vi "myRIO_BRig_RT_v0,50.vi"() -> ()   [LabVIEW 2014]
uses:
  myRIO_BRig_RT__Case_Exp_stateList.ctl
  myRIO_BRig_RT__Case_NonExp_stateList.ctl
  <vilib>/Platform/TimedLoop/XDataNode/timing_clust.ctl
  <vilib>/Platform/TimedLoop/XDataNode/nitl_modes.ctl
  <vilib>/Platform/TimedLoop/XDataNode/wakeup.ctl
  <vilib>/WebDAVClient/Advanced/SessionHandle.ctl
  <vilib>/myRIO/Common/Instrument Driver Framework/myRIO v1.0/UART/vis/myRIO v1.0 Close UART.vi
  <vilib>/FPGAPlugInAG/myRIO-1900/niLvFpga_Open_myRIO-1900.vi
  <vilib>/rvi/interface/common/dynamic/niFpgaDynamicAddResources.vi
  <vilib>/Utility/error.llb/Error Cluster From Error Code.vi
  <vilib>/rvi/errors/niLvFpgaAdjustHostInterfaceError.vi
  <vilib>/FPGAPlugInAG/Dynamic/niLvFpga_Close_Dynamic.vi
  <vilib>/myRIO/Common/Instrument Driver Framework/Utilities/vis/FPGA Ref Manager.vi
  <vilib>/myRIO/Common/Instrument Driver Framework/myRIO v1.0/myRIO v1.0 Reset FPGA.vi
  <vilib>/myRIO/Common/Instrument Driver Framework/myRIO v1.0/IRQ/vis/myRIO v1.0 IRQ Info FGV.vi
  <vilib>/myRIO/Common/Instrument Driver Framework/myRIO v1.0/IRQ/vis/myRIO v1.0 Timer IRQ Info FGV.vi
  <vilib>/myRIO/Common/Instrument Driver Framework/myRIO v1.0/IRQ/vis/myRIO v1.0 ISR Agent.vi
  <vilib>/rvi/interface/nirviOpenFPGA/nirviOpenFPGA.xnode
  myRIO_BRig_FPGA_v3,40__build.lvbitx
  myRIO_BRig_FPGA_v3,40.vi
  <vilib>/rvi/interface/nirviReadWriteControl/nirviReadWriteControl.xnode
  <vilib>/Platform/TimedLoop/XDataNode/XDataNode.xnode
  <vilib>/rvi/interface/nirviCloseFPGA/nirviCloseFPGA.xnode
  <vilib>/Platform/TimedLoop/XDataNode/XDNodeRunTimeDep.lvlib
  <vilib>/rvi/interface/Simulation/niFpgaSimulationCallBeginRW.vi
  <vilib>/myRIO/Instrument Drivers/Utilities/Utilities.lvlib
  <vilib>/WebDAVClient/NI_WebDAV.lvlib
  NiFpgaLv.dll
panel:
  in  "laser_power":dbl
  in  "f_millisec2count":dbl=109.0
  in  "laser_Tshutter":dbl=2.0
  in  "laser_Freq":dbl=10.0
  in  "laser_Tpeak":dbl=2.0
  in  "laser_duration":u16
  out "error out":errorcluster
  in  "LC_Cue1_All_Count":u16
  in  "LC_Cue1_First_Count":u16
  in  "LC_Cue1_All_delayOpt":bool
  in  "LC_ENL1_All_delayOpt":bool
  in  "LC_ENL1_All_Count":u16
  in  "LC_ENL1_First_Count":u16
  in  "LC_Cue1_First_delayOpt":bool
  in  "LC_ENL1_First_delayOpt":bool
  in  "Tcycle_Cue_max":u16=1000 caption="Max [ms]" min=5 max=5000 step=5
  in  "Tcycle_Cue_min":u16=1000 caption="Min [ms]" min=5 max=5000 step=5
  in  "SendData":bool
  out "cSpout":enum16{"Left", "Right"}(ring) caption="Left or Right Spout"
  out "A4":u32 caption="LickCounter_Right"
  out "A2":u32 caption="LickCounter_Left"
  in  "tDelay_laser_wro":u32
  in  "tCycle_laser_wro":u32=1000
  in  "tDelay_laser_rew":u32
  in  "laserResponse_wrong_LED":bool
  out "error_initTrial":errorcluster
  out "error_Selection_pre":errorcluster
  out "error_Selection":errorcluster
  in  "tCycle_laser_rew":u32=1000
  out "SelectWrong":bool
  out "SelectReward":bool
  in  "Left(F)_or_Right(T)":bool
  in  "ignoreWrong":bool
  in  "SelectionState":bool
  in  "laserResponse_wrong":bool
  in  "laserResponse_reward":bool
  in  "laserResponse_reward_LED":bool
  out "nRewards_Right":u16 caption="# Rewards Total (Right)"
  out "nRewards_Left":u16 caption="# Rewards Total (Left)"
  out "nRewards_cur":u16 caption="# Rewards in Current Block"
  out "TpB_target":u16 caption="Target Trials Per Block"
  out "cState_NonExp":T1 caption="NonExperimental State"
  out "iBlock":u16 caption="Current Block"
  out "cState":T2 caption="Experimental State"
  out "iTrial":u16 caption="Current Trial"
  in  "warmupType":bool
  in  "TestConnection":bool
  in  "warmup":bool caption="WarmUp"
  in  "Host Filename Prefix":string="Exp1_TM2"
  out "Connected To Host?":bool
  in  "Host Password":string="sabalab"
  in  "Host UserName":string="Test2"
  in  "sp_RightSpout":u16(slide)=2 max=2 step=1 scale=0.0..2.0
  in  "sp_LeftSpout":u16(slide)=2 max=2 step=1 scale=0.0..2.0
  in  "BUR_max":u16 caption="Count Reward Structure  (0 = off)"
  in  "LC_Wrong_Probability":u16
  in  "LC_Wrong_Trial":u16(slide) max=2 step=1 scale=0.0..2.0
  in  "LC_Wrong_Block":u16(slide) max=2 step=1 scale=0.0..2.0
  in  "LC_Wrong_OnOff":bool
  in  "LC_Reward_Probability":u16
  in  "LC_Reward_Trial":u16(slide) max=2 step=1 scale=0.0..2.0
  in  "LC_Reward_Block":u16(slide) max=2 step=1 scale=0.0..2.0
  in  "LC_Reward_OnOff":bool
  in  "LC_Cue1_All_Probability":u16
  in  "LC_Cue1_All_Block":u16(slide) max=2 step=1 scale=0.0..2.0
  in  "LC_Cue1_All_OnOff":bool
  in  "LC_Cue1_First_Probability":u16
  in  "LC_Cue1_First_Block":u16(slide) max=2 step=1 scale=0.0..2.0
  in  "LC_Cue1_First_OnOff":bool
  in  "LC_ENL1_All_Probability":u16 max=100 step=1
  in  "LC_ENL1_All_Block":u16(slide) max=2 step=1 scale=0.0..2.0
  in  "LC_ENL1_All_OnOff":bool
  in  "LC_ENL1_First_Probability":u16 max=100 step=1
  in  "LC_ENL1_First_Block":u16(slide) max=2 step=1 scale=0.0..2.0
  in  "Tcycle_Timeout":u16=1000 caption="Timeout Time [ms]" min=10 max=10000 step=1
  in  "Tcycle_Wrong":u16=1000 caption="Wrong Time [ms]" min=10 max=10000 step=1
  in  "Tcycle_Selection":u16=1000 caption="Answer Time [ms]" min=1 max=10000 step=1
  in  "Tcycle_RewardPost":u16=1000 caption="Consumption Time [ms]" min=250 max=10000 step=250
  in  "Tcycle_Reward_L":u16=500 caption="Reward Time [ms]" min=1 max=1000 step=1
  in  "Tcycle_Reward_R":u16=500 caption="Reward Time [ms]" min=1 max=1000 step=1
  in  "TpB_Max_R":u16=4 caption="Max TrialsPerBlock" min=1 max=12 step=1
  in  "TpB_Min_R":u16=4 caption="Min TrialsPerBlock" min=1 max=12 step=1
  in  "TpB_Max_L":u16=4 caption="Max TrialsPerBlock" min=1 max=12 step=1
  in  "TpB_Min_L":u16=4 caption="Min TrialsPerBlock" min=1 max=12 step=1
  in  "BUR_min":u16 caption="Count Reward Structure  (0 = off)"
  in  "TrialUntilReward":bool caption="Ignore Wrong \nSelection"
  in  "CueCycles":u16=1 caption="Cue Structure" min=1 max=1 step=1
  in  "MTrig_Laser_Tcycle":u16=10 caption="Time [ms]"
  in  "MTrig_Laser_trig":bool
  in  "MTrig_Audio_trig__R":bool caption="Trigger Audio"
  in  "MTrig_Audio_trig__L":bool caption="Trigger Audio"
  in  "RewCalib_Trig_R":bool caption="Calibrate_R"
  in  "RewCalib_Trig_L":bool caption="Calibrate_L"
  in  "MTrig_Solenoid_Tcycle__R":u16=300 caption="Time [ms]"
  in  "MTrig_Solenoid_Tcycle__L":u16=300 caption="Time [ms]"
  in  "MTrig_Solenoid_trig__R":bool caption="Solenoid"
  in  "MTrig_Solenoid_trig__L":bool caption="Solenoid"
  in  "STOP_abort":bool caption="Stop LabView\n(Stops myRio and FPGA)"
  in  "STOP_endBlock":bool caption="Stop Experiment\n@ End of Block"
  in  "STOP_endTrial":bool caption="Stop Experiment\n@ End of Trial"
  in  "START":bool caption="Start Experiment"
  in  "Tcycle_CuePenalty":u16=1000 caption="Penalty [ms]" min=1 max=10000 step=1
  in  "Audio_Amp__R":u16=100 caption="Amp"
  in  "Audio_Freq__R":u16=5 caption="Freq [kHz]" max=14 step=1
  in  "Audio_Amp__L":u16=100 caption="Amp"
  in  "Audio_Freq__L":u16=5 caption="Freq [kHz]" max=14 step=1
  in  "LC_Wrong_Tdelay":u16
  in  "LC_Cue1_All_Tdelay":u16
  in  "LC_ENL1_All_Tdelay":u16
  in  "LC_Reward_Tdelay":u16
  in  "LC_Cue1_First_Tdelay":u16
  in  "LC_ENL1_First_Tdelay":u16
  in  "LC_ENL1_First_OnOff":bool
  in  "Tcycle_ENLPenalty":u16=100 caption="Penalty [ms]" min=10 max=10000 step=10
  in  "Tcycle_ENL_max":u16=1000 caption="Max [ms]" min=250 max=10000 step=250
  in  "Tcycle_ENL_min":u16=1000 caption="Min [ms]" min=250 max=10000 step=250
  # "Manual Control"
  # "Task Structure"
  # "Task Timing"
  # "Laser Control\n\n                                                    On/Off      Block        Probability [%]   Delay [ms]                              Count"
  # "Manual Solenoid Trigger\nLeft              Right"
  # "Master Structure"
  # "Enforced NonLick"
  # "Enforced NonLick 1"
  # "from end"
  # "Time = Cue Min"
  # "Min\n \n  \nMax"
  # "First Trial"
  # "from start"
  # "(1) = Switching\n(2) = Two Choice"
  # "from end"
  # "All Trials"
  # "Cue"
  # "from start"
  # "Cue 1"
  # "from end"
  # "from start"
  # "Cue then reward"
  # "Min"
  # "Max"
  # "from end"
  # "Cue with reward"
  # "Trial Per Block Structure\n       Left                    Right"
  # "from start"
  # "Spout Selection Control"
  # "Manual Speaker Trigger\nLeft              Right"
  # "Selection Reward"
  # "Answer Time\n         [ms]\n\n  \nWrong Choice Penalty\n         [ms]\n \n \nChoice Timeout Penalty\n         [ms]"
  # "Selection Wrong"
  # "Cue Control"
  # "Left              Right"
  # "State"
  # "Manual Laser Trigger"
  # "Freq [kHz]\n \n \nAmp\n \n\n \n\nSpeaker\nSetting"
  # "Reward Control\n                 Left              Right"
  # "Min = 1\nMax = 32k"
  # "Reward Time\n         [ms]"
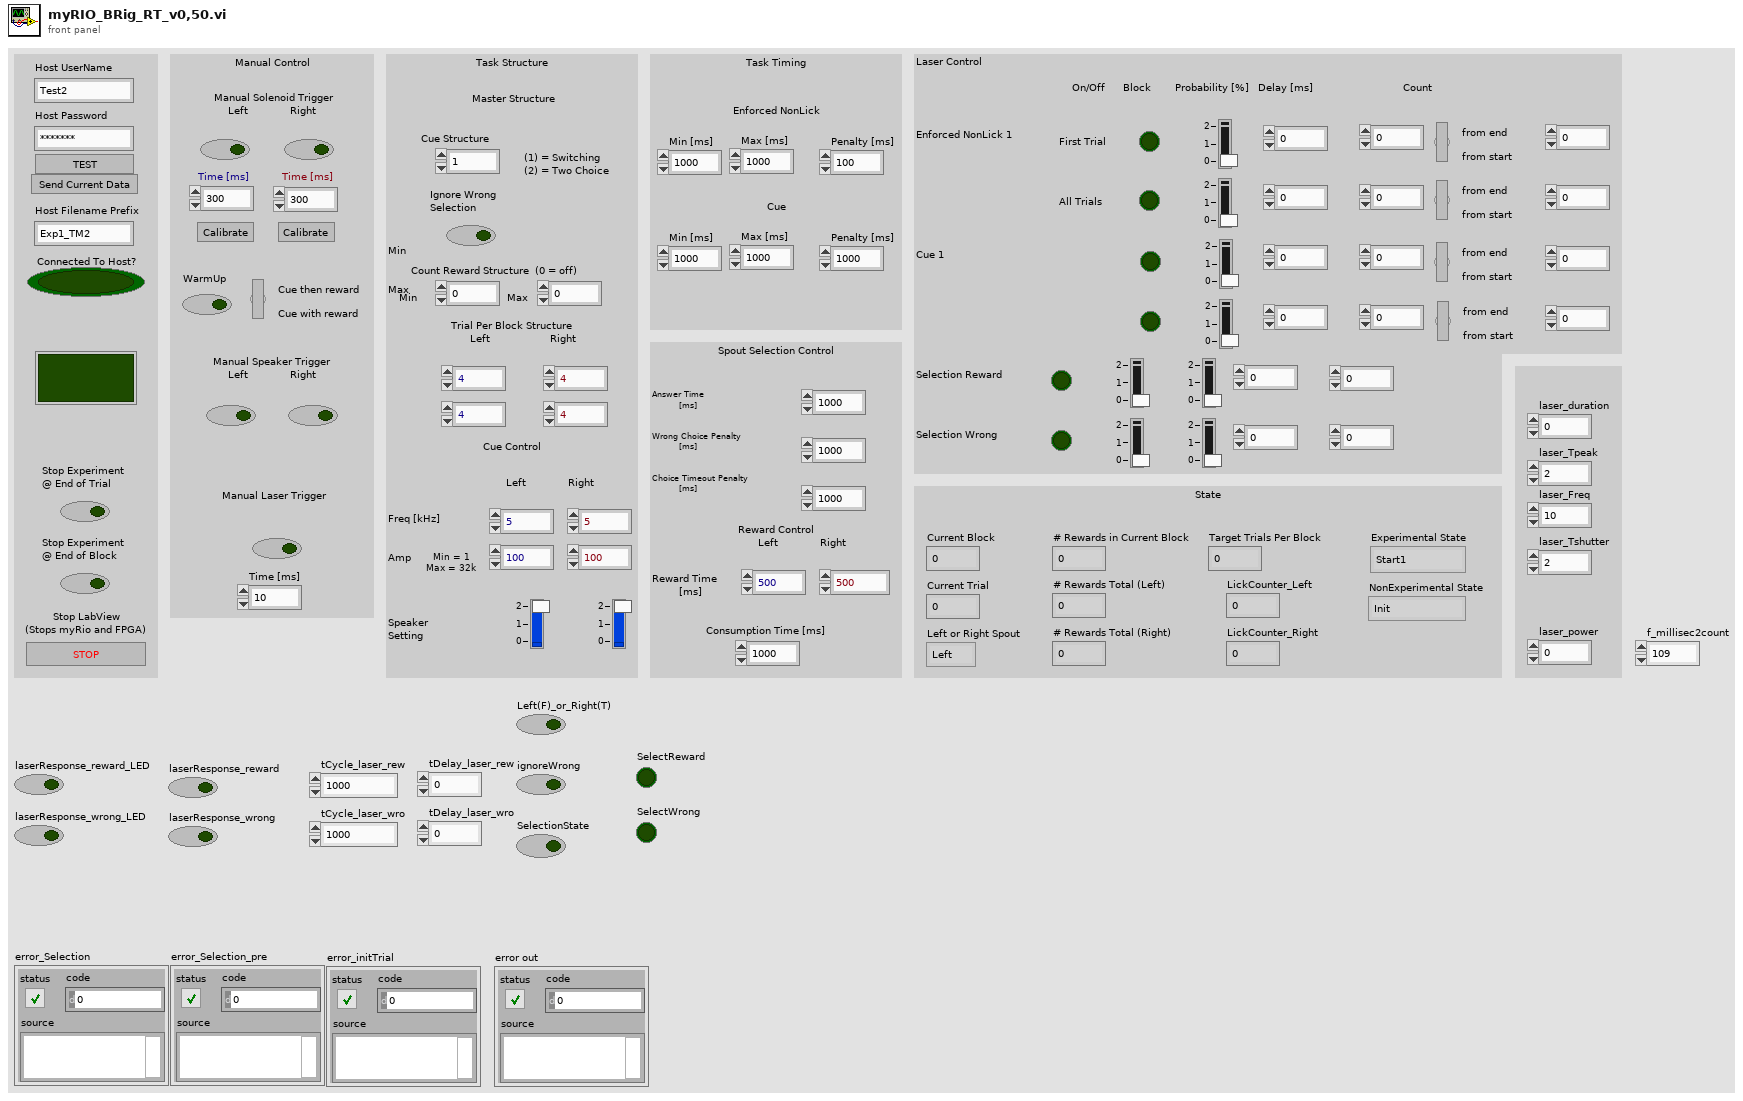
[diagram p1: front panel]
types:
  T1 = typedef "myRIO_BRig_RT__Case_NonExp_stateList.ctl" = enum16{"Init", "UploadSettings_pre", "UploadSettings_Read_dataExp", "UploadSettings_dataExp_1", "UploadSettings_Read_dataLC", "UploadSettings_dataLC_1", "UploadSettings_dataLC_2", "UploadSettings_Read_dataMTrig", "UploadSettings_dataMTrig_1", "UploadSettings_post", "Idle_pre", "IdleEmpty", "IdleEmpty2", "IdleEmpty3", "IdleEmpty4", "Idle", "Idle_2", "Idle_3", "Idle_4", "Idle_post", "Cue_pre__pre", "Cue_pre", "Cue", "Cue_post", "RewardCalibration_pre", "DispenseWater_pre__pre", "DispenseWater_pre", "DispenseWater", "DispenseWater_post", "TestConnection", "SendData", "End"}
  T2 = typedef "myRIO_BRig_RT__Case_Exp_stateList.ctl" = enum16{"Start1", "Start2", "Start3", "saveSettings1", "saveSettings2", "saveSettings3", "saveSettings4_LC_ENL", "saveSettings5_LC_Cue", "saveSettings6_LC_Other", "setSettings_Audio", "setSettings_Laser", "initBlock_pre", "initBlock", "initBlock2", "initBlock_post", "initTrial_pre", "initTrial", "initTrial2", "initTrial3", "initTrial4", "initTrial_LC_ENL1", "initTrial_LC_Cue1", "initTrial_post", "ENL1_pre", "ENL1", "ENL1_post", "ENL1Penalty_pre", "ENL1Penalty", "ENL2_pre", "ENL2", "ENL2Penalty_pre", "ENL2Penalty", "Cue1_pre", "Cue1", "Cue1_post", "Cue1Penalty_pre", "Cue1Penalty", "Cue2_pre", "Cue2", "Cue2Penalty_pre", "Cue2Penalty", "Selection_pre", "Selection", "Select_post", "SelectReward_pre", "SelectReward", "SelectRewardPost_pre", "SelectRewardPost", "SelectWrong_pre", "SelectWrong", "SelectWrong_post", "SelectTimeout_pre", "SelectTimeout", "SelectTimeout_post", "endTrial_pre", "endTrial1", "endTrial2", "endTrial3", "endTrial_post", "endBlock_pre", "endBlock", "endBlock_post", "endExp", "commConnect", "commUpload_pre", "commUpload_dataBlock", "commUpload_dataCurrent", "commUpload_dataExp", "commUpload_dataLC", "commUpload_dataTrial", "commUpload_post", "saveData_pre", "saveData_dataBlock", "saveData_dataCurrent", "saveData_dataExp", "saveData_dataLC", "saveData_dataTrial", "saveData_post", "empty_endBlock1", "empty_endBlock2", "empty_endTrial1", "empty_endTrial2", "empty_endTrial3", "empty_endTrial4", "empty_endTrial5"}
  T3 = typedef "XDNodeRunTimeDep.lvlib/timing_clust.ctl" = cluster{"Expected End [f-1]":u64, "Actual End [f-1]":u64, "Finished Late? [f-1]":bool, "Expected End [i-1]":u64, "Actual End [i-1]":u64, "Finished Late? [i-1]":bool, "Expected Start [i]":u64, "Actual Start [i]":u64, "Expected Start [f]":u64, "Actual Start [f]":u64, "Source Name":string, "Structure Name":string, "Period":i64, "Deadline":i64, "Offset":i64, "Start":i64, "Priority":i32, "Timeout":i32, "Mode":T4, "Wakeup Reason":T5, "Error":errorcluster, "Source Type":string, "Secondary Source Type":string, "Global End Time":u64, "Global Start Time":u64, "Frame Duration":u64, "Iteration Duration":u64, "Assigned CPU":i32, "I/O Scan Engine Mode":u32}
  T4 = typedef "XDNodeRunTimeDep.lvlib/nitl_modes.ctl" = enum32{"No Change", "Process missed periods, maintain original phase", "Discard missed periods, maintain original phase", "Process missed periods, ignore original phase", "Discard missed periods, ignore original phase"}
  T5 = typedef "XDNodeRunTimeDep.lvlib/wakeup.ctl" = enum32{"Normal", "Aborted", "Asynchronous wakeup", "Timing source error", "Timed loop error", "Timeout"}
  T6 = typedef "NI_WebDAV.lvlib/SessionHandle.ctl" = refnum<k1>
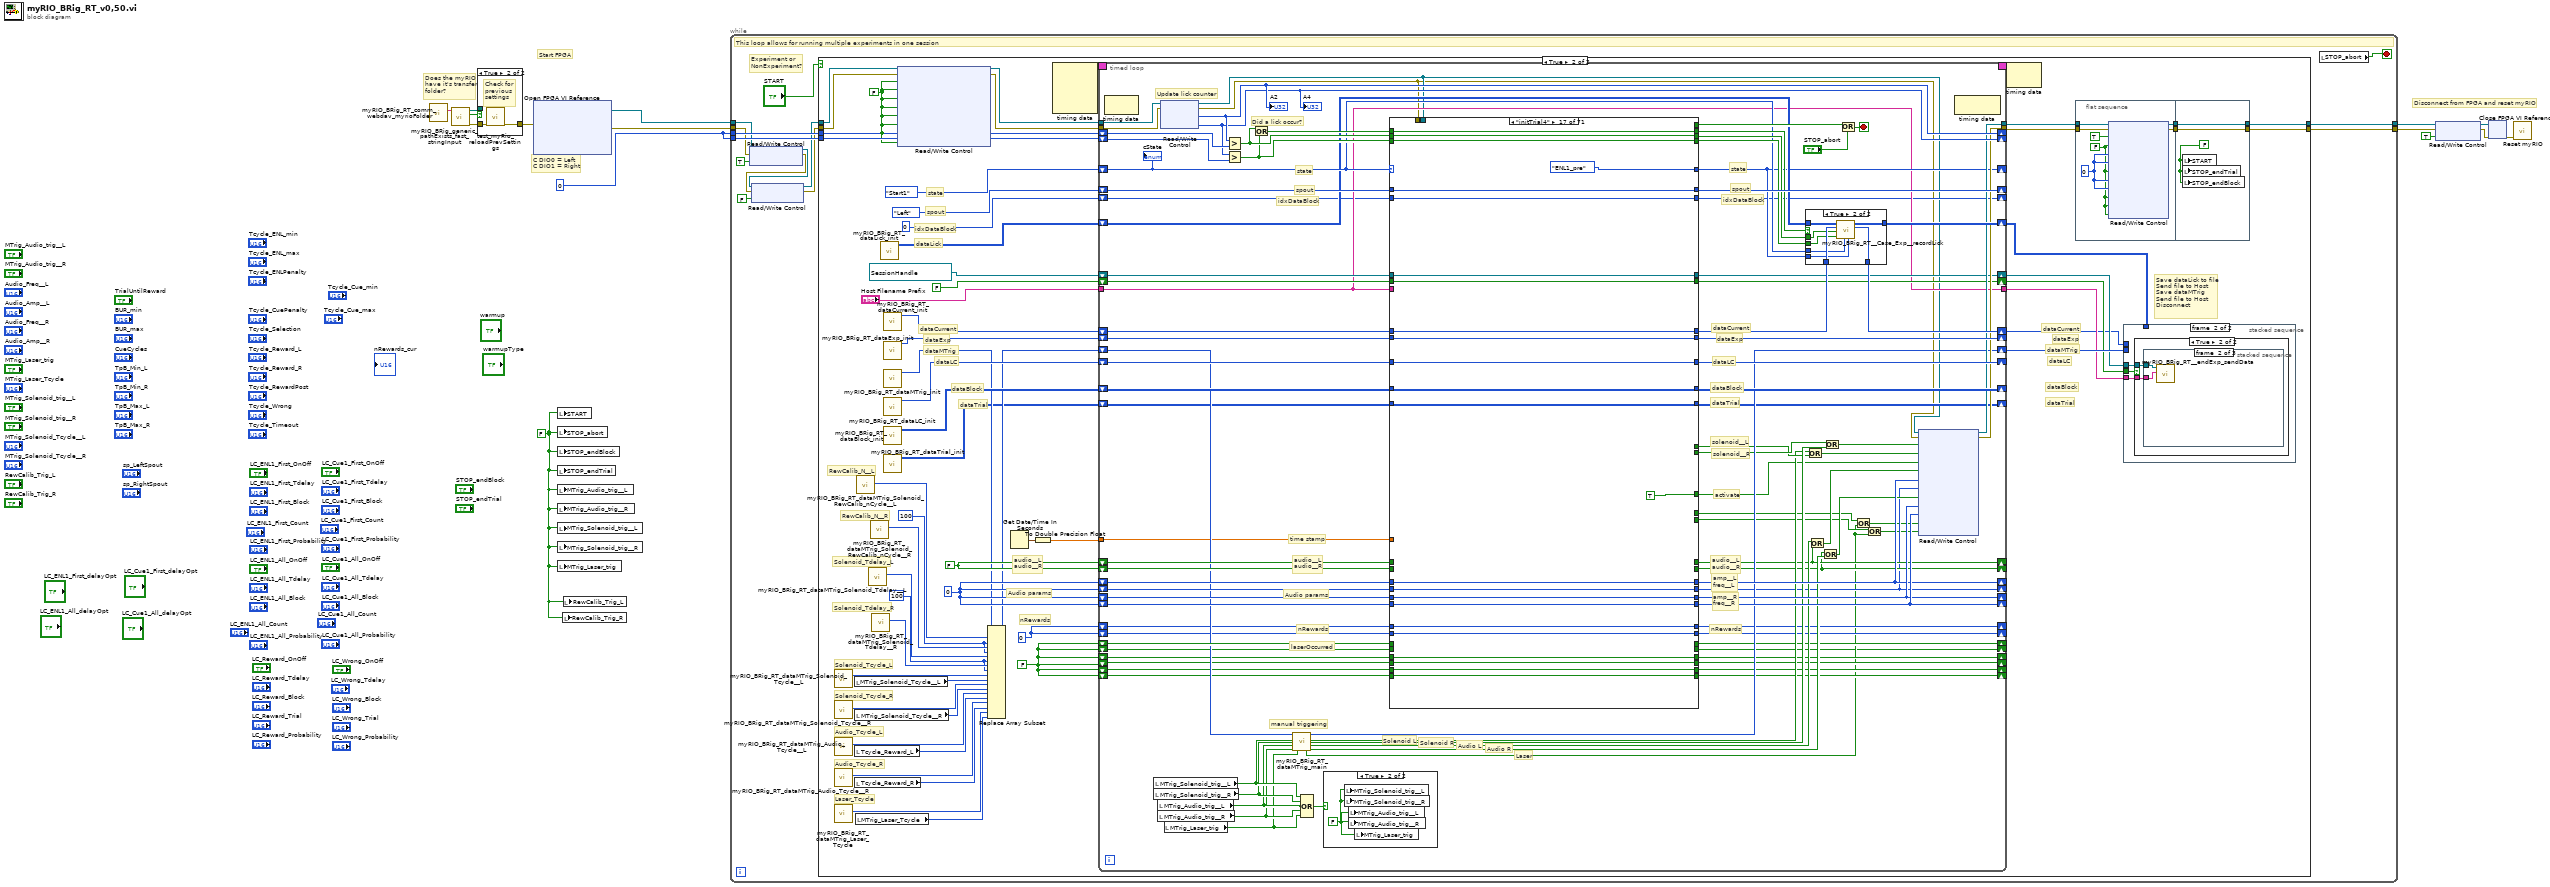
[diagram p0: block diagram]
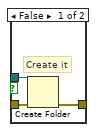
[diagram p2: hidden frame]
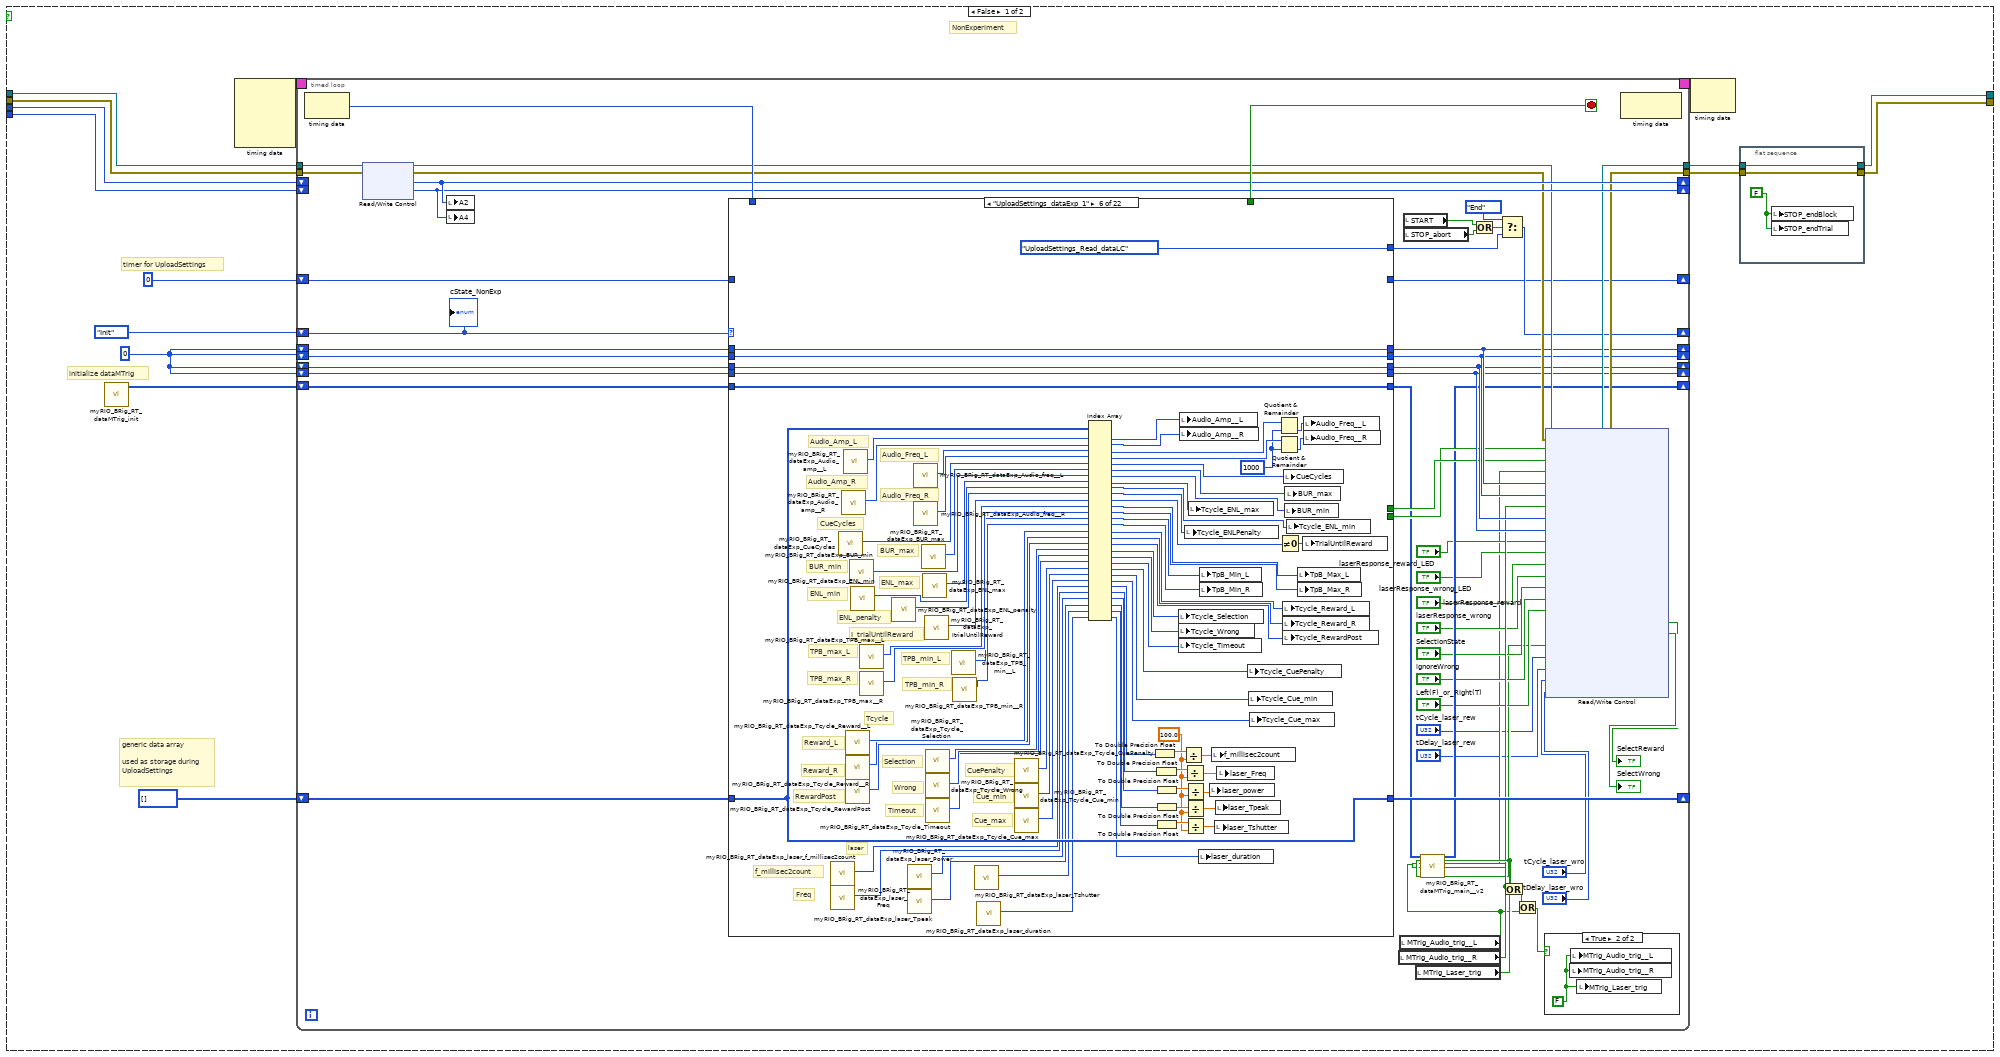
[diagram p3: hidden frame]
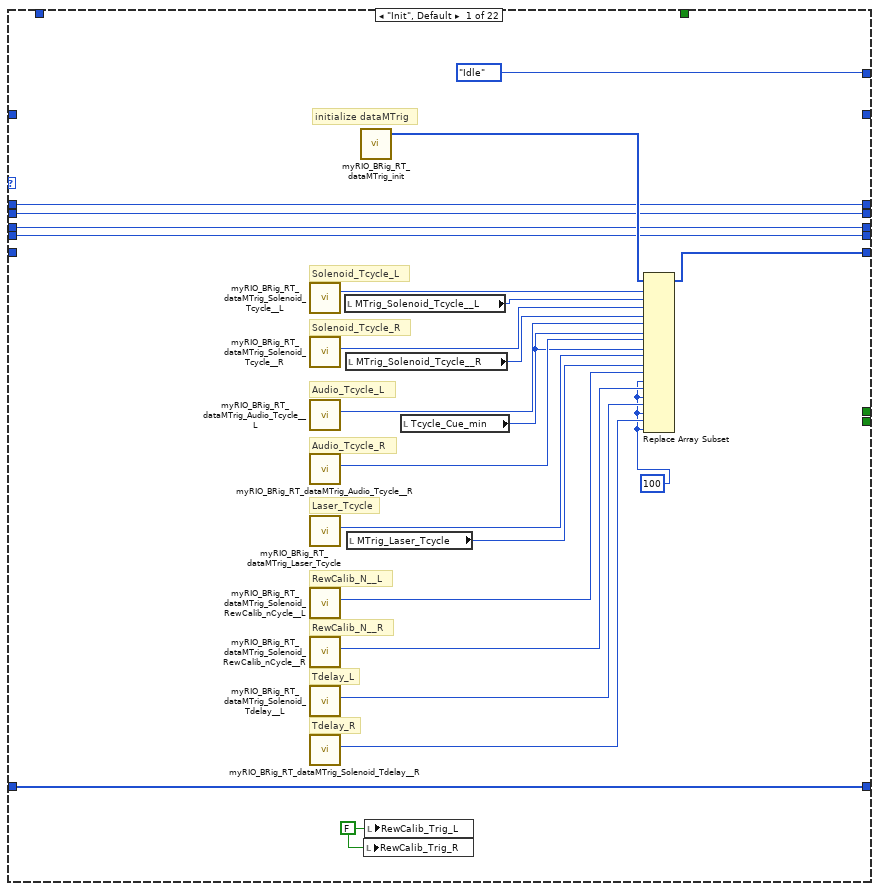
[diagram p5: hidden frame]
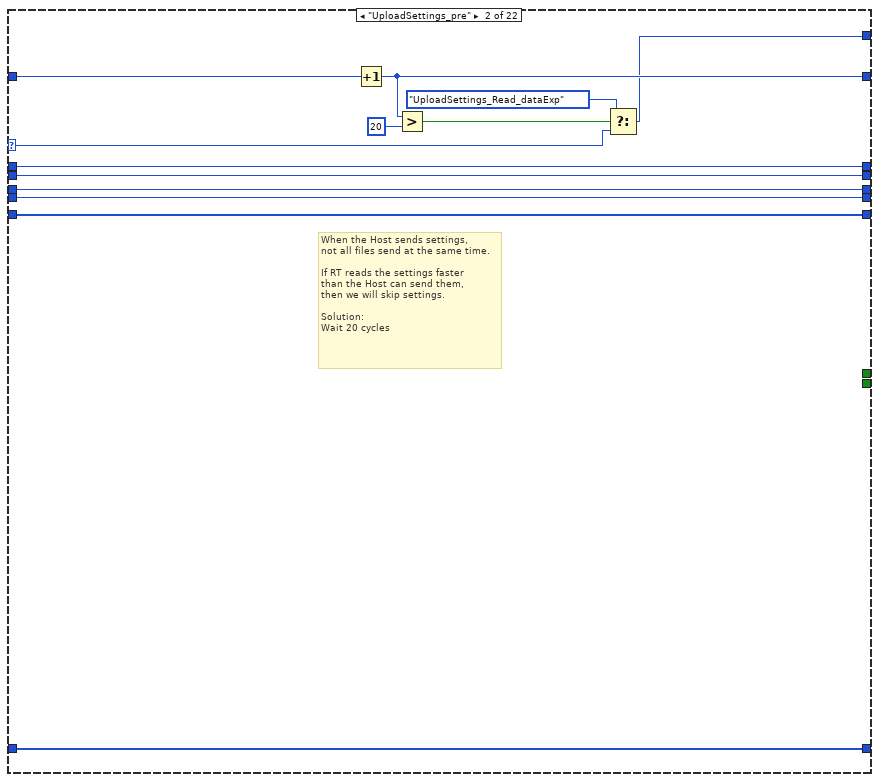
[diagram p6: hidden frame]
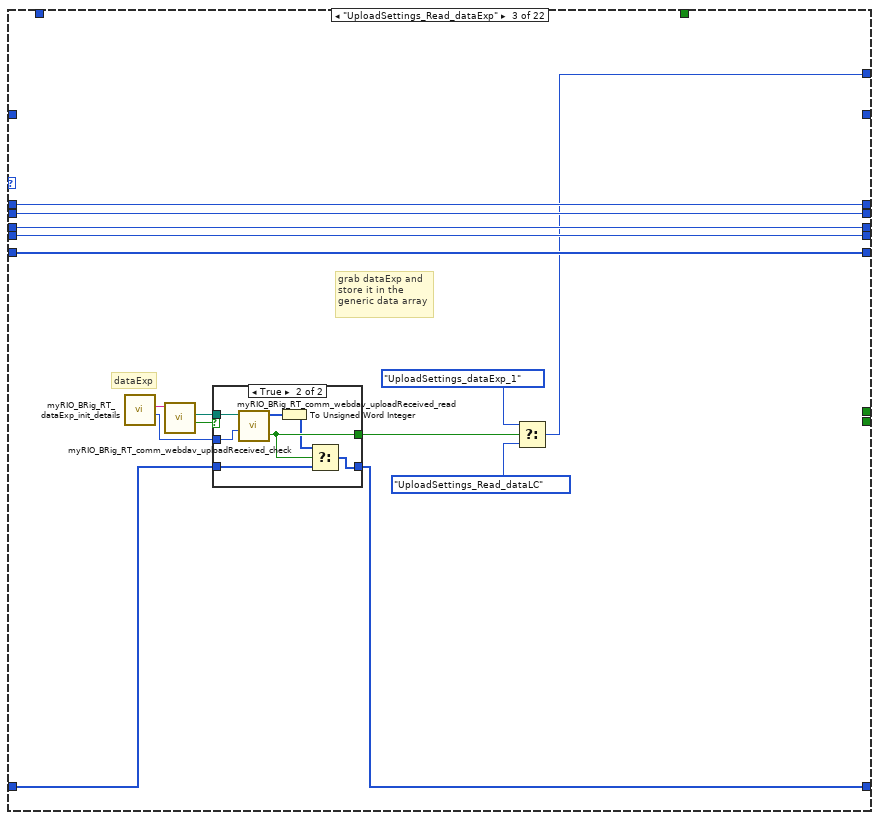
[diagram p7: hidden frame]
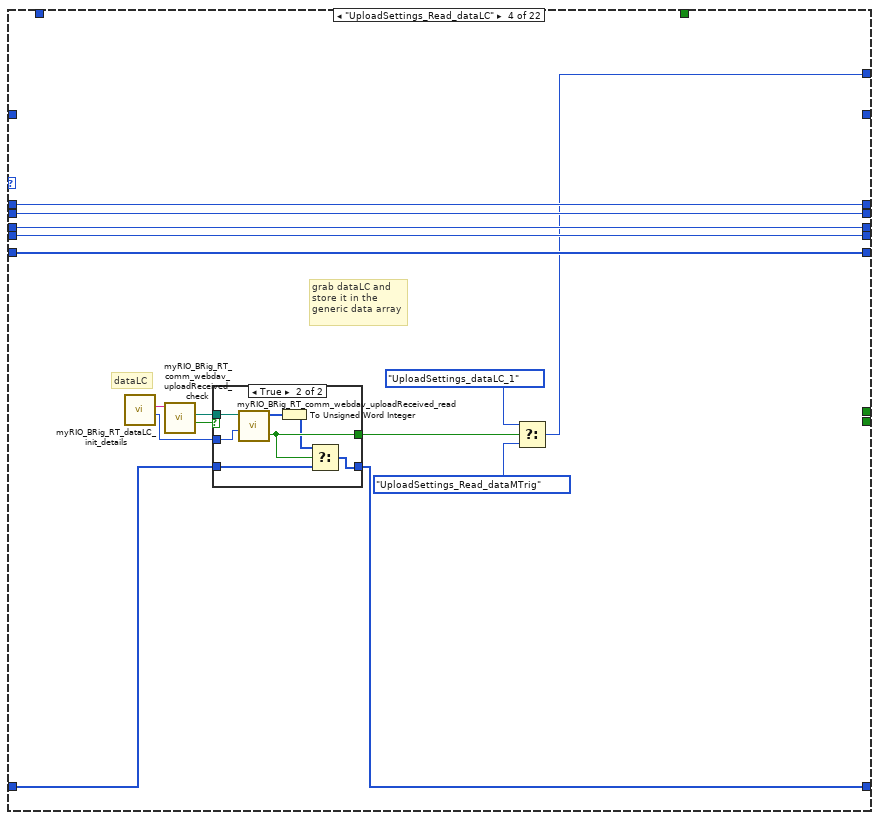
[diagram p9: hidden frame]
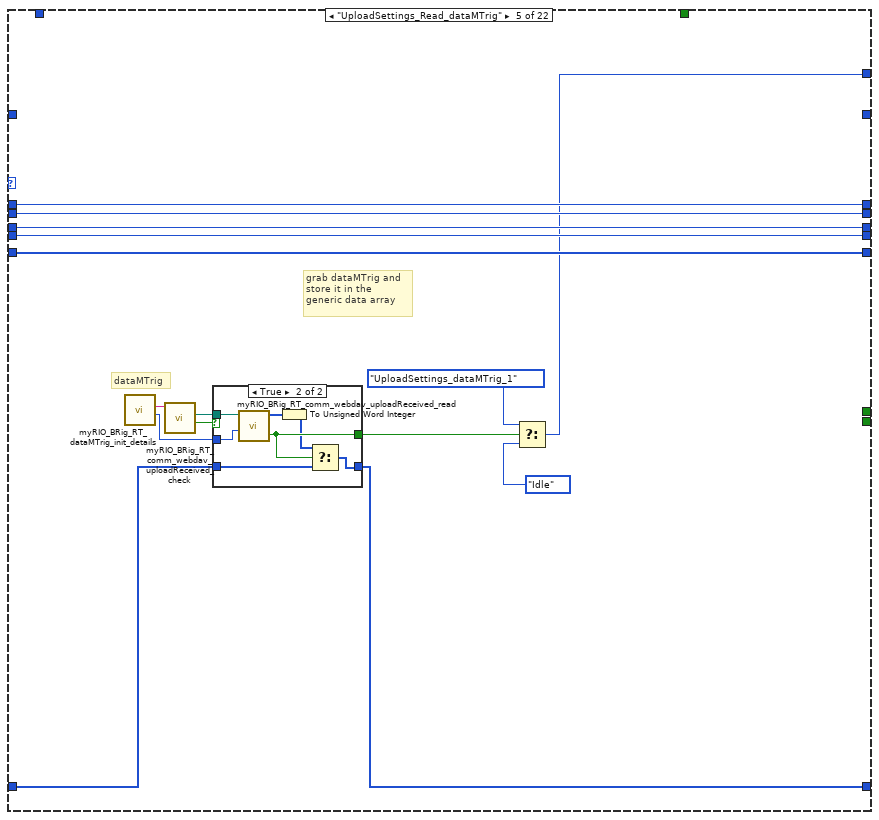
[diagram p11: hidden frame]
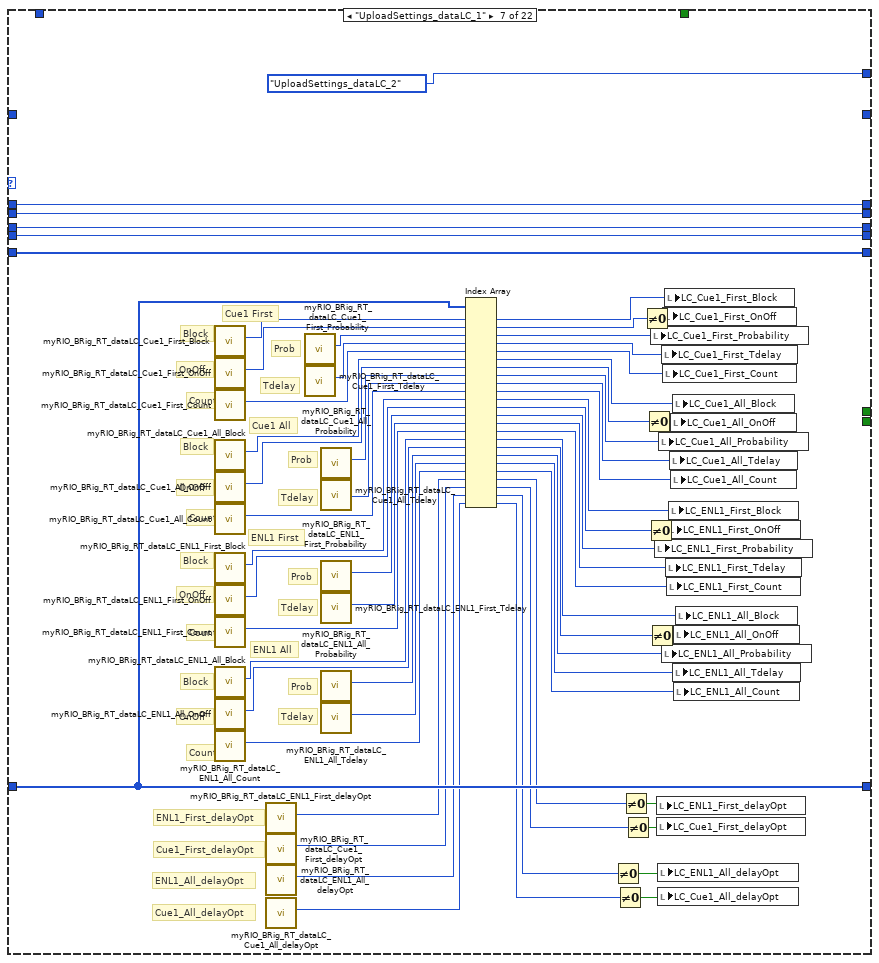
[diagram p13: hidden frame]
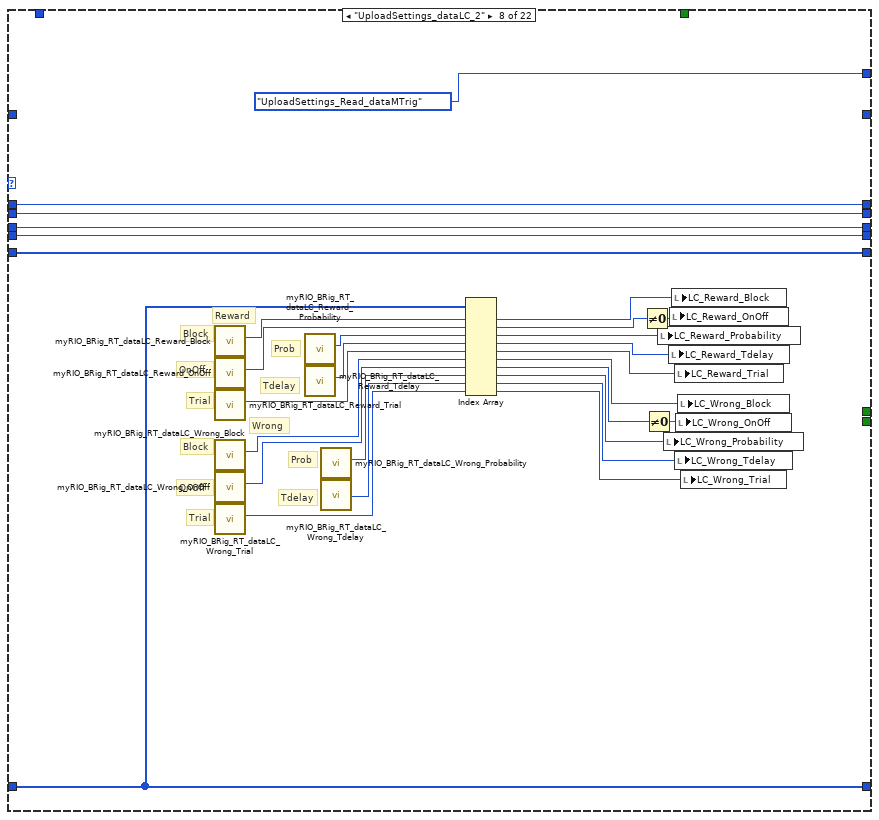
[diagram p14: hidden frame]
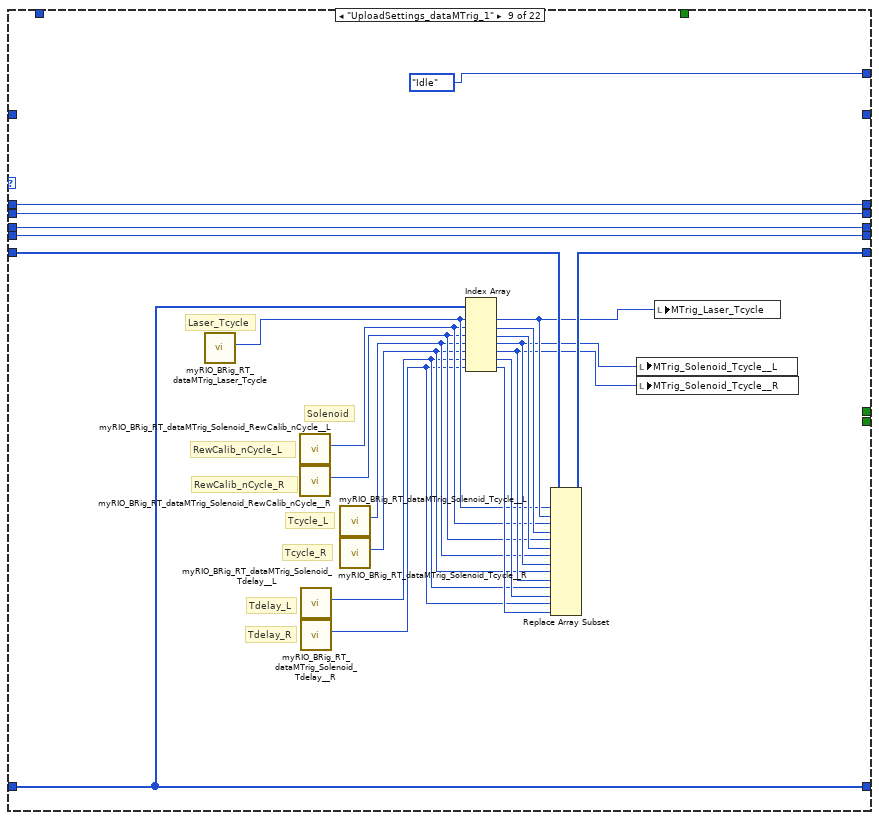
[diagram p15: hidden frame]
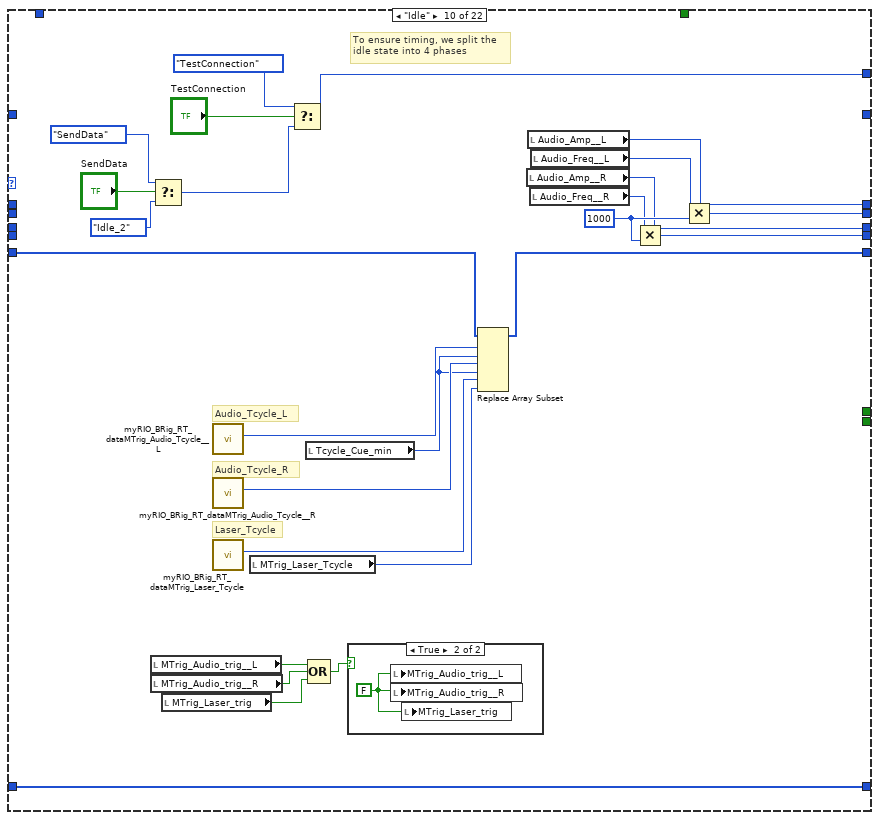
[diagram p16: hidden frame]
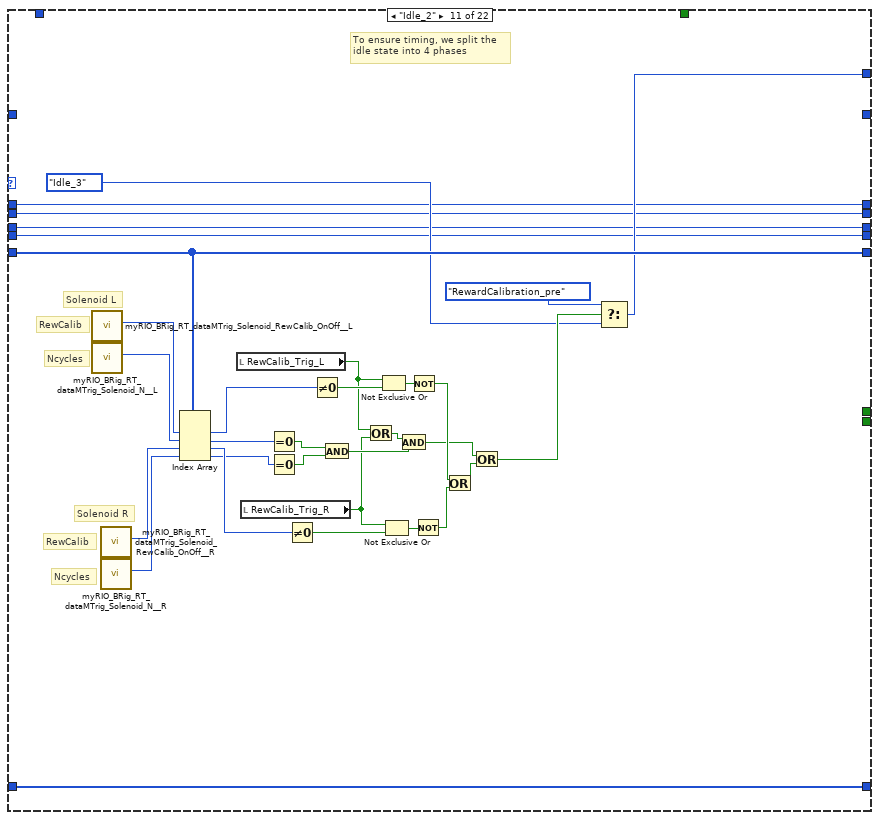
[diagram p18: hidden frame]
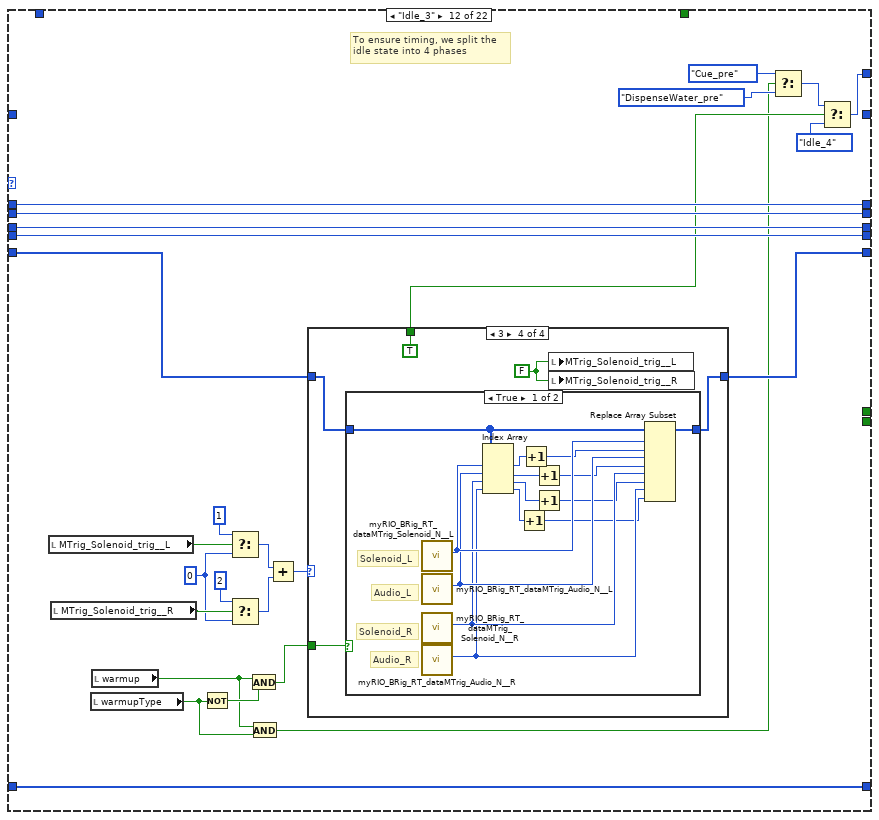
[diagram p19: hidden frame]
diagram:
  w9 = u32 0
  w6 = FALSE
  # "Does the myRIO\nhave it's transfer\nfolder?"
  # "C DIO0 = Left\nC DIO1 = Right"
  # "Start FPGA"
  # "Disconnect from FPGA and reset myRIO"
  n1 = call "myRIO_BRig_RT_comm_webdav_myrioFolder.vi"() -> ("output_myrioFolder"=w4:string)  [unwired: 11 in]
  n2 = call "myRIO_BRig_generic_pathExists_fast_stringInput.vi"("input_filePath"=w4) -> ("output_error"=w3:errorcluster, "output_Iexist"=w2:bool, "output_filePath"=w1:path)  [unwired: 8 in]
  n3 = case shown="True" w2 {
    tunnel: w1 -> [w18 _]
    tunnel: w3 -> [w17 w20]
    tunnel: [w16 w19] -> w5
    frame False {
      # "Create it"
      n4 = Create Folder(path (use dialog)=w18, error in=w17) -> (error out=w16:errorcluster)  [unwired: 1 in, 2 out]
    }
    frame True {
      # "Check for\nprevious\nsettings"
      n5 = call "test_myRio_reloadPrevSettings.vi"("input_error"=w20) -> ("output_error"=w19:errorcluster)  [unwired: 10 in]
    }
  }
  n6 = xnode "Open FPGA VI Reference"("error in"=w5) -> ("FPGA VI Reference Out"=w11:refnum<k20>, "error out"=w10:errorcluster)  [unwired: 1 in]
  n7 = local write "START"(w6) -> ()
  n8 = local write "STOP_abort"(w6) -> ()
  n9 = local write "STOP_endBlock"(w6) -> ()
  n10 = local write "STOP_endTrial"(w6) -> ()
  n11 = local write "MTrig_Audio_trig__L"(w6) -> ()
  n12 = local write "MTrig_Audio_trig__R"(w6) -> ()
  n13 = local write "MTrig_Solenoid_trig__L"(w6) -> ()
  n14 = local write "MTrig_Solenoid_trig__R"(w6) -> ()
  n15 = local write "MTrig_Laser_trig"(w6) -> ()
  n16 = local write "RewCalib_Trig_R"(w6) -> ()
  n17 = local write "RewCalib_Trig_L"(w6) -> ()
  n18 = while {
    tunnel: w11 -> [w24]
    tunnel: w10 -> [w29]
    tunnel: w9 -> [w32]
    tunnel: w9 -> [w31]
    tunnel: [w22] -> w8
    tunnel: [w21] -> w7
    stop <- w30 stop-if-true
    # "Experiment or\nNonExperiment?"
    # "This loop allows for running multiple experiments in one session"
    n19 = xnode "Read/Write Control"("FPGA VI Reference In"=w24, "error in"=w29, "Counts_Reset"=TRUE) -> ("FPGA VI Reference Out"=w26:refnum<k20>, "error out"=w27:errorcluster)
    n20 = xnode "Read/Write Control"("FPGA VI Reference In"=w26, "error in"=w27, "Counts_Reset"=FALSE) -> ("FPGA VI Reference Out"=w23:refnum<k20>, "error out"=w25:errorcluster)
    n21 = case shown="True" "START" {
      tunnel: w32 -> [w45 w936]
      tunnel: w31 -> [w44 w935]
      tunnel: w25 -> [w42 w886]
      tunnel: w23 -> [w43 w885]
      tunnel: [w40 w932] -> w22
      tunnel: [w38 w927] -> w21
      frame False {
        w37 = u16 0 ("Audio_Amp__L")
        # "generic data array\n\nused as storage during\nUploadSettings"
        # "timer for UploadSettings"
        # "initialize dataMTrig"
        # "NonExperiment"
        n22 = call "myRIO_BRig_RT_dataMTrig_init.vi"() -> ("output_dataMTrig"=w46:u16[])  [unwired: 5 in]
        n23 = node-c288() -> (w49:T3)  [unwired: 4 in]
        n24 = timed-loop {
          timing: w49 -> [_]
          timing-out: [_] -> w48
          shift-right: [w82] -> _
          shift-left: w46 -> [w106]
          shift-right: [w71] -> _
          shift-left: myRIO_BRig_RT__Case_NonExp_stateList."Init" ("Enum") -> [w96]
          shift-right: [w104] -> _
          shift-left: w45 -> [_]
          shift-right: [w103] -> _
          shift-left: w44 -> [_]
          tunnel: [w99] -> w41
          tunnel: [w97] -> w39
          tunnel: w42 -> [w102]
          tunnel: w43 -> [w101]
          shift-right: [w95] -> _
          shift-left: u16[] [] ("output_data") -> [w94]
          shift-right: [w89] -> _
          shift-left: w37 -> [w93]
          shift-right: [w88] -> _
          shift-left: w37 -> [w92]
          shift-right: [w87] -> _
          shift-left: w37 -> [w91]
          shift-right: [w86] -> _
          shift-left: w37 -> [w90]
          shift-right: [w53] -> _
          shift-left: u16 0 ("Audio_Amp__L") -> [w54]
          stop <- w107 stop-if-true
          n25 = node-c288() -> (w105:i64)  [unwired: 1 in]
          n26 = xnode "Read/Write Control"("FPGA VI Reference In"=w101, "error in"=w102) -> ("FPGA VI Reference Out"=w100:refnum<k20>, "error out"=w98:errorcluster, "A2_LickL"=w104:u32, "A4_LickR"=w103:u32)
          n27 = local write "A2"(w104) -> ()
          n28 = local write "A4"(w103) -> ()
          n29 = case shown="\"UploadSettings_dataExp_1\"" w96 {
            selector: w96 -> [_ w140 _ _ _ _ _ _ _ _ _ _ _ _ w595 _ _ w780 _ _ _ w877]
            tunnel: [myRIO_BRig_RT__Case_NonExp_stateList."Idle" ("Enum") w138 w145 w168 w191 myRIO_BRig_RT__Case_NonExp_stateList."UploadSettings_Read_dataLC" ("Enum") myRIO_BRig_RT__Case_NonExp_stateList."UploadSettings_dataLC_2" ("Enum") myRIO_BRig_RT__Case_NonExp_stateList."UploadSettings_Read_dataMTrig" ("f") myRIO_BRig_RT__Case_NonExp_stateList."Idle" ("Enum") w421 w442 w475 w566 myRIO_BRig_RT__Case_NonExp_stateList."Cue" ("t") w594 myRIO_BRig_RT__Case_NonExp_stateList."DispenseWater_pre" ("Enum") w722 w778 w805 myRIO_BRig_RT__Case_NonExp_stateList."Idle" ("Enum") myRIO_BRig_RT__Case_NonExp_stateList."Idle" ("Enum") w877] -> w72
            tunnel: [w123 w133 w155 w178 w201 w295 w358 w387 w407 w432 w457 w486 w564 w582 w608 w632 w759 w785 w816 w859 w869 w875] -> w83
            tunnel: [_ _ _ _ _ _ _ _ _ _ _ _ _ _ _ _ _ _ _ _ _ TRUE] -> w107
            tunnel: w106 -> [_ w133 w155 w178 w201 w295 w358 w387 w408 w431 w457 w487 w564 w583 w608 w618 w755 w786 w817 w859 w869 w875]
            tunnel: w105 -> [_ _ _ _ _ _ _ _ _ _ _ _ _ _ _ _ _ w790 _ _ _ _]
            tunnel: [w112 w132 w146 w169 w192 w239 w310 w359 w388 w416 w437 w469 w559 w570 w593 w609 w707 w763 w798 w847 w863 w870] -> w95
            tunnel: w94 -> [w112 w132 w147 w170 w193 w239 w310 w359 w388 w416 w437 w469 w559 w570 w593 w609 w707 w763 w798 w847 w863 w870]
            tunnel: [w116 w136 w158 w181 w204 w292 w356 w362 w405 w427 w440 w479 w561 w590 w605 w612 w761 w796 w823 w850 w866 w873] -> w88
            tunnel: [w114 w134 w156 w179 w202 w290 w354 w360 w403 w426 w438 w481 w563 w588 w607 w610 w760 w794 w821 w848 w864 w871] -> w86
            tunnel: [w117 w137 w159 w182 w205 w293 w357 w363 w406 w425 w441 w478 w560 w592 w604 w613 w762 w797 w824 w851 w867 w874] -> w89
            tunnel: [w115 w135 w157 w180 w203 w291 w355 w361 w404 w424 w439 w480 w562 w589 w606 w611 w760 w795 w822 w849 w865 w872] -> w87
            tunnel: w93 -> [w117 w137 w159 w182 w205 w293 w357 w363 w406 _ w441 w478 w560 w592 w604 w613 w762 w797 w824 w851 w867 w874]
            tunnel: w92 -> [w116 w136 w158 w181 w204 w292 w356 w362 w405 _ w440 w479 w561 w590 w605 w612 w761 w796 w823 w850 w866 w873]
            tunnel: w91 -> [w115 w135 w157 w180 w203 w291 w355 w361 w404 _ w439 w480 w562 w589 w606 w611 w760 w795 w822 w849 w865 w872]
            tunnel: w90 -> [w114 w134 w156 w179 w202 w290 w354 w360 w403 _ w438 w481 w563 w588 w607 w610 _ w794 w821 w848 w864 w871]
            tunnel: [_ _ _ _ _ _ _ _ _ _ _ _ _ _ _ _ _ w787 _ _ _ _] -> w85
            tunnel: [_ _ _ _ _ _ _ _ _ _ _ _ _ _ _ _ _ w769 _ _ _ _] -> w84
            tunnel: w54 -> [_ w144 _ _ _ _ _ _ _ _ _ _ _ _ _ _ _ _ _ _ _ _]
            tunnel: [_ w143 _ _ _ _ _ _ _ _ _ _ _ _ _ _ _ _ _ _ _ _] -> w53
            frame "Init", Default {
              w113 = FALSE ("RewCalib_Trig_L")
              w109 = u16 100 ("new element/subarray")
              # "Tdelay_R"
              # "Tdelay_L"
              # "RewCalib_N__R"
              # "RewCalib_N__L"
              # "Solenoid_Tcycle_R"
              # "Solenoid_Tcycle_L"
              # "Laser_Tcycle"
              # "Audio_Tcycle_R"
              # "Audio_Tcycle_L"
              # "initialize dataMTrig"
              n30 = call "myRIO_BRig_RT_dataMTrig_Solenoid_Tcycle__L.vi"() -> ("output_Solenoid_Tcycle__L"=w125:i32)  [unwired: 11 in]
              n31 = call "myRIO_BRig_RT_dataMTrig_Solenoid_Tcycle__R.vi"() -> ("output_Solenoid_Tcycle__R"=w126:i32)  [unwired: 11 in]
              n32 = call "myRIO_BRig_RT_dataMTrig_Audio_Tcycle__L.vi"() -> ("output_Audio_Tcycle__L"=w127:i32)  [unwired: 11 in]
              n33 = call "myRIO_BRig_RT_dataMTrig_Audio_Tcycle__R.vi"() -> ("output_Audio_Tcycle__R"=w128:i32)  [unwired: 11 in]
              n34 = call "myRIO_BRig_RT_dataMTrig_Laser_Tcycle.vi"() -> ("output_Laser_Tcycle"=w129:i32)  [unwired: 11 in]
              n35 = call "myRIO_BRig_RT_dataMTrig_Solenoid_RewCalib_nCycle__L.vi"() -> ("output_Solenoid_RewCalib_nCycle__L"=w121:i32)  [unwired: 11 in]
              n36 = call "myRIO_BRig_RT_dataMTrig_Solenoid_RewCalib_nCycle__R.vi"() -> ("output_Solenoid_RewCalib_nCycle__R"=w120:i32)  [unwired: 11 in]
              n37 = call "myRIO_BRig_RT_dataMTrig_Solenoid_Tdelay__L.vi"() -> ("output_Solenoid_Tdelay__L"=w119:i32)  [unwired: 11 in]
              n38 = call "myRIO_BRig_RT_dataMTrig_Solenoid_Tdelay__R.vi"() -> ("output_Solenoid_Tdelay__R"=w118:i32)  [unwired: 11 in]
              n39 = local read "MTrig_Solenoid_Tcycle__L"() -> (w130:u16)
              n40 = local read "MTrig_Solenoid_Tcycle__R"() -> (w131:u16)
              n41 = local read "MTrig_Laser_Tcycle"() -> (w110:u16)
              n42 = call "myRIO_BRig_RT_dataMTrig_init.vi"() -> ("output_dataMTrig"=w124:u16[])  [unwired: 5 in]
              n43 = local write "RewCalib_Trig_R"(w113) -> ()
              n44 = local write "RewCalib_Trig_L"(w113) -> ()
              n45 = local read "Tcycle_Cue_min"() -> (w111:u16)
              n46 = Replace Array Subset(array=w124, new element #1=w130, index #1=w125, new element #2=w131, index #2=w126, new element #3=w111, index #3=w127, new element #4=w111, index #4=w128, new element #5=w110, index #5=w129, new element #6=w109, index #6=w121, new element #7=w109, index #7=w120, new element #8=w109, index #8=w119, new element #9=w109, index #9=w118) -> (w123:u16[])
            }
            frame "UploadSettings_pre" {
              # "When the Host sends settings,\nnot all files send at the same time.\n\nIf RT reads the settings faster\nthan the Host can send them,\nthen we will skip settings.\n\nSolution:\nWait 20 cycles"
              n47 = Increment(x=w144) -> (x+1=w143:u16)
              n48 = Greater?(x=w143, y=u16 20) -> (0:w141:bool)
              n49 = Select(t=myRIO_BRig_RT__Case_NonExp_stateList."UploadSettings_Read_dataExp", s=w141, f=w140) -> (s? t:f=w138:T1)
            }
            frame "UploadSettings_Read_dataExp" {
              # "grab dataExp and\nstore it in the\ngeneric data array"
              # "dataExp"
              n50 = call "myRIO_BRig_RT_dataExp_init_details.vi"() -> ("output_dataSize"=w151:i32, "output_dataName"=w154:string)  [unwired: 10 in]
              n51 = call "myRIO_BRig_RT_comm_webdav_uploadReceived_check.vi"("input_dataName"=w154) -> ("output_Iexist"=w153:bool, "output_dataPath"=w152:path)  [unwired: 9 in]
              n52 = case shown="True" w153 {
                tunnel: w152 -> [_ w167]
                tunnel: w151 -> [_ w166]
                tunnel: [_ w165] -> w150
                tunnel: w147 -> [w160 w164]
                tunnel: [w160 w161] -> w146
                frame False {
                }
                frame True {
                  n53 = call "myRIO_BRig_RT_comm_webdav_uploadReceived_read.vi"("input_dataSize"=w166, "input_filePath"=w167) -> ("output_Ivalid"=w165:bool, "output_data"=w163:i64[])  [unwired: 8 in]
                  n54 = To Unsigned Word Integer(number=w163) -> (unsigned 16bit integer=w162:u16[])
                  n55 = Select(t=w162, s=w165, f=w164) -> (s? t:f=w161:u16[])
                }
              }
              n56 = Select(t=myRIO_BRig_RT__Case_NonExp_stateList."UploadSettings_dataExp_1", s=w150, f=myRIO_BRig_RT__Case_NonExp_stateList."UploadSettings_Read_dataLC" ("t")) -> (s? t:f=w145:T1)
            }
            frame "UploadSettings_Read_dataLC" {
              # "grab dataLC and\nstore it in the\ngeneric data array"
              # "dataLC"
              n57 = call "myRIO_BRig_RT_dataLC_init_details.vi"() -> ("output_dataSize"=w174:i32, "output_dataName"=w177:string)  [unwired: 10 in]
              n58 = call "myRIO_BRig_RT_comm_webdav_uploadReceived_check.vi"("input_dataName"=w177) -> ("output_Iexist"=w176:bool, "output_dataPath"=w175:path)  [unwired: 9 in]
              n59 = case shown="True" w176 {
                tunnel: w175 -> [_ w190]
                tunnel: w174 -> [_ w189]
                tunnel: [_ w188] -> w173
                tunnel: w170 -> [w183 w187]
                tunnel: [w183 w184] -> w169
                frame False {
                }
                frame True {
                  n60 = call "myRIO_BRig_RT_comm_webdav_uploadReceived_read.vi"("input_dataSize"=w189, "input_filePath"=w190) -> ("output_Ivalid"=w188:bool, "output_data"=w186:i64[])  [unwired: 8 in]
                  n61 = To Unsigned Word Integer(number=w186) -> (unsigned 16bit integer=w185:u16[])
                  n62 = Select(t=w185, s=w188, f=w187) -> (s? t:f=w184:u16[])
                }
              }
              n63 = Select(t=myRIO_BRig_RT__Case_NonExp_stateList."UploadSettings_dataLC_1", s=w173, f=myRIO_BRig_RT__Case_NonExp_stateList."UploadSettings_Read_dataMTrig" ("t")) -> (s? t:f=w168:T1)
            }
            frame "UploadSettings_Read_dataMTrig" {
              # "grab dataMTrig and\nstore it in the\ngeneric data array"
              # "dataMTrig"
              n64 = call "myRIO_BRig_RT_dataMTrig_init_details.vi"() -> ("output_dataSize"=w197:i32, "output_dataName"=w200:string)  [unwired: 10 in]
              n65 = call "myRIO_BRig_RT_comm_webdav_uploadReceived_check.vi"("input_dataName"=w200) -> ("output_Iexist"=w199:bool, "output_dataPath"=w198:path)  [unwired: 9 in]
              n66 = case shown="True" w199 {
                tunnel: w198 -> [_ w213]
                tunnel: w197 -> [_ w212]
                tunnel: [_ w211] -> w196
                tunnel: w193 -> [w206 w210]
                tunnel: [w206 w207] -> w192
                frame False {
                }
                frame True {
                  n67 = call "myRIO_BRig_RT_comm_webdav_uploadReceived_read.vi"("input_dataSize"=w212, "input_filePath"=w213) -> ("output_Ivalid"=w211:bool, "output_data"=w209:i64[])  [unwired: 8 in]
                  n68 = To Unsigned Word Integer(number=w209) -> (unsigned 16bit integer=w208:u16[])
                  n69 = Select(t=w208, s=w211, f=w210) -> (s? t:f=w207:u16[])
                }
              }
              n70 = Select(t=myRIO_BRig_RT__Case_NonExp_stateList."UploadSettings_dataMTrig_1", s=w196, f=myRIO_BRig_RT__Case_NonExp_stateList."Idle" ("t")) -> (s? t:f=w191:T1)
            }
            frame "UploadSettings_dataExp_1" {
              w222 = 100.0 ("y")
              w240 = u16 1000 ("y")
              # "Freq"
              # "f_millisec2count"
              # "laser"
              # "Cue_max"
              # "Cue_min"
              # "CuePenalty"
              # "Timeout"
              # "Wrong"
              # "Selection"
              # "RewardPost"
              # "Reward_R"
              # "Reward_L"
              # "Tcycle"
              # "TPB_min_R"
              # "TPB_min_L"
              # "TPB_max_R"
              # "TPB_max_L"
              # "I_trialUntilReward"
              # "ENL_penalty"
              # "ENL_min"
              # "ENL_max"
              # "BUR_max"
              # "BUR_min"
              # "CueCycles"
              # "Audio_Freq_R"
              # "Audio_Freq_L"
              # "Audio_Amp_R"
              # "Audio_Amp_L"
              n71 = call "myRIO_BRig_RT_dataExp_laser_f_millisec2count.vi"() -> ("output_laser_f_millisec2count"=w236:i32)  [unwired: 11 in]
              n72 = call "myRIO_BRig_RT_dataExp_laser_Freq.vi"() -> ("output_laser_Freq"=w235:i32)  [unwired: 11 in]
              n73 = call "myRIO_BRig_RT_dataExp_CueCycles.vi"() -> ("output_CueCycles"=w283:i32)  [unwired: 11 in]
              n74 = call "myRIO_BRig_RT_dataExp_Audio_amp__R.vi"() -> ("output_Audio_amp__R"=w287:i32)  [unwired: 11 in]
              n75 = call "myRIO_BRig_RT_dataExp_Audio_amp__L.vi"() -> ("output_Audio_amp__L"=w289:i32)  [unwired: 11 in]
              n76 = call "myRIO_BRig_RT_dataExp_Tcycle_Reward__L.vi"() -> ("output_Tcycle_Reward__L"=w260:i32)  [unwired: 11 in]
              n77 = call "myRIO_BRig_RT_dataExp_Tcycle_Reward__R.vi"() -> ("output_Tcycle_Reward__R"=w259:i32)  [unwired: 11 in]
              n78 = call "myRIO_BRig_RT_dataExp_Tcycle_RewardPost.vi"() -> ("output_Tcycle_RewardPost"=w258:i32)  [unwired: 11 in]
              n79 = call "myRIO_BRig_RT_dataExp_BUR_min.vi"() -> ("output_BUR_min"=w280:i32)  [unwired: 11 in]
              n80 = call "myRIO_BRig_RT_dataExp_ENL_min.vi"() -> ("output_ENL_min"=w276:i32)  [unwired: 11 in]
              n81 = call "myRIO_BRig_RT_dataExp_TPB_max__L.vi"() -> ("output_TPB_max__L"=w268:i32)  [unwired: 11 in]
              n82 = call "myRIO_BRig_RT_dataExp_TPB_max__R.vi"() -> ("output_TPB_max__R"=w267:i32)  [unwired: 11 in]
              n83 = call "myRIO_BRig_RT_dataExp_ENL_penalty.vi"() -> ("output_ENL_penalty"=w275:i32)  [unwired: 11 in]
              n84 = call "myRIO_BRig_RT_dataExp_laser_Power.vi"() -> ("output_laser_Power"=w234:i32)  [unwired: 11 in]
              n85 = call "myRIO_BRig_RT_dataExp_laser_Tpeak.vi"() -> ("output_laser_Tpeak"=w233:i32)  [unwired: 11 in]
              n86 = call "myRIO_BRig_RT_dataExp_Audio_freq__L.vi"() -> ("output_Audio_freq__L"=w285:i32)  [unwired: 11 in]
              n87 = call "myRIO_BRig_RT_dataExp_Audio_freq__R.vi"() -> ("output_Audio_freq__R"=w284:i32)  [unwired: 11 in]
              n88 = call "myRIO_BRig_RT_dataExp_BUR_max.vi"() -> ("output_BUR_max"=w281:i32)  [unwired: 11 in]
              n89 = call "myRIO_BRig_RT_dataExp_ENL_max.vi"() -> ("output_ENL_max"=w277:i32)  [unwired: 11 in]
              n90 = call "myRIO_BRig_RT_dataExp_ItrialUntilReward.vi"() -> ("output_I_trialUntilReward"=w271:i32)  [unwired: 11 in]
              n91 = call "myRIO_BRig_RT_dataExp_Tcycle_Selection.vi"() -> ("output_Tcycle_Selection"=w257:i32)  [unwired: 11 in]
              n92 = call "myRIO_BRig_RT_dataExp_Tcycle_Wrong.vi"() -> ("output_Tcycle_Wrong"=w256:i32)  [unwired: 11 in]
              n93 = call "myRIO_BRig_RT_dataExp_Tcycle_Timeout.vi"() -> ("output_Tcycle_Timeout"=w255:i32)  [unwired: 11 in]
              n94 = call "myRIO_BRig_RT_dataExp_TPB_min__L.vi"() -> ("output_TPB_min__L"=w266:i32)  [unwired: 11 in]
              n95 = call "myRIO_BRig_RT_dataExp_TPB_min__R.vi"() -> ("output_TPB_min__R"=w265:i32)  [unwired: 11 in]
              n96 = call "myRIO_BRig_RT_dataExp_laser_Tshutter.vi"() -> ("output_laser_Tshutter"=w232:i32)  [unwired: 11 in]
              n97 = call "myRIO_BRig_RT_dataExp_laser_duration.vi"() -> ("output_laser_duration"=w231:i32)  [unwired: 11 in]
              n98 = call "myRIO_BRig_RT_dataExp_Tcycle_CuePenalty.vi"() -> ("output_Tcycle_CuePenalty"=w248:i32)  [unwired: 11 in]
              n99 = call "myRIO_BRig_RT_dataExp_Tcycle_Cue_min.vi"() -> ("output_Tcycle_Cue_min"=w247:i32)  [unwired: 11 in]
              n100 = call "myRIO_BRig_RT_dataExp_Tcycle_Cue_max.vi"() -> ("output_Tcycle_Cue_max"=w246:i32)  [unwired: 11 in]
              n101 = Index Array(array=w239, index #1=w289, index #2=w287, index #3=w285, index #4=w284, index #5=w283, index #6=w281, index #7=w280, index #8=w277, index #9=w276, index #10=w275, index #11=w271, index #12=w268, index #13=w267, index #14=w266, index #15=w265, index #16=w260, index #17=w259, index #18=w258, index #19=w257, index #20=w256, index #21=w255, index #22=w248, index #23=w247, index #24=w246, index #25=w236, index #26=w235, index #27=w234, index #28=w233, index #29=w232, index #30=w231) -> (element #1=w288:u16, element #2=w286:u16, element #3=w243:u16, element #4=w242:u16, element #5=w282:u16, element #6=w279:u16, element #7=w278:u16, element #8=w274:u16, element #9=w273:u16, element #10=w272:u16, element #11=w269:u16, element #12=w264:u16, element #13=w263:u16, element #14=w262:u16, element #15=w261:u16, element #16=w254:u16, element #17=w253:u16, element #18=w252:u16, element #19=w251:u16, element #20=w250:u16, element #21=w249:u16, element #22=w245:u16, element #23=w238:u16, element #24=w237:u16, element #25=w230:u16, element #26=w221:u16, element #27=w220:u16, element #28=w219:u16, element #29=w218:u16, element #30=w214:u16)
              n102 = To Double Precision Float(number=w230) -> (double precision float=w229:dbl)
              n103 = To Double Precision Float(number=w221) -> (double precision float=w227:dbl)
              n104 = To Double Precision Float(number=w220) -> (double precision float=w225:dbl)
              n105 = To Double Precision Float(number=w219) -> (double precision float=w224:dbl)
              n106 = To Double Precision Float(number=w218) -> (double precision float=w223:dbl)
              n107 = local write "Tcycle_Selection"(w251) -> ()
              n108 = local write "Tcycle_Wrong"(w250) -> ()
              n109 = local write "Tcycle_Timeout"(w249) -> ()
              n110 = local write "Audio_Amp__L"(w288) -> ()
              n111 = local write "Audio_Amp__R"(w286) -> ()
              n112 = Divide(x=w229, y=w222) -> (x/y=w228:dbl)
              n113 = Divide(x=w227, y=w222) -> (x/y=w226:dbl)
              n114 = Divide(x=w225, y=w222) -> (x/y=w217:dbl)
              n115 = Divide(x=w224, y=w222) -> (x/y=w216:dbl)
              n116 = Divide(x=w223, y=w222) -> (x/y=w215:dbl)
              n117 = local write "Tcycle_ENLPenalty"(w272) -> ()
              n118 = local write "Tcycle_ENL_max"(w274) -> ()
              n119 = local write "laser_duration"(w214) -> ()
              n120 = local write "TpB_Min_L"(w262) -> ()
              n121 = local write "TpB_Min_R"(w261) -> ()
              n122 = local write "laser_power"(w217) -> ()
              n123 = local write "f_millisec2count"(w228) -> ()
              n124 = local write "laser_Tshutter"(w215) -> ()
              n125 = local write "laser_Tpeak"(w216) -> ()
              n126 = local write "laser_Freq"(w226) -> ()
              n127 = local write "Tcycle_CuePenalty"(w245) -> ()
              n128 = local write "Tcycle_Cue_min"(w238) -> ()
              n129 = local write "Tcycle_Cue_max"(w237) -> ()
              n130 = Quotient & Remainder(x=w243, y=w240) -> (floor(x/y)=w244:u16)  [unwired: 1 out]
              n131 = Quotient & Remainder(x=w242, y=w240) -> (floor(x/y)=w241:u16)  [unwired: 1 out]
              n132 = Not Equal To 0?(x=w269) -> (x != 0?=w270:bool)
              n133 = local write "Tcycle_Reward_L"(w254) -> ()
              n134 = local write "Tcycle_Reward_R"(w253) -> ()
              n135 = local write "Tcycle_RewardPost"(w252) -> ()
              n136 = local write "CueCycles"(w282) -> ()
              n137 = local write "BUR_min"(w278) -> ()
              n138 = local write "BUR_max"(w279) -> ()
              n139 = local write "Tcycle_ENL_min"(w273) -> ()
              n140 = local write "TpB_Max_L"(w264) -> ()
              n141 = local write "TpB_Max_R"(w263) -> ()
              n142 = local write "TrialUntilReward"(w270) -> ()
              n143 = local write "Audio_Freq__L"(w244) -> ()
              n144 = local write "Audio_Freq__R"(w241) -> ()
            }
            frame "UploadSettings_dataLC_1" {
              # "Cue1_All_delayOpt"
              # "ENL1_All_delayOpt"
              # "Cue1_First_delayOpt"
              # "ENL1_First_delayOpt"
              # "ENL1 First"
              # "Cue1 All"
              # "Cue1 First"
              # "Count"
              # "Tdelay"
              # "Prob"
              # "OnOff"
              # "Block"
              # "ENL1 All"
              # "Count"
              # "Tdelay"
              # "Prob"
              # "OnOff"
              # "Block"
              # "Count"
              # "Tdelay"
              # "Prob"
              # "Block"
              # "OnOff"
              # "Count"
              # "Tdelay"
              # "Prob"
              # "OnOff"
              # "Block"
              n145 = call "myRIO_BRig_RT_dataLC_Cue1_First_Block.vi"() -> ("output_Cue1_First_Block"=w352:i32)  [unwired: 11 in]
              n146 = call "myRIO_BRig_RT_dataLC_Cue1_First_OnOff.vi"() -> ("output_Cue1_First_OnOff"=w350:i32)  [unwired: 11 in]
              n147 = call "myRIO_BRig_RT_dataLC_Cue1_First_Count.vi"() -> ("output_Cue1_First_Count"=w347:i32)  [unwired: 11 in]
              n148 = call "myRIO_BRig_RT_dataLC_Cue1_All_Block.vi"() -> ("output_Cue1_All_Block"=w334:i32)  [unwired: 11 in]
              n149 = call "myRIO_BRig_RT_dataLC_Cue1_All_OnOff.vi"() -> ("output_Cue1_All_OnOff"=w333:i32)  [unwired: 11 in]
              n150 = call "myRIO_BRig_RT_dataLC_Cue1_All_Count.vi"() -> ("output_Cue1_All_Count"=w344:i32)  [unwired: 11 in]
              n151 = call "myRIO_BRig_RT_dataLC_ENL1_First_Block.vi"() -> ("output_ENL1_First_Block"=w332:i32)  [unwired: 11 in]
              n152 = call "myRIO_BRig_RT_dataLC_ENL1_First_OnOff.vi"() -> ("output_ENL1_First_OnOff"=w343:i32)  [unwired: 11 in]
              n153 = call "myRIO_BRig_RT_dataLC_ENL1_First_Count.vi"() -> ("output_ENL1_First_Count"=w340:i32)  [unwired: 11 in]
              n154 = call "myRIO_BRig_RT_dataLC_ENL1_All_Block.vi"() -> ("output_ENL1_All_Block"=w339:i32)  [unwired: 11 in]
              n155 = call "myRIO_BRig_RT_dataLC_ENL1_All_OnOff.vi"() -> ("output_ENL1_All_OnOff"=w338:i32)  [unwired: 11 in]
              n156 = call "myRIO_BRig_RT_dataLC_ENL1_All_Count.vi"() -> ("output_ENL1_All_Count"=w335:i32)  [unwired: 11 in]
              n157 = call "myRIO_BRig_RT_dataLC_ENL1_First_delayOpt.vi"() -> ("output_ENL1_First_delayOpt"=w309:i32)  [unwired: 11 in]
              n158 = call "myRIO_BRig_RT_dataLC_Cue1_First_delayOpt.vi"() -> ("output_Cue1_First_delayOpt"=w308:i32)  [unwired: 11 in]
              n159 = call "myRIO_BRig_RT_dataLC_ENL1_All_delayOpt.vi"() -> ("output_ENL1_All_delayOpt"=w301:i32)  [unwired: 11 in]
              n160 = call "myRIO_BRig_RT_dataLC_Cue1_All_delayOpt.vi"() -> ("output_Cue1_All_delayOpt"=w300:i32)  [unwired: 11 in]
              n161 = call "myRIO_BRig_RT_dataLC_Cue1_First_Probability.vi"() -> ("output_Cue1_First_Probability"=w349:i32)  [unwired: 11 in]
              n162 = call "myRIO_BRig_RT_dataLC_Cue1_First_Tdelay.vi"() -> ("output_Cue1_First_Tdelay"=w348:i32)  [unwired: 11 in]
              n163 = call "myRIO_BRig_RT_dataLC_Cue1_All_Probability.vi"() -> ("output_Cue1_All_Probability"=w346:i32)  [unwired: 11 in]
              n164 = call "myRIO_BRig_RT_dataLC_Cue1_All_Tdelay.vi"() -> ("output_Cue1_All_Tdelay"=w345:i32)  [unwired: 11 in]
              n165 = call "myRIO_BRig_RT_dataLC_ENL1_First_Probability.vi"() -> ("output_ENL1_First_Probability"=w342:i32)  [unwired: 11 in]
              n166 = call "myRIO_BRig_RT_dataLC_ENL1_First_Tdelay.vi"() -> ("output_ENL1_First_Tdelay"=w341:i32)  [unwired: 11 in]
              n167 = call "myRIO_BRig_RT_dataLC_ENL1_All_Probability.vi"() -> ("output_ENL1_All_Probability"=w337:i32)  [unwired: 11 in]
              n168 = call "myRIO_BRig_RT_dataLC_ENL1_All_Tdelay.vi"() -> ("output_ENL1_All_Tdelay"=w336:i32)  [unwired: 11 in]
              n169 = Index Array(array=w310, index #1=w352, index #2=w350, index #3=w349, index #4=w348, index #5=w347, index #6=w334, index #7=w333, index #8=w346, index #9=w345, index #10=w344, index #11=w332, index #12=w343, index #13=w342, index #14=w341, index #15=w340, index #16=w339, index #17=w338, index #18=w337, index #19=w336, index #20=w335, index #21=w309, index #22=w308, index #23=w301, index #24=w300) -> (element #1=w351:u16, element #2=w330:u16, element #3=w329:u16, element #4=w328:u16, element #5=w327:u16, element #6=w323:u16, element #7=w322:u16, element #8=w321:u16, element #9=w320:u16, element #10=w319:u16, element #11=w318:u16, element #12=w317:u16, element #13=w316:u16, element #14=w315:u16, element #15=w302:u16, element #16=w314:u16, element #17=w313:u16, element #18=w312:u16, element #19=w311:u16, element #20=w303:u16, element #21=w306:u16, element #22=w304:u16, element #23=w297:u16, element #24=w296:u16)
              n170 = Not Equal To 0?(x=w297) -> (x != 0?=w299:bool)
              n171 = Not Equal To 0?(x=w296) -> (x != 0?=w298:bool)
              n172 = Not Equal To 0?(x=w306) -> (x != 0?=w307:bool)
              n173 = Not Equal To 0?(x=w304) -> (x != 0?=w305:bool)
              n174 = Not Equal To 0?(x=w330) -> (x != 0?=w331:bool)
              n175 = Not Equal To 0?(x=w322) -> (x != 0?=w326:bool)
              n176 = Not Equal To 0?(x=w317) -> (x != 0?=w325:bool)
              n177 = Not Equal To 0?(x=w313) -> (x != 0?=w324:bool)
              n178 = local write "LC_Cue1_First_Probability"(w329) -> ()
              n179 = local write "LC_ENL1_First_Probability"(w316) -> ()
              n180 = local write "LC_ENL1_First_delayOpt"(w307) -> ()
              n181 = local write "LC_Cue1_First_delayOpt"(w305) -> ()
              n182 = local write "LC_ENL1_All_delayOpt"(w299) -> ()
              n183 = local write "LC_Cue1_All_delayOpt"(w298) -> ()
              n184 = local write "LC_Cue1_All_Probability"(w321) -> ()
              n185 = local write "LC_Cue1_First_Tdelay"(w328) -> ()
              n186 = local write "LC_ENL1_All_Probability"(w312) -> ()
              n187 = local write "LC_Cue1_First_OnOff"(w331) -> ()
              n188 = local write "LC_Cue1_First_Count"(w327) -> ()
              n189 = local write "LC_Cue1_First_Block"(w351) -> ()
              n190 = local write "LC_ENL1_First_Tdelay"(w315) -> ()
              n191 = local write "LC_ENL1_First_OnOff"(w325) -> ()
              n192 = local write "LC_ENL1_First_Count"(w302) -> ()
              n193 = local write "LC_ENL1_First_Block"(w318) -> ()
              n194 = local write "LC_Cue1_All_Tdelay"(w320) -> ()
              n195 = local write "LC_Cue1_All_OnOff"(w326) -> ()
              n196 = local write "LC_Cue1_All_Count"(w319) -> ()
              n197 = local write "LC_Cue1_All_Block"(w323) -> ()
              n198 = local write "LC_ENL1_All_Tdelay"(w311) -> ()
              n199 = local write "LC_ENL1_All_OnOff"(w324) -> ()
              n200 = local write "LC_ENL1_All_Count"(w303) -> ()
              n201 = local write "LC_ENL1_All_Block"(w314) -> ()
            }
            frame "UploadSettings_dataLC_2" {
              # "Wrong"
              # "Reward"
              # "Trial"
              # "Tdelay"
              # "Prob"
              # "Block"
              # "OnOff"
              # "Trial"
              # "Tdelay"
              # "Prob"
              # "OnOff"
              # "Block"
              n202 = call "myRIO_BRig_RT_dataLC_Reward_Block.vi"() -> ("output_Reward_Block"=w385:i32)  [unwired: 11 in]
              n203 = call "myRIO_BRig_RT_dataLC_Reward_OnOff.vi"() -> ("output_Reward_OnOff"=w383:i32)  [unwired: 11 in]
              n204 = call "myRIO_BRig_RT_dataLC_Reward_Trial.vi"() -> ("output_Reward_Trial"=w380:i32)  [unwired: 11 in]
              n205 = call "myRIO_BRig_RT_dataLC_Wrong_Block.vi"() -> ("output_Wrong_Block"=w376:i32)  [unwired: 11 in]
              n206 = call "myRIO_BRig_RT_dataLC_Wrong_OnOff.vi"() -> ("output_Wrong_OnOff"=w375:i32)  [unwired: 11 in]
              n207 = call "myRIO_BRig_RT_dataLC_Wrong_Trial.vi"() -> ("output_Wrong_Trial"=w377:i32)  [unwired: 11 in]
              n208 = call "myRIO_BRig_RT_dataLC_Reward_Probability.vi"() -> ("output_Reward_Probability"=w382:i32)  [unwired: 11 in]
              n209 = call "myRIO_BRig_RT_dataLC_Reward_Tdelay.vi"() -> ("output_Reward_Tdelay"=w381:i32)  [unwired: 11 in]
              n210 = call "myRIO_BRig_RT_dataLC_Wrong_Probability.vi"() -> ("output_Wrong_Probability"=w379:i32)  [unwired: 11 in]
              n211 = call "myRIO_BRig_RT_dataLC_Wrong_Tdelay.vi"() -> ("output_Wrong_Tdelay"=w378:i32)  [unwired: 11 in]
              n212 = Index Array(array=w359, index #1=w385, index #2=w383, index #3=w382, index #4=w381, index #5=w380, index #6=w376, index #7=w375, index #8=w379, index #9=w378, index #10=w377) -> (element #1=w384:u16, element #2=w373:u16, element #3=w372:u16, element #4=w371:u16, element #5=w370:u16, element #6=w368:u16, element #7=w367:u16, element #8=w366:u16, element #9=w365:u16, element #10=w364:u16)
              n213 = Not Equal To 0?(x=w373) -> (x != 0?=w374:bool)
              n214 = Not Equal To 0?(x=w367) -> (x != 0?=w369:bool)
              n215 = local write "LC_Reward_Probability"(w372) -> ()
              n216 = local write "LC_Wrong_Probability"(w366) -> ()
              n217 = local write "LC_Reward_Tdelay"(w371) -> ()
              n218 = local write "LC_Reward_OnOff"(w374) -> ()
              n219 = local write "LC_Reward_Block"(w384) -> ()
              n220 = local write "LC_Reward_Trial"(w370) -> ()
              n221 = local write "LC_Wrong_Tdelay"(w365) -> ()
              n222 = local write "LC_Wrong_OnOff"(w369) -> ()
              n223 = local write "LC_Wrong_Block"(w368) -> ()
              n224 = local write "LC_Wrong_Trial"(w364) -> ()
            }
            frame "UploadSettings_dataMTrig_1" {
              # "Tdelay_R"
              # "Tdelay_L"
              # "Tcycle_R"
              # "Tcycle_L"
              # "RewCalib_nCycle_R"
              # "RewCalib_nCycle_L"
              # "Solenoid"
              # "Laser_Tcycle"
              n225 = call "myRIO_BRig_RT_dataMTrig_Laser_Tcycle.vi"() -> ("output_Laser_Tcycle"=w395:i32)  [unwired: 11 in]
              n226 = call "myRIO_BRig_RT_dataMTrig_Solenoid_RewCalib_nCycle__L.vi"() -> ("output_Solenoid_RewCalib_nCycle__L"=w394:i32)  [unwired: 11 in]
              n227 = call "myRIO_BRig_RT_dataMTrig_Solenoid_RewCalib_nCycle__R.vi"() -> ("output_Solenoid_RewCalib_nCycle__R"=w393:i32)  [unwired: 11 in]
              n228 = call "myRIO_BRig_RT_dataMTrig_Solenoid_Tdelay__L.vi"() -> ("output_Solenoid_Tdelay__L"=w390:i32)  [unwired: 11 in]
              n229 = call "myRIO_BRig_RT_dataMTrig_Solenoid_Tdelay__R.vi"() -> ("output_Solenoid_Tdelay__R"=w389:i32)  [unwired: 11 in]
              n230 = call "myRIO_BRig_RT_dataMTrig_Solenoid_Tcycle__L.vi"() -> ("output_Solenoid_Tcycle__L"=w392:i32)  [unwired: 11 in]
              n231 = call "myRIO_BRig_RT_dataMTrig_Solenoid_Tcycle__R.vi"() -> ("output_Solenoid_Tcycle__R"=w391:i32)  [unwired: 11 in]
              n232 = Index Array(array=w388, index #1=w395, index #2=w394, index #3=w393, index #4=w392, index #5=w391, index #6=w390, index #7=w389) -> (element #1=w402:u16, element #2=w401:u16, element #3=w400:u16, element #4=w399:u16, element #5=w398:u16, element #6=w397:u16, element #7=w396:u16)
              n233 = Replace Array Subset(array=w408, new element #1=w402, index #1=w395, new element #2=w401, index #2=w394, new element #3=w400, index #3=w393, new element #4=w399, index #4=w392, new element #5=w398, index #5=w391, new element #6=w397, index #6=w390, new element #7=w396, index #7=w389) -> (w407:u16[])
              n234 = local write "MTrig_Solenoid_Tcycle__L"(w399) -> ()
              n235 = local write "MTrig_Solenoid_Tcycle__R"(w398) -> ()
              n236 = local write "MTrig_Laser_Tcycle"(w402) -> ()
            }
            frame "Idle" {
              w428 = u16 1000 ("y")
              # "To ensure timing, we split the\nidle state into 4 phases"
              # "Laser_Tcycle"
              # "Audio_Tcycle_R"
              # "Audio_Tcycle_L"
              n237 = local read "MTrig_Audio_trig__L"() -> (w417:bool)
              n238 = local read "MTrig_Audio_trig__R"() -> (w419:bool)
              n239 = Select(t=myRIO_BRig_RT__Case_NonExp_stateList."SendData" ("Enum"), s="SendData", f=myRIO_BRig_RT__Case_NonExp_stateList."Idle_2" ("Enum")) -> (s? t:f=w412:T1)
              n240 = local read "MTrig_Laser_trig"() -> (w418:bool)
              n241 = call "myRIO_BRig_RT_dataMTrig_Audio_Tcycle__L.vi"() -> ("output_Audio_Tcycle__L"=w435:i32)  [unwired: 11 in]
              n242 = call "myRIO_BRig_RT_dataMTrig_Audio_Tcycle__R.vi"() -> ("output_Audio_Tcycle__R"=w434:i32)  [unwired: 11 in]
              n243 = call "myRIO_BRig_RT_dataMTrig_Laser_Tcycle.vi"() -> ("output_Laser_Tcycle"=w433:i32)  [unwired: 11 in]
              n244 = local read "MTrig_Laser_Tcycle"() -> (w410:u16)
              n245 = Select(t=myRIO_BRig_RT__Case_NonExp_stateList."TestConnection" ("Enum"), s="TestConnection", f=w412) -> (s? t:f=w421:T1)
              n246 = local read "Tcycle_Cue_min"() -> (w411:u16)
              n247 = Compound Arithmetic op=OR(w417, w419, w418) -> (w420:bool)
              n248 = case shown="True" w420 {
                frame False {
                }
                frame True {
                  w436 = FALSE
                  n249 = local write "MTrig_Audio_trig__L"(w436) -> ()
                  n250 = local write "MTrig_Audio_trig__R"(w436) -> ()
                  n251 = local write "MTrig_Laser_trig"(w436) -> ()
                }
              }
              n252 = Replace Array Subset(array=w431, new element #1=w411, index #1=w435, new element #2=w411, index #2=w434, new element #3=w410, index #3=w433) -> (w432:u16[])
              n253 = local read "Audio_Amp__R"() -> (w424:u16)
              n254 = local read "Audio_Amp__L"() -> (w425:u16)
              n255 = local read "Audio_Freq__R"() -> (w422:u16)
              n256 = local read "Audio_Freq__L"() -> (w423:u16)
              n257 = Multiply(x=w422, y=w428) -> (x*y=w426:u16)
              n258 = Multiply(x=w423, y=w428) -> (x*y=w427:u16)
            }
            frame "Idle_2" {
              # "To ensure timing, we split the\nidle state into 4 phases"
              # "Ncycles"
              # "Ncycles"
              # "RewCalib"
              # "RewCalib"
              # "Solenoid R"
              # "Solenoid L"
              n259 = call "myRIO_BRig_RT_dataMTrig_Solenoid_RewCalib_OnOff__L.vi"() -> ("output_Solenoid_RewCalib_OnOff__L"=w466:i32)  [unwired: 11 in]
              n260 = call "myRIO_BRig_RT_dataMTrig_Solenoid_N__L.vi"() -> ("output_Solenoid_N__L"=w454:i32)  [unwired: 11 in]
              n261 = call "myRIO_BRig_RT_dataMTrig_Solenoid_RewCalib_OnOff__R.vi"() -> ("output_Solenoid_RewCalib_OnOff__R"=w451:i32)  [unwired: 11 in]
              n262 = call "myRIO_BRig_RT_dataMTrig_Solenoid_N__R.vi"() -> ("output_Solenoid_N__R"=w450:i32)  [unwired: 11 in]
              n263 = Index Array(array=w457, index #1=w466, index #2=w454, index #3=w451, index #4=w450) -> (element #1=w453:u16, element #2=w448:u16, element #3=w449:u16, element #4=w447:u16)
              n264 = local read "RewCalib_Trig_L"() -> (w446:bool)
              n265 = local read "RewCalib_Trig_R"() -> (w445:bool)
              n266 = Equal To 0?(x=w448) -> (x = 0?=w456:bool)
              n267 = Equal To 0?(x=w447) -> (x = 0?=w455:bool)
              n268 = Not Equal To 0?(x=w449) -> (x != 0?=w467:bool)
              n269 = Not Equal To 0?(x=w453) -> (x != 0?=w468:bool)
              n270 = And(x=w456, y=w455) -> (x .and. y?=w460:bool)
              n271 = Or(x=w446, y=w445) -> (x .or. y?=w461:bool)
              n272 = Not Exclusive Or(1:w468, 2:w446) -> (0:w463:bool)
              n273 = Not Exclusive Or(1:w467, 2:w445) -> (0:w465:bool)
              n274 = And(x=w461, y=w460) -> (x .and. y?=w443:bool)
              n275 = Not(x=w463) -> (.not. x?=w462:bool)
              n276 = Not(x=w465) -> (.not. x?=w464:bool)
              n277 = Or(x=w462, y=w464) -> (x .or. y?=w444:bool)
              n278 = Or(x=w443, y=w444) -> (x .or. y?=w459:bool)
              n279 = Select(t=myRIO_BRig_RT__Case_NonExp_stateList."RewardCalibration_pre" ("Enum"), s=w459, f=myRIO_BRig_RT__Case_NonExp_stateList."Idle_3" ("Enum")) -> (s? t:f=w442:T1)
            }
            frame "Idle_3" {
              w491 = u8 0 ("f")
              # "To ensure timing, we split the\nidle state into 4 phases"
              n280 = local read "MTrig_Solenoid_trig__L"() -> (w477:bool)
              n281 = local read "MTrig_Solenoid_trig__R"() -> (w492:bool)
              n282 = local read "warmupType"() -> (w483:bool)
              n283 = local read "warmup"() -> (w484:bool)
              n284 = Not(x=w483) -> (.not. x?=w485:bool)
              n285 = Select(t=u8 1, s=w477, f=w491) -> (s? t:f=w490:u8)
              n286 = Select(t=u8 2, s=w492, f=w491) -> (s? t:f=w489:u8)
              n287 = And(x=w484, y=w485) -> (x .and. y?=w482:bool)
              n288 = And(x=w484, y=w483) -> (x .and. y?=w472:bool)
              n289 = Add(x=w490, y=w489) -> (x+y=w488:u8)
              n290 = case shown="3" w488 {
                tunnel: w487 -> [w495 w499 w517 w535]
                tunnel: [w495 w498 w516 w534] -> w486
                tunnel: w482 -> [_ w497 w515 w533]
                tunnel: [_ TRUE TRUE TRUE] -> w474
                frame 0, Default {
                }
                frame 1 {
                  n291 = case shown="True" w497 {
                    tunnel: w499 -> [w508 w513]
                    tunnel: [w507 w512] -> w498
                    frame True {
                      # "Audio_L"
                      # "Solenoid_L"
                      n292 = call "myRIO_BRig_RT_dataMTrig_Solenoid_N__L.vi"() -> ("output_Solenoid_N__L"=w504:i32)  [unwired: 11 in]
                      n293 = call "myRIO_BRig_RT_dataMTrig_Audio_N__L.vi"() -> ("output_Audio_N__L"=w502:i32)  [unwired: 11 in]
                      n294 = Index Array(array=w508, index #1=w504, index #2=w502) -> (element #1=w506:u16, element #2=w505:u16)
                      n295 = Increment(x=w506) -> (x+1=w503:u16)
                      n296 = Increment(x=w505) -> (x+1=w501:u16)
                      n297 = Replace Array Subset(array=w508, new element #1=w503, index #1=w504, new element #2=w501, index #2=w502) -> (w507:u16[])
                    }
                    frame False {
                      # "Solenoid_L"
                      n298 = call "myRIO_BRig_RT_dataMTrig_Solenoid_N__L.vi"() -> ("output_Solenoid_N__L"=w510:i32)  [unwired: 11 in]
                      n299 = Index Array(array=w513, index=w510) -> (element=w511:u16)
                      n300 = Increment(x=w511) -> (x+1=w509:u16)
                      n301 = Replace Array Subset(array=w513, new element=w509, index=w510) -> (w512:u16[])
                    }
                  }
                  n302 = local write "MTrig_Solenoid_trig__L"(FALSE) -> ()
                }
                frame 2 {
                  n303 = case shown="True" w515 {
                    tunnel: w517 -> [w526 w531]
                    tunnel: [w525 w530] -> w516
                    frame True {
                      # "Audio_R"
                      # "Solenoid_R"
                      n304 = call "myRIO_BRig_RT_dataMTrig_Solenoid_N__R.vi"() -> ("output_Solenoid_N__R"=w522:i32)  [unwired: 11 in]
                      n305 = call "myRIO_BRig_RT_dataMTrig_Audio_N__R.vi"() -> ("output_Audio_N__R"=w521:i32)  [unwired: 11 in]
                      n306 = Index Array(array=w526, index #1=w522, index #2=w521) -> (element #1=w524:u16, element #2=w523:u16)
                      n307 = Increment(x=w523) -> (x+1=w519:u16)
                      n308 = Increment(x=w524) -> (x+1=w520:u16)
                      n309 = Replace Array Subset(array=w526, new element #1=w520, index #1=w522, new element #2=w519, index #2=w521) -> (w525:u16[])
                    }
                    frame False {
                      # "Solenoid_R"
                      n310 = call "myRIO_BRig_RT_dataMTrig_Solenoid_N__R.vi"() -> ("output_Solenoid_N__R"=w527:i32)  [unwired: 11 in]
                      n311 = Index Array(array=w531, index=w527) -> (element=w529:u16)
                      n312 = Increment(x=w529) -> (x+1=w528:u16)
                      n313 = Replace Array Subset(array=w531, new element=w528, index=w527) -> (w530:u16[])
                    }
                  }
                  n314 = local write "MTrig_Solenoid_trig__R"(FALSE) -> ()
                }
                frame 3 {
                  w536 = FALSE
                  n315 = case shown="True" w533 {
                    tunnel: w535 -> [w550 w558]
                    tunnel: [w549 w557] -> w534
                    frame True {
                      # "Audio_R"
                      # "Solenoid_R"
                      # "Audio_L"
                      # "Solenoid_L"
                      n316 = call "myRIO_BRig_RT_dataMTrig_Solenoid_N__L.vi"() -> ("output_Solenoid_N__L"=w544:i32)  [unwired: 11 in]
                      n317 = call "myRIO_BRig_RT_dataMTrig_Audio_N__L.vi"() -> ("output_Audio_N__L"=w542:i32)  [unwired: 11 in]
                      n318 = call "myRIO_BRig_RT_dataMTrig_Solenoid_N__R.vi"() -> ("output_Solenoid_N__R"=w540:i32)  [unwired: 11 in]
                      n319 = call "myRIO_BRig_RT_dataMTrig_Audio_N__R.vi"() -> ("output_Audio_N__R"=w539:i32)  [unwired: 11 in]
                      n320 = Index Array(array=w550, index #1=w544, index #2=w542, index #3=w540, index #4=w539) -> (element #1=w548:u16, element #2=w547:u16, element #3=w546:u16, element #4=w545:u16)
                      n321 = Increment(x=w545) -> (x+1=w537:u16)
                      n322 = Increment(x=w548) -> (x+1=w543:u16)
                      n323 = Increment(x=w547) -> (x+1=w541:u16)
                      n324 = Increment(x=w546) -> (x+1=w538:u16)
                      n325 = Replace Array Subset(array=w550, new element #1=w543, index #1=w544, new element #2=w541, index #2=w542, new element #3=w538, index #3=w540, new element #4=w537, index #4=w539) -> (w549:u16[])
                    }
                    frame False {
                      # "Solenoid_R"
                      # "Solenoid_L"
                      n326 = call "myRIO_BRig_RT_dataMTrig_Solenoid_N__L.vi"() -> ("output_Solenoid_N__L"=w554:i32)  [unwired: 11 in]
                      n327 = call "myRIO_BRig_RT_dataMTrig_Solenoid_N__R.vi"() -> ("output_Solenoid_N__R"=w551:i32)  [unwired: 11 in]
                      n328 = Index Array(array=w558, index #1=w554, index #2=w551) -> (element #1=w556:u16, element #2=w555:u16)
                      n329 = Increment(x=w556) -> (x+1=w553:u16)
                      n330 = Increment(x=w555) -> (x+1=w552:u16)
                      n331 = Replace Array Subset(array=w558, new element #1=w553, index #1=w554, new element #2=w552, index #2=w551) -> (w557:u16[])
                    }
                  }
                  n332 = local write "MTrig_Solenoid_trig__L"(w536) -> ()
                  n333 = local write "MTrig_Solenoid_trig__R"(w536) -> ()
                }
              }
              n334 = Select(t=myRIO_BRig_RT__Case_NonExp_stateList."Cue_pre", s=w472, f=myRIO_BRig_RT__Case_NonExp_stateList."DispenseWater_pre" ("Enum")) -> (s? t:f=w470:T1)
              n335 = Select(t=w470, s=w474, f=myRIO_BRig_RT__Case_NonExp_stateList."Idle_4" ("Enum")) -> (s? t:f=w475:T1)
            }
            frame "Idle_4" {
              # "use dataMTrig as it is one of the last to transfer"
              # "To ensure timing, we split the\nidle state into 4 phases"
              n336 = call "myRIO_BRig_RT_comm_webdav_uploadReceived_check_v2,0.vi"("input_dataName"="dataMTrig") -> ("output_Iexist"=w568:bool)  [unwired: 9 in, 1 out]
              n337 = Select(t=myRIO_BRig_RT__Case_NonExp_stateList."UploadSettings_pre" ("Enum"), s=w568, f=myRIO_BRig_RT__Case_NonExp_stateList."Idle") -> (s? t:f=w566:T1)
            }
            frame "Cue_pre" {
              w576 = u16 1 ("t")
              w575 = u16 0 ("new element/subarray")
              w572 = u16 0 ("new element/subarray")
              # "Ncycle"
              # "count"
              # "Audio_R"
              # "Solenoid_R"
              # "Solenoid_L"
              # "Ncycle"
              # "count"
              # "Audio_L"
              n338 = call "myRIO_BRig_RT_dataMTrig_Solenoid_N__L.vi"() -> ("output_Solenoid_N__L"=w587:i32)  [unwired: 11 in]
              n339 = call "myRIO_BRig_RT_dataMTrig_Solenoid_N__R.vi"() -> ("output_Solenoid_N__R"=w586:i32)  [unwired: 11 in]
              n340 = Index Array(array=w583, index #1=w587, index #2=w586) -> (element #1=w585:u16, element #2=w584:u16)
              n341 = Not Equal To 0?(x=w584) -> (x != 0?=w577:bool)
              n342 = Not Equal To 0?(x=w585) -> (x != 0?=w579:bool)
              n343 = Select(t=w576, s=w579, f=w575) -> (s? t:f=w578:u16)
              n344 = Select(t=w576, s=w577, f=w575) -> (s? t:f=w571:u16)
              n345 = call "myRIO_BRig_RT_dataMTrig_Audio_c__L.vi"() -> ("output_Audio_c__L"=w581:i32)  [unwired: 11 in]
              n346 = call "myRIO_BRig_RT_dataMTrig_Audio_N__L.vi"() -> ("output_Audio_N__L"=w580:i32)  [unwired: 11 in]
              n347 = call "myRIO_BRig_RT_dataMTrig_Audio_c__R.vi"() -> ("output_Audio_c__R"=w574:i32)  [unwired: 11 in]
              n348 = call "myRIO_BRig_RT_dataMTrig_Audio_N__R.vi"() -> ("output_Audio_N__R"=w573:i32)  [unwired: 11 in]
              n349 = Replace Array Subset(array=w583, new element #1=w572, index #1=w581, new element #2=w578, index #2=w580, new element #3=w572, index #3=w574, new element #4=w571, index #4=w573) -> (w582:u16[])
            }
            frame "Cue" {
              # "Ncycle"
              # "Audio_R"
              # "Ncycle"
              # "Audio_L"
              n350 = call "myRIO_BRig_RT_dataMTrig_Audio_N__L.vi"() -> ("output_Audio_N__L"=w603:i32)  [unwired: 11 in]
              n351 = call "myRIO_BRig_RT_dataMTrig_Audio_N__R.vi"() -> ("output_Audio_N__R"=w602:i32)  [unwired: 11 in]
              n352 = Index Array(array=w608, index #1=w603, index #2=w602) -> (element #1=w601:u16, element #2=w600:u16)
              n353 = Equal To 0?(x=w601) -> (x = 0?=w599:bool)
              n354 = Equal To 0?(x=w600) -> (x = 0?=w598:bool)
              n355 = And(x=w599, y=w598) -> (x .and. y?=w597:bool)
              n356 = Select(t=myRIO_BRig_RT__Case_NonExp_stateList."DispenseWater_pre", s=w597, f=w595) -> (s? t:f=w594:T1)
            }
            frame "RewardCalibration_pre" {
              (unwired) FALSE
              w614 = FALSE
              w625 = u8 0
              w641 = u8 0
              # "Are we starting a RewardCalibration?\nOr are we stopping a RewardCalibration?\nOr is a RewardCalibration over?"
              # "RewCalib\nOnOff"
              # "N"
              # "Solenoid R"
              # "RewCalib\nOnOff"
              # "N"
              # "Solenoid L"
              n357 = local read "RewCalib_Trig_L"() -> (w648:bool)
              n358 = local read "RewCalib_Trig_R"() -> (w617:bool)
              n359 = call "myRIO_BRig_RT_dataMTrig_Solenoid_N__R.vi"() -> ("output_Solenoid_N__R"=w619:i32)  [unwired: 11 in]
              n360 = call "myRIO_BRig_RT_dataMTrig_Solenoid_RewCalib_OnOff__R.vi"() -> ("output_Solenoid_RewCalib_OnOff__R"=w616:i32)  [unwired: 11 in]
              n361 = call "myRIO_BRig_RT_dataMTrig_Solenoid_N__L.vi"() -> ("output_Solenoid_N__L"=w634:i32)  [unwired: 11 in]
              n362 = call "myRIO_BRig_RT_dataMTrig_Solenoid_RewCalib_OnOff__L.vi"() -> ("output_Solenoid_RewCalib_OnOff__L"=w635:i32)  [unwired: 11 in]
              n363 = Index Array(array=w618, index #1=w619, index #2=w616) -> (element #1=w629:u16, element #2=w624:u16)
              n364 = Index Array(array=w618, index #1=w634, index #2=w635) -> (element #1=w645:u16, element #2=w640:u16)
              n365 = Equal To 0?(x=w629) -> (x = 0?=w630:bool)
              n366 = Not Equal To 0?(x=w624) -> (x != 0?=w627:bool)
              n367 = Equal To 0?(x=w645) -> (x = 0?=w646:bool)
              n368 = Not Equal To 0?(x=w640) -> (x != 0?=w643:bool)
              n369 = local write "MTrig_Solenoid_trig__L"(w614) -> ()
              n370 = local write "MTrig_Solenoid_trig__R"(w614) -> ()
              n371 = Select(t=u8 1, s=w617, f=w625) -> (s? t:f=w621:u8)
              n372 = Select(t=u8 1, s=w648, f=w641) -> (s? t:f=w637:u8)
              n373 = Select(t=u8 2, s=w630, f=w625) -> (s? t:f=w622:u8)
              n374 = Select(t=u8 4, s=w627, f=w625) -> (s? t:f=w623:u8)
              n375 = Select(t=u8 2, s=w646, f=w641) -> (s? t:f=w638:u8)
              n376 = Select(t=u8 4, s=w643, f=w641) -> (s? t:f=w639:u8)
              n377 = Compound Arithmetic op=ADD(w621, w622, w623) -> (w620:u8)
              n378 = Compound Arithmetic op=ADD(w637, w638, w639) -> (w636:u8)
              n379 = case shown="7" w636 {
                tunnel: w618 -> [w678 w683 w685 w690 w695 w697 w700 w705]
                tunnel: [w678 w684 w685 w691 w696 w697 w701 w706] -> w633
                tunnel: w635 -> [_ w681 _ w688 w693 _ w699 w704]
                tunnel: w634 -> [_ w682 _ w689 w694 _ _ _]
                frame 0, Default {
                }
                frame 1 {
                  n380 = Replace Array Subset(array=w683, new element #1=u16 100 ("new element/subarray"), index #1=w682, new element #2=u16 1 ("new element/subarray"), index #2=w681) -> (w684:u16[])
                }
                frame 2 {
                }
                frame 3 {
                  n381 = Replace Array Subset(array=w690, new element #1=u16 100 ("new element/subarray"), index #1=w689, new element #2=u16 1 ("new element/subarray"), index #2=w688) -> (w691:u16[])
                }
                frame 4 {
                  w692 = u16 0 ("new element/subarray")
                  n382 = Replace Array Subset(array=w695, new element #1=w692, index #1=w694, new element #2=w692, index #2=w693) -> (w696:u16[])
                }
                frame 5 {
                }
                frame 6 {
                  n383 = Replace Array Subset(array=w700, new element=u16 0 ("new element/subarray"), index=w699) -> (w701:u16[])
                }
                frame 7 {
                  n384 = local write "RewCalib_Trig_L"(FALSE ("RewCalib_Trig_L")) -> ()
                  n385 = Replace Array Subset(array=w705, new element=u16 0 ("new element/subarray"), index=w704) -> (w706:u16[])
                }
              }
              n386 = case shown="7" w620 {
                tunnel: w633 -> [w649 w654 w656 w661 w666 w668 w671 w676]
                tunnel: [w649 w655 w656 w662 w667 w668 w672 w677] -> w632
                tunnel: w616 -> [_ w652 _ w659 w664 _ w670 w675]
                tunnel: w619 -> [_ w653 _ w660 w665 _ _ _]
                frame 0, Default {
                }
                frame 1 {
                  n387 = Replace Array Subset(array=w654, new element #1=u16 100 ("new element/subarray"), index #1=w653, new element #2=u16 1 ("new element/subarray"), index #2=w652) -> (w655:u16[])
                }
                frame 2 {
                }
                frame 3 {
                  n388 = Replace Array Subset(array=w661, new element #1=u16 100 ("new element/subarray"), index #1=w660, new element #2=u16 1 ("new element/subarray"), index #2=w659) -> (w662:u16[])
                }
                frame 4 {
                  w663 = u16 0 ("new element/subarray")
                  n389 = Replace Array Subset(array=w666, new element #1=w663, index #1=w665, new element #2=w663, index #2=w664) -> (w667:u16[])
                }
                frame 5 {
                }
                frame 6 {
                  n390 = Replace Array Subset(array=w671, new element=u16 0 ("new element/subarray"), index=w670) -> (w672:u16[])
                }
                frame 7 {
                  n391 = local write "RewCalib_Trig_R"(FALSE ("RewCalib_Trig_L")) -> ()
                  n392 = Replace Array Subset(array=w676, new element=u16 0 ("new element/subarray"), index=w675) -> (w677:u16[])
                }
              }
            }
            frame "DispenseWater_pre" {
              w713 = u16 0 ("t")
              w756 = u16 0 ("new element/subarray")
              # "just trust me on this one"
              # "RewCalib\nOnOff"
              # "RewCalib\nOnOff"
              # "nCycle"
              # "Solenoid__R"
              # "Tdelay"
              # "delay"
              # "nCycle"
              # "Solenoid__L"
              # "Tdelay"
              # "delay"
              # "Solenoid__R"
              # "count"
              # "Solenoid_Tcycle_R"
              # "Solenoid_Tcycle_L"
              # "Solenoid__L"
              # "count"
              n393 = call "myRIO_BRig_RT_dataMTrig_Solenoid_RewCalib_OnOff__L.vi"() -> ("output_Solenoid_RewCalib_OnOff__L"=w720:i32)  [unwired: 11 in]
              n394 = call "myRIO_BRig_RT_dataMTrig_Solenoid_N__L.vi"() -> ("output_Solenoid_N__L"=w711:i32)  [unwired: 11 in]
              n395 = call "myRIO_BRig_RT_dataMTrig_Solenoid_delay__L.vi"() -> ("output_Solenoid_delay__L"=w754:i32)  [unwired: 11 in]
              n396 = call "myRIO_BRig_RT_dataMTrig_Solenoid_Tdelay__L.vi"() -> ("output_Solenoid_Tdelay__L"=w753:i32)  [unwired: 11 in]
              n397 = call "myRIO_BRig_RT_dataMTrig_Solenoid_N__R.vi"() -> ("output_Solenoid_N__R"=w709:i32)  [unwired: 11 in]
              n398 = call "myRIO_BRig_RT_dataMTrig_Solenoid_delay__R.vi"() -> ("output_Solenoid_delay__R"=w743:i32)  [unwired: 11 in]
              n399 = call "myRIO_BRig_RT_dataMTrig_Solenoid_Tdelay__R.vi"() -> ("output_Solenoid_Tdelay__R"=w742:i32)  [unwired: 11 in]
              n400 = call "myRIO_BRig_RT_dataMTrig_Solenoid_RewCalib_OnOff__R.vi"() -> ("output_Solenoid_RewCalib_OnOff__R"=w716:i32)  [unwired: 11 in]
              n401 = Index Array(array=w755, index #1=w711, index #2=w754, index #3=w753, index #4=w709, index #5=w743, index #6=w742, index #7=w720, index #8=w716) -> (element #1=w712:u16, element #2=w752:u16, element #3=w747:u16, element #4=w715:u16, element #5=w737:u16, element #6=w736:u16, element #7=w721:u16, element #8=w718:u16)
              n402 = Equal To 0?(x=w752) -> (x = 0?=w751:bool)
              n403 = Equal To 0?(x=w737) -> (x = 0?=w741:bool)
              n404 = local read "RewCalib_Trig_L"() -> (w732:bool)
              n405 = local read "RewCalib_Trig_R"() -> (w727:bool)
              n406 = Not Equal To 0?(x=w712) -> (x != 0?=w750:bool)
              n407 = Not Equal To 0?(x=w715) -> (x != 0?=w740:bool)
              n408 = local read "MTrig_Solenoid_Tcycle__L"() -> (w749:u16)
              n409 = local read "MTrig_Solenoid_Tcycle__R"() -> (w735:u16)
              n410 = Not Equal To 0?(x=w721) -> (x != 0?=w731:bool)
              n411 = Not Equal To 0?(x=w718) -> (x != 0?=w729:bool)
              n412 = Not(x=w732) -> (.not. x?=w730:bool)
              n413 = Not(x=w727) -> (.not. x?=w728:bool)
              n414 = And(x=w731, y=w730) -> (x .and. y?=w726:bool)
              n415 = And(x=w729, y=w728) -> (x .and. y?=w725:bool)
              n416 = call "myRIO_BRig_RT_dataMTrig_Solenoid_c__L.vi"() -> ("output_Solenoid_c__L"=w758:i32)  [unwired: 11 in]
              n417 = call "myRIO_BRig_RT_dataMTrig_Solenoid_c__R.vi"() -> ("output_Solenoid_c__R"=w757:i32)  [unwired: 11 in]
              n418 = Select(t=w749, s=w750, f=u16 0) -> (s? t:f=w746:u16)
              n419 = Or(x=w726, y=w725) -> (x .or. y?=w714:bool)
              n420 = Select(t=w735, s=w740, f=u16 0) -> (s? t:f=w738:u16)
              n421 = Select(t=w746, s=w751, f=w747) -> (s? t:f=w744:u16)
              n422 = Select(t=w738, s=w741, f=w736) -> (s? t:f=w733:u16)
              n423 = call "myRIO_BRig_RT_dataMTrig_Solenoid_Tcycle__L.vi"() -> ("output_Solenoid_Tcycle__L"=w745:i32)  [unwired: 11 in]
              n424 = call "myRIO_BRig_RT_dataMTrig_Solenoid_Tcycle__R.vi"() -> ("output_Solenoid_Tcycle__R"=w734:i32)  [unwired: 11 in]
              n425 = Select(t=w713, s=w714, f=w712) -> (s? t:f=w710:u16)
              n426 = Select(t=w713, s=w714, f=w715) -> (s? t:f=w708:u16)
              n427 = Select(t=myRIO_BRig_RT__Case_NonExp_stateList."Idle" ("Enum"), s=w714, f=myRIO_BRig_RT__Case_NonExp_stateList."DispenseWater" ("Enum")) -> (s? t:f=w722:T1)
              n428 = Select(t=w713, s=w714, f=w721) -> (s? t:f=w719:u16)
              n429 = Select(t=w713, s=w714, f=w718) -> (s? t:f=w717:u16)
              n430 = Replace Array Subset(array=w755, new element #1=w756, index #1=w758, new element #2=w756, index #2=w757, new element #3=w744, index #3=w745, new element #4=w733, index #4=w734, new element #5=w719, index #5=w720, new element #6=w717, index #6=w716, new element #7=w710, index #7=w711, new element #8=w708, index #8=w709) -> (w759:u16[])
            }
            frame "DispenseWater" {
              # "D"
              # "C"
              # "B"
              # "A"
              # "(A) Add COUNT and INCREMENT\n(B) Is (A) smaller than Tcycle?\n(C) Are we dispensing water or in the delay phase?\n(D) If (A) is smaller than Tcycle   AND   if we are dispensing water\n      then send TRUE to solenoid"
              # "delay"
              # "Tcycle"
              # "Solenoid__R"
              # "count"
              # "delay"
              # "Tcycle"
              # "Solenoid__L"
              # "count"
              n431 = To Unsigned Word Integer(number=w790) -> (unsigned 16bit integer=w772:u16)
              n432 = call "myRIO_BRig_RT_dataMTrig_Solenoid_delay__R.vi"() -> ("output_Solenoid_delay__R"=w776:i32)  [unwired: 11 in]
              n433 = call "myRIO_BRig_RT_dataMTrig_Solenoid_c__R.vi"() -> ("output_Solenoid_c__R"=w775:i32)  [unwired: 11 in]
              n434 = call "myRIO_BRig_RT_dataMTrig_Solenoid_Tcycle__R.vi"() -> ("output_Solenoid_Tcycle__R"=w777:i32)  [unwired: 11 in]
              n435 = call "myRIO_BRig_RT_dataMTrig_Solenoid_delay__L.vi"() -> ("output_Solenoid_delay__L"=w792:i32)  [unwired: 11 in]
              n436 = call "myRIO_BRig_RT_dataMTrig_Solenoid_c__L.vi"() -> ("output_Solenoid_c__L"=w784:i32)  [unwired: 11 in]
              n437 = call "myRIO_BRig_RT_dataMTrig_Solenoid_Tcycle__L.vi"() -> ("output_Solenoid_Tcycle__L"=w793:i32)  [unwired: 11 in]
              n438 = Index Array(array=w786, index #1=w784, index #2=w793, index #3=w792, index #4=w775, index #5=w777, index #6=w776) -> (element #1=w791:u16, element #2=w781:u16, element #3=w789:u16, element #4=w771:u16, element #5=w768:u16, element #6=w767:u16)
              n439 = Add(x=w791, y=w772) -> (x+y=w782:u16)
              n440 = Add(x=w771, y=w772) -> (x+y=w773:u16)
              n441 = Less?(x=w782, y=w781) -> (x < y?=w765:bool)
              n442 = Equal To 0?(x=w789) -> (x = 0?=w788:bool)
              n443 = Less?(x=w773, y=w768) -> (x < y?=w766:bool)
              n444 = Equal To 0?(x=w767) -> (x = 0?=w774:bool)
              n445 = And(x=w765, y=w788) -> (x .and. y?=w787:bool)
              n446 = Or(x=w765, y=w766) -> (x .or. y?=w764:bool)
              n447 = And(x=w766, y=w774) -> (x .and. y?=w769:bool)
              n448 = Select(t=w782, s=w765, f=w781) -> (s? t:f=w783:u16)
              n449 = Select(t=w773, s=w766, f=w768) -> (s? t:f=w770:u16)
              n450 = Replace Array Subset(array=w786, new element #1=w783, index #1=w784, new element #2=w770, index #2=w775) -> (w785:u16[])
              n451 = Select(t=w780, s=w764, f=myRIO_BRig_RT__Case_NonExp_stateList."DispenseWater_post" ("Enum")) -> (s? t:f=w778:T1)
            }
            frame "DispenseWater_post" {
              # "nCycle"
              # "delay"
              # "Solenoid__R"
              # "nCycle"
              # "delay"
              # "Solenoid__L"
              n452 = call "myRIO_BRig_RT_dataMTrig_Solenoid_N__L.vi"() -> ("output_Solenoid_N__L"=w815:i32)  [unwired: 11 in]
              n453 = call "myRIO_BRig_RT_dataMTrig_Solenoid_delay__L.vi"() -> ("output_Solenoid_delay__L"=w814:i32)  [unwired: 11 in]
              n454 = call "myRIO_BRig_RT_dataMTrig_Solenoid_N__R.vi"() -> ("output_Solenoid_N__R"=w811:i32)  [unwired: 11 in]
              n455 = call "myRIO_BRig_RT_dataMTrig_Solenoid_delay__R.vi"() -> ("output_Solenoid_delay__R"=w810:i32)  [unwired: 11 in]
              n456 = Index Array(array=w817, index #1=w815, index #2=w814, index #3=w811, index #4=w810) -> (element #1=w819:u16, element #2=w818:u16, element #3=w802:u16, element #4=w804:u16)
              n457 = Not Equal To 0?(x=w819) -> (x != 0?=w820:bool)
              n458 = Not Equal To 0?(x=w802) -> (x != 0?=w803:bool)
              n459 = case shown="True" w803 {
                selector: w803 -> [_ w828]
                tunnel: w802 -> [w826 w834]
                tunnel: w804 -> [_ w835]
                tunnel: [w826 w832] -> w801
                tunnel: [u16 0 w831] -> w800
                tunnel: [_ w828] -> w799
                frame False {
                }
                frame True {
                  n460 = Equal To 0?(x=w835) -> (x = 0?=w827:bool)
                  n461 = Decrement(x=w834) -> (x-1=w833:u16)
                  n462 = Select(t=w833, s=w827, f=w834) -> (s? t:f=w832:u16)
                  n463 = Select(t=u16 1, s=w827, f=u16 0) -> (s? t:f=w831:u16)
                }
              }
              n464 = case shown="True" w820 {
                selector: w820 -> [_ w839]
                tunnel: w819 -> [w837 w845]
                tunnel: w818 -> [_ w846]
                tunnel: [w837 w843] -> w813
                tunnel: [u16 0 w842] -> w812
                tunnel: [_ w839] -> w809
                frame False {
                }
                frame True {
                  n465 = Equal To 0?(x=w846) -> (x = 0?=w838:bool)
                  n466 = Decrement(x=w845) -> (x-1=w844:u16)
                  n467 = Select(t=w844, s=w838, f=w845) -> (s? t:f=w843:u16)
                  n468 = Select(t=u16 1, s=w838, f=u16 0) -> (s? t:f=w842:u16)
                }
              }
              n469 = Or(x=w809, y=w799) -> (x .or. y?=w808:bool)
              n470 = Replace Array Subset(array=w817, new element #1=w813, index #1=w815, new element #2=w812, index #2=w814, new element #3=w801, index #3=w811, new element #4=w800, index #4=w810) -> (w816:u16[])
              n471 = Select(t=myRIO_BRig_RT__Case_NonExp_stateList."DispenseWater_pre" ("Enum"), s=w808, f=myRIO_BRig_RT__Case_NonExp_stateList."Idle" ("Enum")) -> (s? t:f=w805:T1)
            }
            frame "TestConnection" {
              n472 = local read "Host Password"() -> (w857:string)
              n473 = local read "Host UserName"() -> (w858:string)
              n474 = call "myRIO_BRig_RT_comm_webdav_testConnect.vi"("input_password"=w857, "input_username"=w858) -> ("output_Iconnected"=w855:bool)  [unwired: 9 in]
              n475 = Select(t="Connection accepted!" ("message"), s=w855, f="Error!") -> (s? t:f=w853:string)
              n476 = One Button Dialog(message=w853) -> ()  [unwired: 1 in, 1 out]
            }
            frame "SendData" {
              n477 = local read "Host Filename Prefix"() -> (w860:string)
              n478 = local read "Host Password"() -> (w861:string)
              n479 = local read "Host UserName"() -> (w862:string)
              n480 = call "myRIO_BRig_RT_comm_webdav_sendData_all.vi"("Host Filename Prefix"=w860, "Host Password"=w861, "Host UserName"=w862) -> ()  [unwired: 9 in]
            }
            frame "End" {
            }
          }
          n481 = local read "MTrig_Audio_trig__R"() -> (w80:bool)
          n482 = local read "MTrig_Audio_trig__L"() -> (w79:bool)
          n483 = local read "START"() -> (w75:bool)
          n484 = local read "STOP_abort"() -> (w74:bool)
          n485 = local read "MTrig_Laser_trig"() -> (w81:bool)
          n486 = call "myRIO_BRig_RT_dataMTrig_main__v2.vi"("input_dataMTrig"=w83, "input_Audio_trig_L"=w79, "input_Audio_trig_R"=w80, "input_Laser_trig"=w81) -> ("output_dataMTrig"=w82:u16[], "output_Audio_L"=w59:bool, "output_Audio_R"=w70:bool, "output_Laser"=w62:bool)  [unwired: 12 in]
          n487 = Or(x=w75, y=w74) -> (x .or. y?=w73:bool)
          n488 = Select(t=myRIO_BRig_RT__Case_NonExp_stateList."End" ("Enum"), s=w73, f=w72) -> (s? t:f=w71:T1)
          n489 = Or(x=w80, y=w81) -> (x .or. y?=w78:bool)
          n490 = Or(x=w78, y=w79) -> (x .or. y?=w77:bool)
          n491 = case shown="True" w77 {
            frame False {
            }
            frame True {
              w108 = FALSE
              n492 = local write "MTrig_Audio_trig__R"(w108) -> ()
              n493 = local write "MTrig_Audio_trig__L"(w108) -> ()
              n494 = local write "MTrig_Laser_trig"(w108) -> ()
            }
          }
          n495 = xnode "Read/Write Control"("FPGA VI Reference In"=w100, "error in"=w98, "A1_SR"=w84, "A3_SL"=w85, "audioTrigger_L"=w59, "audioAmp_L"=w89, "audioFreq_L_Hz"=w88, "audioTrigger_R"=w70, "audioAmp_R"=w87, "audioFreq_R_Hz"=w86, "laserResponse_reward_LED"="laserResponse_reward_LED", "laserResponse_wrong_LED"="laserResponse_wrong_LED", "laserResponse_reward"="laserResponse_reward", "laserResponse_wrong"="laserResponse_wrong", "SelectionState"="SelectionState", "ignoreWrong"="ignoreWrong", "Left(F)_or_Right(T)"="Left(F)_or_Right(T)", "laserMTrig"=w62, "tCycle_laser_rew"="tCycle_laser_rew", "tDelay_laser_rew"="tDelay_laser_rew", "tCycle_laser_wro"="tCycle_laser_wro", "tDelay_laser_wro"="tDelay_laser_wro") -> ("FPGA VI Reference Out"=w99:refnum<k20>, "error out"=w97:errorcluster, "SelectReward"=→"SelectReward":bool, "SelectWrong"=→"SelectWrong":bool)
          n496 = node-c288() -> ()  [unwired: 1 in, 1 out]
          "cState_NonExp" <- w96
        }
        n497 = node-c288(w48) -> ()  [unwired: 1 out]
        n498 = flat-sequence {
          tunnel: w41 -> [w52]
          tunnel: [w52] -> w40
          tunnel: w39 -> [w51]
          tunnel: [w51] -> w38
          frame #0 {
            w50 = FALSE
            n499 = local write "STOP_endBlock"(w50) -> ()
            n500 = local write "STOP_endTrial"(w50) -> ()
          }
        }
      }
      frame True {
        w884 = FALSE ("SelectionState")
        w889 = u16 0 ("idxDataBlock")
        w891 = u16 100 ("new element/subarray")
        w892 = u16 100 ("new element/subarray")
        w912 = T6 refnum items=["Session NI_WebDAV"] ("output_hSession")
        w921 = FALSE
        w922 = u16 0
        w883 = FALSE
        # "audio__L\naudio__R"
        # "Audio params"
        # "nRewards"
        # "idxDataBlock"
        # "Solenoid_Tdelay_R"
        # "Solenoid_Tdelay_L"
        # "RewCalib_N__R"
        # "RewCalib_N__L"
        # "Save dataLick to file\nSend file to Host\nSave dataMTrig\nSend file to Host\nDisconnect"
        # "dataTrial"
        # "dataTrial"
        # "Solenoid_Tcycle_R"
        # "Solenoid_Tcycle_L"
        # "Laser_Tcycle"
        # "Audio_Tcycle_R"
        # "Audio_Tcycle_L"
        # "dataLick"
        # "dataLC"
        # "dataLC"
        # "dataBlock"
        # "dataBlock"
        # "dataMTrig"
        # "dataMTrig"
        # "dataExp"
        # "dataCurrent"
        # "dataExp"
        # "dataCurrent"
        # "spout"
        # "state"
        n501 = call "myRIO_BRig_RT_dataMTrig_Solenoid_Tcycle__L.vi"() -> ("output_Solenoid_Tcycle__L"=w918:i32)  [unwired: 11 in]
        n502 = call "myRIO_BRig_RT_dataMTrig_Solenoid_Tcycle__R.vi"() -> ("output_Solenoid_Tcycle__R"=w917:i32)  [unwired: 11 in]
        n503 = call "myRIO_BRig_RT_dataMTrig_Audio_Tcycle__L.vi"() -> ("output_Audio_Tcycle__L"=w916:i32)  [unwired: 11 in]
        n504 = call "myRIO_BRig_RT_dataMTrig_Audio_Tcycle__R.vi"() -> ("output_Audio_Tcycle__R"=w915:i32)  [unwired: 11 in]
        n505 = call "myRIO_BRig_RT_dataMTrig_Laser_Tcycle.vi"() -> ("output_Laser_Tcycle"=w914:i32)  [unwired: 11 in]
        n506 = local read "MTrig_Solenoid_Tcycle__L"() -> (w897:u16)
        n507 = local read "MTrig_Solenoid_Tcycle__R"() -> (w896:u16)
        n508 = local read "Tcycle_Reward_L"() -> (w893:u16)
        n509 = local read "Tcycle_Reward_R"() -> (w894:u16)
        n510 = local read "MTrig_Laser_Tcycle"() -> (w895:u16)
        n511 = call "myRIO_BRig_RT_dataMTrig_Solenoid_RewCalib_nCycle__L.vi"() -> ("output_Solenoid_RewCalib_nCycle__L"=w900:i32)  [unwired: 11 in]
        n512 = call "myRIO_BRig_RT_dataMTrig_Solenoid_Tdelay__L.vi"() -> ("output_Solenoid_Tdelay__L"=w902:i32)  [unwired: 11 in]
        n513 = call "myRIO_BRig_RT_dataMTrig_Solenoid_RewCalib_nCycle__R.vi"() -> ("output_Solenoid_RewCalib_nCycle__R"=w901:i32)  [unwired: 11 in]
        n514 = call "myRIO_BRig_RT_dataMTrig_Solenoid_Tdelay__R.vi"() -> ("output_Solenoid_Tdelay__R"=w903:i32)  [unwired: 11 in]
        n515 = call "myRIO_BRig_RT_dataLick_init.vi"() -> ("output_dataLick"=w924:u16[][])  [unwired: 11 in]
        n516 = call "myRIO_BRig_RT_dataCurrent_init.vi"() -> ("output_dataCurrent"=w931:u16[])  [unwired: 11 in]
        n517 = call "myRIO_BRig_RT_dataExp_init.vi"() -> ("output_dataExp"=w930:u16[])  [unwired: 11 in]
        n518 = call "myRIO_BRig_RT_dataMTrig_init.vi"() -> ("output_dataMTrig"=w920:u16[])  [unwired: 5 in]
        n519 = call "myRIO_BRig_RT_dataLC_init.vi"() -> ("output_dataLC"=w928:u16[])  [unwired: 11 in]
        n520 = call "myRIO_BRig_RT_dataBlock_init.vi"() -> ("output_dataBlock"=w929:u16[][])  [unwired: 11 in]
        n521 = call "myRIO_BRig_RT_dataTrial_init.vi"() -> ("output_dataTrial"=w913:u16[][])  [unwired: 11 in]
        n522 = xnode "Read/Write Control"("FPGA VI Reference In"=w885, "error in"=w886, "SelectionState"=w884, "laserResponse_reward"=w884, "laserResponse_wrong"=w884, "laserResponse_reward_LED"=w884, "laserResponse_wrong_LED"=w884, "Left(F)_or_Right(T)"=w884, "ignoreWrong"=w884, "SelectionState"=w884) -> ("FPGA VI Reference Out"=w887:refnum<k20>, "error out"=w888:errorcluster)
        n523 = Replace Array Subset(array=w920, new element #1=w892, index #1=w900, new element #2=w892, index #2=w901, new element #3=w891, index #3=w902, new element #4=w891, index #4=w903, new element #5=w897, index #5=w918, new element #6=w896, index #6=w917, new element #7=w893, index #7=w916, new element #8=w894, index #8=w915, new element #9=w895, index #9=w914) -> (w919:u16[])
        n524 = Get Date/Time In Seconds() -> (seconds since 1Jan1904=w899:timestamp)
        n525 = To Double Precision Float(number=w899) -> (double precision float=w898:dbl)
        n526 = node-c288() -> (w939:T3)  [unwired: 4 in]
        n527 = timed-loop {
          timing: w939 -> [_]
          timing-out: [_] -> w938
          shift-right: [w1017] -> _
          shift-left: myRIO_BRig_RT__Case_Exp_stateList."Start1" ("Enum") -> [w1048]
          shift-right: [w1069] -> _
          shift-left: enum16{"Left", "Right"}."Left" -> [w1071]
          tunnel: w887 -> [w1068]
          tunnel: w888 -> [w1067]
          shift-right: [w1062] -> _
          shift-left: w936 -> [w1066]
          shift-right: [w1061] -> _
          shift-left: w935 -> [w1065]
          tunnel: [w1042] -> w933
          tunnel: [w1043] -> w934
          shift-right: [w1044] -> w904
          shift-left: w931 -> [w1009]
          shift-right: [w1060] -> _
          shift-left: w930 -> [w1004]
          shift-right: [w1031] -> w908
          shift-left: w919 -> [w1032]
          shift-right: [w1058] -> _
          shift-left: w929 -> [w1059]
          shift-right: [w1056] -> _
          shift-left: w928 -> [w1057]
          shift-right: [w989] -> _
          shift-left: w883 -> [w1055]
          shift-right: [w1046] -> w910
          shift-left: w924 -> [w1047]
          shift-right: [w1033] -> _
          shift-left: w922 -> [w1041]
          shift-right: [w1001] -> _
          shift-left: w922 -> [w1040]
          shift-right: [w1034] -> _
          shift-left: w922 -> [w1039]
          shift-right: [w1035] -> _
          shift-left: w922 -> [w1038]
          shift-right: [w1002] -> _
          shift-left: w921 -> [w1036]
          shift-right: [w1003] -> _
          shift-left: w921 -> [w1037]
          shift-right: [w1015] -> _
          shift-left: w913 -> [w1016]
          shift-right: [w1014] -> w906
          shift-left: w912 -> [w1012]
          shift-right: [w1013] -> w907
          shift-left: FALSE ("output_Iconnected") -> [w1011]
          tunnel: "Host Filename Prefix" -> [w1010]
          tunnel: [w1010] -> w905
          shift-right: [w984] -> _
          shift-left: w883 -> [w1008]
          tunnel: w898 -> [w1005]
          shift-right: [w999] -> _
          shift-left: 0 ("idxDataBlock") -> [w1000]
          shift-right: [w996] -> _
          shift-left: w889 -> [w998]
          shift-right: [w995] -> _
          shift-left: w889 -> [w997]
          shift-right: [w983] -> _
          shift-left: w883 -> [w990]
          shift-right: [w986] -> _
          shift-left: w883 -> [w988]
          shift-right: [w985] -> _
          shift-left: w883 -> [w987]
          shift-right: [w976] -> _
          shift-left: w883 -> [w977]
          stop <- w1054 stop-if-true
          # "Laser"
          # "Audio R"
          # "Audio L"
          # "Solenoid R"
          # "Solenoid L"
          # "manual triggering"
          # "dataTrial"
          # "dataBlock"
          # "nRewards"
          # "laserOccurred"
          # "dataExp"
          # "dataCurrent"
          # "audio__L\naudio__R"
          # "time stamp"
          # "Audio params"
          # "nRewards"
          # "idxDataBlock"
          # "idxDataBlock"
          # "activate"
          # "audio__L\naudio__R"
          # "amp__R\nfreq__R"
          # "amp__L\nfreq__L"
          # "dataLC"
          # "solenoid__R"
          # "solenoid__L"
          # "Did a lick occur?"
          # "Update lick counter"
          # "spout"
          # "spout"
          # "state"
          # "state"
          n528 = node-c288() -> ()  [unwired: 1 in, 1 out]
          n529 = local read "MTrig_Solenoid_trig__L"() -> (w1029:bool)
          n530 = local read "MTrig_Solenoid_trig__R"() -> (w1028:bool)
          n531 = local read "MTrig_Audio_trig__L"() -> (w1027:bool)
          n532 = local read "MTrig_Audio_trig__R"() -> (w1026:bool)
          n533 = xnode "Read/Write Control"("FPGA VI Reference In"=w1068, "error in"=w1067) -> ("FPGA VI Reference Out"=w994:refnum<k20>, "error out"=w993:errorcluster, "A2_LickL"=w1062:u32, "A4_LickR"=w1061:u32)
          "A2" <- w1062
          "A4" <- w1061
          n534 = local read "MTrig_Laser_trig"() -> (w1025:bool)
          n535 = Greater?(x=w1062, y=w1066) -> (0:w1064:bool)
          n536 = Greater?(x=w1061, y=w1065) -> (0:w1063:bool)
          n537 = Or(x=w1064, y=w1063) -> (x .or. y?=w1070:bool)
          n538 = call "myRIO_BRig_RT_dataMTrig_main.vi"("input_dataMTrig"=w1032, "input_Solenoid_trig_L"=w1029, "input_Solenoid_trig_R"=w1028, "input_Audio_trig_L"=w1027, "input_Audio_trig_R"=w1026, "input_Laser_trig"=w1025) -> ("output_Laser"=w981:bool, "output_dataMTrig"=w1031:u16[], "output_Solenoid_L"=w1019:bool, "output_Solenoid_R"=w1021:bool, "output_Audio_L"=w1023:bool, "output_Audio_R"=w1024:bool)  [unwired: 8 in]
          n539 = Compound Arithmetic op=OR(w1029, w1028, w1027, w1026, w1025) -> (w1030:bool)
          n540 = case shown="True" w1030 {
            frame False {
            }
            frame True {
              w1072 = FALSE
              n541 = local write "MTrig_Solenoid_trig__L"(w1072) -> ()
              n542 = local write "MTrig_Solenoid_trig__R"(w1072) -> ()
              n543 = local write "MTrig_Audio_trig__L"(w1072) -> ()
              n544 = local write "MTrig_Audio_trig__R"(w1072) -> ()
              n545 = local write "MTrig_Laser_trig"(w1072) -> ()
            }
          }
          n546 = case shown="\"initTrial4\"" w1048 {
            selector: w1048 -> [_ _ _ _ _ _ _ _ _ _ _ _ _ _ _ _ _ _ _ _ w1771 _ w1836 _ _ _ _ _ w1978 _ w2053 _ _ _ _ _ w2185 _ w2262 _ w2326 _ w2370 _ _ w2437 _ _ _ _ _ w2605 _ _ _ _ _ _ _ _ _ _ _ _ _ _ _ _ _ _ _]
            tunnel: [myRIO_BRig_RT__Case_Exp_stateList."Start2" ("Enum") myRIO_BRig_RT__Case_Exp_stateList."Start3" ("Enum") myRIO_BRig_RT__Case_Exp_stateList."saveSettings1" ("Enum") myRIO_BRig_RT__Case_Exp_stateList."saveSettings2" ("Enum") myRIO_BRig_RT__Case_Exp_stateList."saveSettings3" ("Enum") myRIO_BRig_RT__Case_Exp_stateList."saveSettings4_LC_ENL" ("Enum") myRIO_BRig_RT__Case_Exp_stateList."saveSettings5_LC_Cue" ("Enum") myRIO_BRig_RT__Case_Exp_stateList."saveSettings6_LC_Other" ("Enum") myRIO_BRig_RT__Case_Exp_stateList."setSettings_Audio" ("Enum") myRIO_BRig_RT__Case_Exp_stateList."setSettings_Laser" ("Enum") myRIO_BRig_RT__Case_Exp_stateList."commConnect" ("Enum") w1543 myRIO_BRig_RT__Case_Exp_stateList."initTrial" ("Enum") w1583 myRIO_BRig_RT__Case_Exp_stateList."initTrial3" ("Enum") myRIO_BRig_RT__Case_Exp_stateList."initTrial_LC_ENL1" ("Enum") myRIO_BRig_RT__Case_Exp_stateList."ENL1_pre" ("Enum") myRIO_BRig_RT__Case_Exp_stateList."initTrial_LC_Cue1" ("Enum") myRIO_BRig_RT__Case_Exp_stateList."initTrial4" ("Enum") w1730 w1768 myRIO_BRig_RT__Case_Exp_stateList."ENL1Penalty" ("Enum") w1837 myRIO_BRig_RT__Case_Exp_stateList."endExp" ("Enum") myRIO_BRig_RT__Case_Exp_stateList."endExp" ("Enum") myRIO_BRig_RT__Case_Exp_stateList."endExp" ("Enum") myRIO_BRig_RT__Case_Exp_stateList."endExp" ("Enum") w1932 w1977 myRIO_BRig_RT__Case_Exp_stateList."Cue1Penalty" ("Enum") w2051 myRIO_BRig_RT__Case_Exp_stateList."endExp" ("Enum") myRIO_BRig_RT__Case_Exp_stateList."endExp" ("Enum") myRIO_BRig_RT__Case_Exp_stateList."endExp" ("Enum") myRIO_BRig_RT__Case_Exp_stateList."endExp" ("Enum") w2139 w2193 myRIO_BRig_RT__Case_Exp_stateList."SelectReward" ("Enum") w2263 myRIO_BRig_RT__Case_Exp_stateList."SelectRewardPost" ("Enum") w2327 myRIO_BRig_RT__Case_Exp_stateList."SelectWrong" ("Enum") w2366 myRIO_BRig_RT__Case_Exp_stateList."endTrial1" ("Enum") myRIO_BRig_RT__Case_Exp_stateList."SelectTimeout" ("Enum") w2439 myRIO_BRig_RT__Case_Exp_stateList."endTrial1" ("Enum") myRIO_BRig_RT__Case_Exp_stateList."endTrial2" ("Enum") myRIO_BRig_RT__Case_Exp_stateList."saveData_dataBlock" ("Enum") w2518 w2588 w2605 myRIO_BRig_RT__Case_Exp_stateList."initBlock" ("Enum") w2632 myRIO_BRig_RT__Case_Exp_stateList."commUpload_dataCurrent" ("Enum") myRIO_BRig_RT__Case_Exp_stateList."commUpload_dataExp" ("Enum") myRIO_BRig_RT__Case_Exp_stateList."commUpload_dataLC" ("Enum") myRIO_BRig_RT__Case_Exp_stateList."commUpload_dataTrial" ("Enum") myRIO_BRig_RT__Case_Exp_stateList."endTrial3" ("Enum") myRIO_BRig_RT__Case_Exp_stateList."saveData_dataCurrent" ("Enum") myRIO_BRig_RT__Case_Exp_stateList."saveData_dataExp" ("Enum") myRIO_BRig_RT__Case_Exp_stateList."saveData_dataLC" ("Enum") myRIO_BRig_RT__Case_Exp_stateList."saveData_dataTrial" ("Enum") myRIO_BRig_RT__Case_Exp_stateList."commUpload_pre" ("Enum") myRIO_BRig_RT__Case_Exp_stateList."empty_endBlock2" ("Enum") myRIO_BRig_RT__Case_Exp_stateList."initBlock" ("Enum") myRIO_BRig_RT__Case_Exp_stateList."empty_endTrial2" ("Enum") myRIO_BRig_RT__Case_Exp_stateList."empty_endTrial3" ("Enum") myRIO_BRig_RT__Case_Exp_stateList."empty_endTrial4" ("Enum") myRIO_BRig_RT__Case_Exp_stateList."empty_endTrial5" ("Enum") myRIO_BRig_RT__Case_Exp_stateList."initTrial" ("Enum")] -> w1017
            tunnel: [w1098 w1117 w1139 w1196 w1240 w1297 w1349 w1401 w1445 w1469 w1515 w1519 w1551 w1584 w1607 w1629 w1655 w1680 w1705 w1746 w1784 w1814 w1841 w1857 w1879 w1898 w1917 w1951 w1999 w2024 w2050 w2071 w2092 w2111 w2130 w2150 w2211 w2236 w2259 w2274 w2324 w2348 w2381 w2402 w2418 w2450 w2473 w2485 w2504 w2542 w2561 w2604 w2621 w2635 w2669 w2690 w2711 w2732 w2753 w2781 w2801 w2828 w2848 w2873 w2892 w2911 w2930 w2949 w2968 w2987 w3006] -> w1069
            tunnel: w1071 -> [w1098 w1117 w1139 w1196 w1240 w1297 w1349 w1401 w1445 w1469 w1515 w1542 w1551 w1584 w1607 w1629 w1655 w1680 w1705 w1746 w1784 w1814 w1841 w1857 w1879 w1898 w1917 w1951 w1999 w2024 w2050 w2071 w2092 w2111 w2130 w2150 w2211 w2236 w2259 w2274 w2324 w2348 w2381 w2402 w2418 w2450 w2473 w2485 w2504 w2542 w2561 w2604 w2621 w2635 w2669 w2690 w2711 w2732 w2753 w2781 w2801 w2828 w2848 w2873 w2892 w2911 w2930 w2949 w2968 w2987 w3006]
            tunnel: w1070 -> [w1101 w1120 w1136 w1199 w1243 w1300 w1352 w1404 w1448 w1472 w1518 w1536 w1562 w1585 w1625 w1646 w1670 w1693 w1718 w1733 w1765 w1817 w1844 w1863 w1882 w1901 w1920 w1931 w1976 w2032 w2057 w2076 w2095 w2114 w2133 w2148 w2209 w2246 w2270 w2305 w2332 w2359 w2384 w2401 w2430 w2455 w2470 w2493 w2503 w2553 w2587 w2608 w2618 w2644 w2672 w2693 w2714 w2735 w2756 w2784 w2804 w2831 w2851 w2876 w2895 w2914 w2933 w2952 w2971 w2990 w3009]
            tunnel: w1064 -> [w1100 w1119 w1137 w1198 w1242 w1299 w1351 w1403 w1447 w1471 w1517 w1535 w1561 w1586 w1624 w1647 w1671 w1694 w1719 w1756 w1786 w1816 w1843 w1862 w1881 w1900 w1919 w1965 w2000 w2031 w2056 w2075 w2094 w2113 w2132 w2149 w2208 w2245 w2269 w2304 w2331 w2358 w2383 w2400 w2429 w2454 w2471 w2494 w2502 w2552 w2586 w2607 w2619 w2645 w2671 w2692 w2713 w2734 w2755 w2783 w2803 w2830 w2850 w2875 w2894 w2913 w2932 w2951 w2970 w2989 w3008]
            tunnel: w1063 -> [w1099 w1118 w1138 w1197 w1241 w1298 w1350 w1402 w1446 w1470 w1516 w1534 w1560 w1587 w1623 w1648 w1672 w1695 w1720 w1755 w1785 w1815 w1842 w1861 w1880 w1899 w1918 w1964 w2001 w2030 w2055 w2074 w2093 w2112 w2131 w2168 w2212 w2244 w2268 w2303 w2330 w2357 w2382 w2399 w2428 w2453 w2472 w2495 w2501 w2551 w2585 w2606 w2620 w2646 w2670 w2691 w2712 w2733 w2754 w2782 w2802 w2829 w2849 w2874 w2893 w2912 w2931 w2950 w2969 w2988 w3007]
            tunnel: [w1101 w1120 w1136 w1199 w1243 w1300 w1352 w1404 w1448 w1472 w1518 w1536 w1562 w1585 w1625 w1646 w1670 w1693 w1718 w1733 w1765 w1817 w1844 w1863 w1882 w1901 w1920 w1931 w1976 w2032 w2057 w2076 w2095 w2114 w2133 w2148 w2209 w2246 w2270 w2305 w2332 w2359 w2384 w2401 w2430 w2455 w2470 w2493 w2503 w2553 w2587 w2608 w2618 w2644 w2672 w2693 w2714 w2735 w2756 w2784 w2804 w2831 w2851 w2876 w2895 w2914 w2933 w2952 w2971 w2990 w3009] -> w1051
            tunnel: [w1100 w1119 w1137 w1198 w1242 w1299 w1351 w1403 w1447 w1471 w1517 w1535 w1561 w1586 w1624 w1647 w1671 w1694 w1719 w1756 w1786 w1816 w1843 w1862 w1881 w1900 w1919 w1965 w2000 w2031 w2056 w2075 w2094 w2113 w2132 w2149 w2208 w2245 w2269 w2304 w2331 w2358 w2383 w2400 w2429 w2454 w2471 w2494 w2502 w2552 w2586 w2607 w2619 w2645 w2671 w2692 w2713 w2734 w2755 w2783 w2803 w2830 w2850 w2875 w2894 w2913 w2932 w2951 w2970 w2989 w3008] -> w1050
            tunnel: [w1099 w1118 w1138 w1197 w1241 w1298 w1350 w1402 w1446 w1470 w1516 w1534 w1560 w1587 w1623 w1648 w1672 w1695 w1720 w1755 w1785 w1815 w1842 w1861 w1880 w1899 w1918 w1964 w2001 w2030 w2055 w2074 w2093 w2112 w2131 w2168 w2212 w2244 w2268 w2303 w2330 w2357 w2382 w2399 w2428 w2453 w2472 w2495 w2501 w2551 w2585 w2606 w2620 w2646 w2670 w2691 w2712 w2733 w2754 w2782 w2802 w2829 w2849 w2874 w2893 w2912 w2931 w2950 w2969 w2988 w3007] -> w1049
            tunnel: w1009 -> [w1097 w1116 w1135 w1157 w1216 w1274 w1348 w1400 w1444 w1467 w1496 w1541 w1550 w1582 w1596 w1630 w1656 w1677 w1704 w1745 w1770 w1808 w1840 w1858 w1878 w1897 w1916 w1935 w1996 w2023 w2054 w2072 w2091 w2110 w2129 w2159 w2189 w2228 w2265 w2276 w2329 w2349 w2380 w2398 w2419 w2452 w2469 w2482 w2506 w2522 w2559 w2603 w2622 w2647 w2666 w2687 w2708 w2729 w2740 w2770 w2789 w2813 w2845 w2862 w2882 w2901 w2920 w2939 w2958 w2977 w2996]
            tunnel: w1004 -> [w1096 w1115 w1134 w1194 w1238 w1294 w1346 w1398 w1442 w1460 w1511 w1540 w1559 w1581 w1604 w1634 w1658 w1683 w1708 w1748 w1783 w1807 w1838 w1860 w1877 w1896 w1915 w1953 w1998 w2021 w2049 w2073 w2090 w2109 w2128 w2161 w2210 w2242 w2267 w2297 w2325 w2350 w2378 w2397 w2421 w2449 w2468 w2492 w2509 w2521 w2578 w2602 w2623 w2648 w2665 w2686 w2707 w2728 w2741 w2778 w2798 w2809 w2844 w2870 w2889 w2908 w2927 w2946 w2965 w2984 w3003]
            tunnel: [w1097 w1116 w1135 w1157 w1216 w1273 w1348 w1400 w1444 w1467 w1495 w1525 w1550 w1570 w1596 w1630 w1656 w1676 w1703 w1749 w1769 w1809 w1839 w1858 w1878 w1897 w1916 w1960 w1995 w2022 w2052 w2072 w2091 w2110 w2129 w2162 w2184 w2243 w2264 w2298 w2328 w2351 w2379 w2398 w2422 w2451 w2469 w2481 w2505 w2522 w2557 w2603 w2622 w2647 w2666 w2687 w2708 w2729 w2740 w2770 w2789 w2813 w2845 w2862 w2882 w2901 w2920 w2939 w2958 w2977 w2996] -> w1045
            tunnel: [w1096 w1115 w1134 w1193 w1237 w1289 w1346 w1398 w1442 w1460 w1511 w1539 w1559 w1580 w1604 w1634 w1658 w1683 w1708 w1748 w1783 w1807 w1838 w1860 w1877 w1896 w1915 w1953 w1998 w2021 w2049 w2073 w2090 w2109 w2128 w2161 w2210 w2242 w2267 w2297 w2325 w2350 w2378 w2397 w2421 w2449 w2468 w2492 w2509 w2521 w2578 w2602 w2623 w2648 w2665 w2686 w2707 w2728 w2741 w2778 w2798 w2812 w2844 w2870 w2889 w2908 w2927 w2946 w2965 w2984 w3003] -> w1060
            tunnel: [_ _ _ _ _ _ _ _ _ _ _ _ _ _ _ _ _ _ _ _ _ _ _ _ _ _ _ _ _ _ _ _ _ _ _ _ _ _ w2257 _ _ _ _ _ _ _ _ _ _ _ _ _ _ _ _ _ _ _ _ _ _ _ _ _ _ _ _ _ _ _ _] -> w1020
            tunnel: [_ _ _ _ _ _ _ _ _ _ _ _ _ _ _ _ _ _ _ _ _ _ _ _ _ _ _ _ _ _ _ _ _ _ _ _ _ _ w2258 _ _ _ _ _ _ _ _ _ _ _ _ _ _ _ _ _ _ _ _ _ _ _ _ _ _ _ _ _ _ _ _] -> w1022
            tunnel: w1059 -> [w1094 w1113 w1132 w1159 w1218 w1295 w1347 w1399 w1443 w1465 w1512 w1537 w1552 w1578 w1616 w1644 w1668 w1673 w1700 w1747 w1782 w1804 w1834 w1859 w1875 w1894 w1913 w1959 w1997 w2020 w2047 w2069 w2088 w2107 w2126 w2160 w2206 w2234 w2266 w2278 w2322 w2347 w2375 w2395 w2420 w2448 w2466 w2484 w2511 w2549 w2570 w2600 w2625 w2650 w2663 w2684 w2705 w2726 w2750 w2764 w2791 w2819 w2838 w2864 w2883 w2902 w2921 w2940 w2959 w2978 w2997]
            tunnel: [w1094 w1113 w1132 w1159 w1218 w1295 w1347 w1399 w1443 w1465 w1512 w1537 w1549 w1578 w1616 w1644 w1668 w1673 w1700 w1747 w1782 w1804 w1834 w1859 w1875 w1894 w1913 w1959 w1997 w2020 w2047 w2069 w2088 w2107 w2126 w2160 w2206 w2234 w2266 w2277 w2322 w2347 w2375 w2395 w2420 w2448 w2466 w2483 w2511 w2549 w2570 w2600 w2625 w2650 w2663 w2684 w2705 w2726 w2750 w2764 w2791 w2819 w2838 w2864 w2883 w2902 w2921 w2940 w2959 w2978 w2997] -> w1058
            tunnel: w1057 -> [w1095 w1114 w1133 w1158 w1217 w1296 w1344 w1396 w1440 w1466 w1513 w1538 w1558 w1579 w1593 w1645 w1669 w1681 w1706 w1744 w1764 w1805 w1835 w1856 w1876 w1895 w1914 w1958 w1975 w2019 w2048 w2070 w2089 w2108 w2127 w2158 w2207 w2235 w2261 w2295 w2323 w2346 w2377 w2396 w2417 w2446 w2467 w2491 w2510 w2550 w2577 w2601 w2624 w2649 w2664 w2685 w2706 w2727 w2751 w2777 w2797 w2825 w2836 w2869 w2888 w2907 w2926 w2945 w2964 w2983 w3002]
            tunnel: [w1095 w1114 w1133 w1158 w1217 w1296 w1345 w1397 w1441 w1466 w1513 w1538 w1558 w1579 w1593 w1645 w1669 w1681 w1706 w1744 w1764 w1805 w1835 w1856 w1876 w1895 w1914 w1958 w1975 w2019 w2048 w2070 w2089 w2108 w2127 w2158 w2207 w2235 w2261 w2295 w2323 w2346 w2377 w2396 w2417 w2446 w2467 w2491 w2510 w2550 w2577 w2601 w2624 w2649 w2664 w2685 w2706 w2727 w2751 w2777 w2797 w2825 w2836 w2869 w2888 w2907 w2926 w2945 w2964 w2983 w3002] -> w1056
            tunnel: w1055 -> [_ _ _ _ _ _ _ _ _ _ _ _ _ _ _ _ _ _ _ w1729 w1757 w1790 w1823 _ _ _ _ _ w1969 w2006 _ _ _ _ _ _ _ _ w2260 _ _ _ w2376 _ _ w2447 _ _ _ _ _ _ _ _ _ _ _ _ _ _ _ _ _ _ _ _ _ _ _ _ _]
            tunnel: [_ _ _ _ _ _ _ _ _ _ _ _ _ _ _ _ _ _ _ _ _ _ _ _ _ _ _ _ _ _ _ _ _ _ _ _ _ _ _ _ _ _ _ _ _ _ _ _ _ _ _ TRUE _ _ _ _ _ _ _ _ _ _ _ _ _ _ _ _ _ _ _] -> w1052
            tunnel: w1041 -> [w1092 w1111 w1130 w1149 w1211 w1284 w1331 w1383 w1412 _ w1503 w1533 w1557 w1577 w1615 w1643 w1667 w1692 w1717 w1743 w1781 w1802 w1833 w1854 w1873 w1892 w1911 w1957 w1992 w2017 w2046 w2067 w2086 w2105 w2124 w2157 w2205 w2224 w2256 w2293 w2321 w2344 w2374 w2394 w2415 w2445 w2465 w2489 w2515 w2548 w2574 w2598 w2616 w2643 w2661 w2682 w2703 w2724 w2748 w2775 w2795 w2823 w2842 w2868 w2887 w2906 w2925 w2944 w2963 w2982 w3001]
            tunnel: w1040 -> [w1091 w1110 w1129 w1148 w1210 w1283 w1330 w1382 w1413 _ w1502 w1532 w1556 w1576 w1614 w1642 w1666 w1691 w1716 w1742 w1780 w1801 w1832 w1853 w1872 w1891 w1910 w1956 w1991 w2016 w2045 w2066 w2085 w2104 w2123 w2156 w2204 w2223 w2255 w2292 w2320 w2343 w2373 w2393 w2414 w2444 w2464 w2488 w2514 w2547 w2573 w2597 w2615 w2642 w2660 w2681 w2702 w2723 w2747 w2774 w2794 w2822 w2841 w2867 w2886 w2905 w2924 w2943 w2962 w2981 w3000]
            tunnel: w1039 -> [w1090 w1109 w1128 w1147 w1209 w1282 w1329 w1381 w1414 _ w1501 w1531 w1555 w1575 w1613 w1641 w1665 w1690 w1715 w1741 w1779 w1800 w1831 w1852 w1871 w1890 w1909 w1955 w1990 w2015 w2044 w2065 w2084 w2103 w2122 w2155 w2203 w2222 w2254 w2291 w2319 w2342 w2372 w2392 w2413 w2443 w2463 w2487 w2513 w2546 w2572 w2596 w2614 w2641 w2659 w2680 w2701 w2722 w2746 w2773 w2793 w2821 w2840 w2866 w2885 w2904 w2923 w2942 w2961 w2980 w2999]
            tunnel: w1038 -> [w1089 w1108 w1127 w1146 w1208 w1281 w1328 w1380 w1415 _ w1500 w1530 w1554 w1574 w1612 w1640 w1664 w1689 w1714 w1740 w1778 w1799 w1830 w1851 w1870 w1889 w1908 w1954 w1989 w2014 w2043 w2064 w2083 w2102 w2121 w2154 w2202 w2221 w2253 w2290 w2318 w2341 w2371 w2391 w2412 w2442 w2462 w2486 w2512 w2545 w2571 w2595 w2613 w2640 w2658 w2679 w2700 w2721 w2745 w2772 w2792 w2820 w2839 w2865 w2884 w2903 w2922 w2941 w2960 w2979 w2998]
            tunnel: w1037 -> [_ _ _ _ _ _ _ _ _ _ _ _ _ _ _ _ _ _ _ _ _ _ _ _ _ _ _ _ w1994 _ _ _ _ _ _ _ _ _ _ _ _ _ _ _ _ _ _ _ _ _ _ _ _ _ _ _ _ _ _ _ _ _ _ _ _ _ _ _ _ _ _]
            tunnel: w1036 -> [_ _ _ _ _ _ _ _ _ _ _ _ _ _ _ _ _ _ _ _ _ _ _ _ _ _ _ _ w1993 _ _ _ _ _ _ _ _ _ _ _ _ _ _ _ _ _ _ _ _ _ _ _ _ _ _ _ _ _ _ _ _ _ _ _ _ _ _ _ _ _ _]
            tunnel: [w1092 w1111 w1130 w1149 w1211 w1284 w1331 w1383 w1412 w1459 w1503 w1533 w1557 w1577 w1615 w1643 w1667 w1692 w1717 w1743 w1781 w1802 w1833 w1854 w1873 w1892 w1911 w1957 w1992 w2017 w2046 w2067 w2086 w2105 w2124 w2157 w2205 w2224 w2256 w2293 w2321 w2344 w2374 w2394 w2415 w2445 w2465 w2489 w2515 w2548 w2574 w2598 w2616 w2643 w2661 w2682 w2703 w2724 w2748 w2775 w2795 w2823 w2842 w2868 w2887 w2906 w2925 w2944 w2963 w2982 w3001] -> w1033
            tunnel: [w1091 w1110 w1129 w1148 w1210 w1283 w1330 w1382 w1413 w1458 w1502 w1532 w1556 w1576 w1614 w1642 w1666 w1691 w1716 w1742 w1780 w1801 w1832 w1853 w1872 w1891 w1910 w1956 w1991 w2016 w2045 w2066 w2085 w2104 w2123 w2156 w2204 w2223 w2255 w2292 w2320 w2343 w2373 w2393 w2414 w2444 w2464 w2488 w2514 w2547 w2573 w2597 w2615 w2642 w2660 w2681 w2702 w2723 w2747 w2774 w2794 w2822 w2841 w2867 w2886 w2905 w2924 w2943 w2962 w2981 w3000] -> w1001
            tunnel: [w1090 w1109 w1128 w1147 w1209 w1282 w1329 w1381 w1414 w1457 w1501 w1531 w1555 w1575 w1613 w1641 w1665 w1690 w1715 w1741 w1779 w1800 w1831 w1852 w1871 w1890 w1909 w1955 w1990 w2015 w2044 w2065 w2084 w2103 w2122 w2155 w2203 w2222 w2254 w2291 w2319 w2342 w2372 w2392 w2413 w2443 w2463 w2487 w2513 w2546 w2572 w2596 w2614 w2641 w2659 w2680 w2701 w2722 w2746 w2773 w2793 w2821 w2840 w2866 w2885 w2904 w2923 w2942 w2961 w2980 w2999] -> w1034
            tunnel: [w1089 w1108 w1127 w1146 w1208 w1281 w1328 w1380 w1415 w1456 w1500 w1530 w1554 w1574 w1612 w1640 w1664 w1689 w1714 w1740 w1778 w1799 w1830 w1851 w1870 w1889 w1908 w1954 w1989 w2014 w2043 w2064 w2083 w2102 w2121 w2154 w2202 w2221 w2253 w2290 w2318 w2341 w2371 w2391 w2412 w2442 w2462 w2486 w2512 w2545 w2571 w2595 w2613 w2640 w2658 w2679 w2700 w2721 w2745 w2772 w2792 w2820 w2839 w2865 w2884 w2903 w2922 w2941 w2960 w2979 w2998] -> w1035
            tunnel: [_ _ _ _ _ _ _ _ _ _ _ _ _ _ _ _ _ _ _ _ _ _ _ _ _ _ _ w1944 w1994 _ _ _ _ _ _ _ _ _ _ _ _ _ _ _ _ _ _ _ _ _ _ _ _ _ _ _ _ _ _ _ _ _ _ _ _ _ _ _ _ _ _] -> w1003
            tunnel: [_ _ _ _ _ _ _ _ _ _ _ _ _ _ _ _ _ _ _ _ _ _ _ _ _ _ _ w1943 w1993 _ _ _ _ _ _ _ _ _ _ _ _ _ _ _ _ _ _ _ _ _ _ _ _ _ _ _ _ _ _ _ _ _ _ _ _ _ _ _ _ _ _] -> w1002
            tunnel: w1016 -> [w1088 w1107 w1126 w1145 w1207 w1280 w1327 w1379 w1411 w1455 w1510 w1529 w1553 w1573 w1598 w1632 w1653 w1675 w1702 w1739 w1777 w1798 w1829 w1850 w1869 w1888 w1907 w1942 w1988 w2013 w2042 w2063 w2082 w2101 w2120 w2153 w2201 w2218 w2252 w2289 w2317 w2338 w2365 w2390 w2409 w2436 w2461 w2480 w2508 w2538 w2569 w2594 w2626 w2651 w2662 w2683 w2704 w2725 w2749 w2776 w2796 w2824 w2843 w2859 w2881 w2900 w2919 w2938 w2957 w2976 w2995]
            tunnel: [w1088 w1107 w1126 w1145 w1207 w1280 w1327 w1379 w1411 w1455 w1510 w1529 w1553 w1573 w1597 w1631 w1653 w1674 w1701 w1739 w1777 w1798 w1829 w1850 w1869 w1888 w1907 w1942 w1988 w2013 w2042 w2063 w2082 w2101 w2120 w2153 w2201 w2218 w2252 w2289 w2317 w2338 w2365 w2390 w2409 w2436 w2461 w2480 w2507 w2538 w2569 w2594 w2626 w2651 w2662 w2683 w2704 w2725 w2749 w2776 w2796 w2824 w2843 w2859 w2881 w2900 w2919 w2938 w2957 w2976 w2995] -> w1015
            tunnel: [w1087 w1106 w1125 w1144 w1206 w1279 w1326 w1378 w1410 w1454 w1509 w1528 w1564 w1572 w1618 w1639 w1663 w1688 w1713 w1738 w1776 w1797 w1828 w1849 w1868 w1887 w1906 w1941 w1987 w2012 w2041 w2062 w2081 w2100 w2119 w2152 w2200 w2217 w2251 w2288 w2316 w2337 w2364 w2389 w2408 w2435 w2460 w2479 w2500 w2544 w2568 w2592 w2627 w2637 w2657 w2678 w2699 w2720 w2744 w2780 w2800 w2827 w2847 w2872 w2891 w2910 w2929 w2948 w2967 w2986 w3005] -> w1014
            tunnel: [w1086 w1105 w1124 w1143 w1205 w1278 w1325 w1377 w1409 w1453 w1508 w1527 w1563 w1571 w1617 w1638 w1662 w1687 w1712 w1737 w1775 w1796 w1827 w1848 w1867 w1886 w1905 w1940 w1986 w2011 w2040 w2061 w2080 w2099 w2118 w2151 w2199 w2216 w2250 w2287 w2315 w2336 w2363 w2388 w2407 w2434 w2459 w2478 w2499 w2543 w2567 w2593 w2609 w2634 w2667 w2688 w2709 w2730 w2752 w2779 w2799 w2826 w2846 w2871 w2890 w2909 w2928 w2947 w2966 w2985 w3004] -> w1013
            tunnel: w1012 -> [w1087 w1106 w1125 w1144 w1206 w1279 w1326 w1378 w1410 w1454 w1509 w1528 w1564 w1572 w1618 w1639 w1663 w1688 w1713 w1738 w1776 w1797 w1828 w1849 w1868 w1887 w1906 w1941 w1987 w2012 w2041 w2062 w2081 w2100 w2119 w2152 w2200 w2217 w2251 w2288 w2316 w2337 w2364 w2389 w2408 w2435 w2460 w2479 w2500 w2544 w2568 w2592 _ w2637 w2657 w2678 w2699 w2720 w2744 w2780 w2800 w2827 w2847 w2872 w2891 w2910 w2929 w2948 w2967 w2986 w3005]
            tunnel: w1011 -> [w1086 w1105 w1124 w1143 w1205 w1278 w1325 w1377 w1409 w1453 w1508 w1527 w1563 w1571 w1617 w1638 w1662 w1687 w1712 w1737 w1775 w1796 w1827 w1848 w1867 w1886 w1905 w1940 w1986 w2011 w2040 w2061 w2080 w2099 w2118 w2151 w2199 w2216 w2250 w2287 w2315 w2336 w2363 w2388 w2407 w2434 w2459 w2478 w2499 w2543 w2567 w2593 _ w2634 w2667 w2688 w2709 w2730 w2752 w2779 w2799 w2826 w2846 w2871 w2890 w2909 w2928 w2947 w2966 w2985 w3004]
            tunnel: w1010 -> [_ _ _ _ _ _ _ _ _ _ _ _ _ _ _ _ _ _ _ _ _ _ _ _ _ _ _ _ _ _ _ _ _ _ _ _ _ _ _ _ _ _ _ _ _ _ _ _ _ _ _ _ _ _ w2655 w2676 w2697 w2718 w2742 _ _ _ _ _ _ _ _ _ _ _ _]
            tunnel: w1008 -> [_ _ _ _ _ _ _ _ _ _ _ _ _ _ _ _ w1652 _ w1697 w1726 w1762 w1788 w1819 _ _ _ _ w1922 w1967 w2005 w2034 _ _ _ _ _ _ _ _ _ _ _ _ _ _ _ _ _ _ _ _ _ _ _ _ _ _ _ _ _ _ _ _ _ _ _ _ _ _ _ _]
            tunnel: [_ _ _ _ _ _ _ _ _ _ _ _ _ _ _ TRUE TRUE _ _ _ _ _ _ _ _ _ _ _ _ _ _ _ _ _ _ _ _ _ _ _ _ _ _ _ _ _ _ _ _ _ _ _ _ _ _ _ _ _ _ _ _ _ _ _ _ _ _ _ _ _ _] -> w991
            tunnel: w1005 -> [_ _ _ _ _ _ _ _ _ _ _ _ _ _ _ _ _ _ _ _ _ _ _ _ _ _ _ _ _ _ _ _ _ _ _ _ _ _ _ _ _ _ _ _ _ _ _ _ _ _ _ _ _ _ _ _ _ _ _ _ _ w2814 _ _ _ _ _ _ _ _ _]
            tunnel: [w1085 w1104 w1123 w1142 w1204 w1277 w1324 w1376 w1408 w1452 w1507 w1522 w1547 w1567 w1619 w1637 w1661 w1686 w1711 w1736 w1774 w1795 w1826 w1847 w1866 w1885 w1904 w1939 w1985 w2010 w2039 w2060 w2079 w2098 w2117 w2147 w2198 w2215 w2249 w2272 w2314 w2335 w2362 w2387 w2406 w2433 w2458 w2477 w2498 w2541 w2554 w2591 w2612 w2636 w2654 w2675 w2696 w2717 w2739 w2759 w2788 w2808 w2835 w2855 w2880 w2899 w2918 w2937 w2956 w2975 w2994] -> w999
            tunnel: w1000 -> [w1085 w1104 w1123 w1142 w1204 w1277 w1324 w1376 w1408 w1452 w1507 w1522 _ w1567 w1619 w1637 w1661 w1686 w1711 w1736 w1774 w1795 w1826 w1847 w1866 w1885 w1904 w1939 w1985 w2010 w2039 w2060 w2079 w2098 w2117 w2147 w2198 w2215 w2249 w2272 w2314 w2335 w2362 w2387 w2406 w2433 w2458 w2477 w2498 w2541 w2555 w2591 w2612 w2636 w2654 w2675 w2696 w2717 w2739 w2759 w2788 w2808 w2835 w2855 w2880 w2899 w2918 w2937 w2956 w2975 w2994]
            tunnel: w998 -> [w1084 w1103 w1122 w1141 w1203 w1276 w1323 w1375 w1407 w1451 w1506 w1521 w1546 w1566 w1611 w1636 w1660 w1685 w1710 w1735 w1773 w1794 w1825 w1846 w1865 w1884 w1903 w1938 w1984 w2009 w2038 w2059 w2078 w2097 w2116 w2146 w2197 w2214 w2248 w2286 w2313 w2334 w2361 w2386 w2405 w2432 w2457 w2476 w2497 w2540 w2566 w2590 w2611 w2639 w2653 w2674 w2695 w2716 w2738 w2758 w2787 w2807 w2834 w2854 w2879 w2898 w2917 w2936 w2955 w2974 w2993]
            tunnel: w997 -> [w1083 w1102 w1121 w1140 w1202 w1275 w1322 w1374 w1406 w1450 w1505 w1520 w1545 w1565 w1610 w1635 w1659 w1684 w1709 w1734 w1772 w1793 w1824 w1845 w1864 w1883 w1902 w1937 w1983 w2008 w2037 w2058 w2077 w2096 w2115 w2145 w2196 w2213 w2247 w2283 w2312 w2333 w2360 w2385 w2404 w2431 w2456 w2475 w2496 w2539 w2565 w2589 w2610 w2638 w2652 w2673 w2694 w2715 w2737 w2757 w2786 w2806 w2833 w2853 w2878 w2897 w2916 w2935 w2954 w2973 w2992]
            tunnel: [w1084 w1103 w1122 w1141 w1203 w1276 w1323 w1375 w1407 w1451 w1506 w1521 w1546 w1566 w1611 w1636 w1660 w1685 w1710 w1735 w1773 w1794 w1825 w1846 w1865 w1884 w1903 w1938 w1984 w2009 w2038 w2059 w2078 w2097 w2116 w2146 w2197 w2214 w2248 w2285 w2313 w2334 w2361 w2386 w2405 w2432 w2457 w2476 w2497 w2540 w2566 w2590 w2611 w2639 w2653 w2674 w2695 w2716 w2738 w2758 w2787 w2807 w2834 w2854 w2879 w2898 w2917 w2936 w2955 w2974 w2993] -> w996
            tunnel: [w1083 w1102 w1121 w1140 w1202 w1275 w1322 w1374 w1406 w1450 w1505 w1520 w1545 w1565 w1610 w1635 w1659 w1684 w1709 w1734 w1772 w1793 w1824 w1845 w1864 w1883 w1902 w1937 w1983 w2008 w2037 w2058 w2077 w2096 w2115 w2145 w2196 w2213 w2247 w2284 w2312 w2333 w2360 w2385 w2404 w2431 w2456 w2475 w2496 w2539 w2565 w2589 w2610 w2638 w2652 w2673 w2694 w2715 w2737 w2757 w2786 w2806 w2833 w2853 w2878 w2897 w2916 w2935 w2954 w2973 w2992] -> w995
            tunnel: w994 -> [_ _ _ _ _ _ _ _ _ _ w1497 _ _ _ w1622 _ _ _ _ _ _ _ _ _ _ _ _ _ w1980 _ _ _ _ _ _ w2143 w2195 _ _ _ _ _ _ _ _ _ _ _ _ _ _ _ _ _ _ _ _ _ _ _ _ _ _ _ _ _ _ _ _ _ _]
            tunnel: w993 -> [_ _ _ _ _ _ _ _ _ _ w1498 _ _ _ w1621 _ _ _ _ _ _ _ _ _ _ _ _ _ w1979 _ _ _ _ _ _ w2144 w2194 _ _ _ _ _ _ _ _ _ _ _ _ _ _ _ _ _ _ _ _ _ _ _ _ _ _ _ _ _ _ _ _ _ _]
            tunnel: w990 -> [_ _ _ _ _ _ _ _ _ _ _ _ _ _ _ _ w1651 _ w1696 w1725 w1761 w1787 w1820 _ _ _ _ w1921 w1966 w2004 w2033 _ _ _ _ _ _ _ _ _ _ _ _ _ _ _ _ _ _ _ _ _ _ _ _ _ _ _ _ _ _ _ _ _ _ _ _ _ _ _ _]
            tunnel: [_ _ _ _ _ _ _ _ _ _ _ _ _ _ _ _ _ _ _ w1729 w1763 w1790 w1823 _ _ _ _ TRUE w1969 w2006 _ _ _ _ _ _ _ _ _ _ _ _ _ _ _ _ _ _ _ _ _ _ _ _ _ _ _ _ _ _ _ _ _ _ _ _ _ _ _ _ _] -> w989
            tunnel: w988 -> [_ _ _ _ _ _ _ _ _ _ _ _ _ _ _ _ w1650 _ _ w1728 w1767 w1792 w1821 _ _ _ _ w1929 w1974 w2003 w2036 _ _ _ _ _ _ _ _ _ _ _ _ _ _ _ _ _ _ _ _ _ _ _ _ _ _ _ _ _ _ _ _ _ _ _ _ _ _ _ _]
            tunnel: w987 -> [_ _ _ _ _ _ _ _ _ _ _ _ _ _ _ _ w1649 _ _ w1727 w1766 w1791 w1822 _ _ _ _ w1928 w1973 w2002 w2035 _ _ _ _ _ _ _ _ _ _ _ _ _ _ _ _ _ _ _ _ _ _ _ _ _ _ _ _ _ _ _ _ _ _ _ _ _ _ _ _]
            tunnel: [_ _ _ _ _ _ _ _ _ _ _ _ _ _ _ _ w1650 _ w1699 w1728 w1767 w1792 w1821 _ _ _ _ w1929 w1974 w2003 w2036 _ _ _ _ _ _ _ _ _ _ _ _ _ _ _ _ _ _ _ _ _ _ _ _ _ _ _ _ _ _ _ _ _ _ _ _ _ _ _ _] -> w986
            tunnel: [_ _ _ _ _ _ _ _ _ _ _ _ _ _ _ _ w1649 _ w1698 w1727 w1766 w1791 w1822 _ _ _ _ w1928 w1973 w2002 w2035 _ _ _ _ _ _ _ _ _ _ _ _ _ _ _ _ _ _ _ _ _ _ _ _ _ _ _ _ _ _ _ _ _ _ _ _ _ _ _ _] -> w985
            tunnel: [_ _ _ _ _ _ _ _ _ _ _ _ _ _ _ _ w1652 w1678 w1697 w1726 w1762 w1788 w1819 _ _ _ _ w1922 w1967 w2005 w2034 _ _ _ _ _ _ _ _ _ _ _ _ _ _ _ _ _ _ _ _ _ _ _ _ _ _ _ _ _ _ _ _ _ _ _ _ _ _ _ _] -> w984
            tunnel: [_ _ _ _ _ _ _ _ _ _ _ _ _ _ _ _ w1651 w1679 w1696 w1725 w1761 w1787 w1820 _ _ _ _ w1921 w1966 w2004 w2033 _ _ _ _ _ _ _ _ _ _ _ _ _ _ _ _ _ _ _ _ _ _ _ _ _ _ _ _ _ _ _ _ _ _ _ _ _ _ _ _] -> w983
            tunnel: [_ _ _ _ _ _ _ _ _ _ _ _ _ _ _ _ _ _ _ _ w1760 _ _ _ _ _ _ _ w1971 _ _ _ _ _ _ _ _ _ _ _ _ _ _ _ _ _ _ _ _ _ _ _ _ _ _ _ _ _ _ _ _ _ _ _ _ _ _ _ _ _ _] -> w980
            tunnel: [_ _ _ _ _ _ _ _ _ _ _ _ _ _ _ _ _ _ _ _ w1759 _ _ _ _ _ _ _ w1972 _ _ _ _ _ _ _ _ _ _ _ _ _ _ _ _ _ _ _ _ _ _ _ _ _ _ _ _ _ _ _ _ _ _ _ _ _ _ _ _ _ _] -> w982
            tunnel: w977 -> [_ _ _ _ _ _ _ _ _ _ _ _ _ _ _ _ _ _ _ w1724 w1758 w1789 w1818 _ _ _ _ w1924 w1968 w2007 _ _ _ _ _ _ _ _ _ _ _ _ _ _ _ _ _ _ _ _ _ _ _ _ _ _ _ _ _ _ _ _ _ _ _ _ _ _ _ _ _]
            tunnel: [_ _ _ _ _ _ _ _ _ _ _ _ _ _ _ _ _ _ _ w1724 w1758 w1789 w1818 _ _ _ _ w1924 w1970 w2007 _ _ _ _ _ _ _ _ _ _ _ _ _ _ _ _ _ _ _ _ _ _ _ _ _ _ _ _ _ _ _ _ _ _ _ _ _ _ _ _ _] -> w976
            frame "Start1", Default {
            }
            frame "Start2" {
            }
            frame "Start3" {
            }
            frame "saveSettings1" {
              n547 = call "myRIO_BRig_RT_dataExp_Audio_freq__L.vi"() -> ("output_Audio_freq__L"=w1169:i32)  [unwired: 11 in]
              n548 = call "myRIO_BRig_RT_dataExp_Audio_freq__R.vi"() -> ("output_Audio_freq__R"=w1166:i32)  [unwired: 11 in]
              n549 = call "myRIO_BRig_RT_dataExp_Audio_amp__L.vi"() -> ("output_Audio_amp__L"=w1163:i32)  [unwired: 11 in]
              n550 = call "myRIO_BRig_RT_dataExp_Audio_amp__R.vi"() -> ("output_Audio_amp__R"=w1161:i32)  [unwired: 11 in]
              n551 = call "myRIO_BRig_RT_dataExp_TPB_min__L.vi"() -> ("output_TPB_min__L"=w1179:i32)  [unwired: 11 in]
              n552 = call "myRIO_BRig_RT_dataExp_TPB_min__R.vi"() -> ("output_TPB_min__R"=w1177:i32)  [unwired: 11 in]
              n553 = call "myRIO_BRig_RT_dataExp_TPB_max__L.vi"() -> ("output_TPB_max__L"=w1175:i32)  [unwired: 11 in]
              n554 = call "myRIO_BRig_RT_dataExp_TPB_max__R.vi"() -> ("output_TPB_max__R"=w1173:i32)  [unwired: 11 in]
              n555 = call "myRIO_BRig_RT_dataExp_ItrialUntilReward.vi"() -> ("output_I_trialUntilReward"=w1192:i32)  [unwired: 11 in]
              n556 = call "myRIO_BRig_RT_dataExp_IblockUntilReward.vi"() -> ("output_I_blockUntilReward"=w1188:i32)  [unwired: 11 in]
              n557 = call "myRIO_BRig_RT_dataExp_CueCycles.vi"() -> ("output_CueCycles"=w1187:i32)  [unwired: 11 in]
              n558 = call "myRIO_BRig_RT_dataExp_ENL_min.vi"() -> ("output_ENL_min"=w1185:i32)  [unwired: 11 in]
              n559 = call "myRIO_BRig_RT_dataExp_ENL_max.vi"() -> ("output_ENL_max"=w1183:i32)  [unwired: 11 in]
              n560 = call "myRIO_BRig_RT_dataExp_ENL_penalty.vi"() -> ("output_ENL_penalty"=w1181:i32)  [unwired: 11 in]
              n561 = local read "Audio_Freq__L"() -> (w1170:u16)
              n562 = local read "Audio_Freq__R"() -> (w1165:u16)
              n563 = local read "Audio_Amp__L"() -> (w1162:u16)
              n564 = local read "TpB_Min_L"() -> (w1178:u16)
              n565 = local read "TpB_Min_R"() -> (w1176:u16)
              n566 = local read "TpB_Max_L"() -> (w1174:u16)
              n567 = local read "TpB_Max_R"() -> (w1172:u16)
              n568 = local read "Audio_Amp__R"() -> (w1160:u16)
              n569 = local read "TrialUntilReward"() -> (w1191:bool)
              n570 = local read "CueCycles"() -> (w1186:u16)
              n571 = local read "Tcycle_ENL_min"() -> (w1184:u16)
              n572 = local read "Tcycle_ENL_max"() -> (w1182:u16)
              n573 = local read "Tcycle_ENLPenalty"() -> (w1180:u16)
              n574 = Multiply(x=w1170, y=u16 1000) -> (x*y=w1168:u16)
              n575 = Multiply(x=w1165, y=u16 1000) -> (x*y=w1164:u16)
              n576 = Boolean To (0,1)(Boolean=w1191) -> (0, 1=w1190:i16)
              n577 = To Unsigned Word Integer(number=w1190) -> (unsigned 16bit integer=w1189:u16)
              n578 = local read "BUR_min"() -> (w1154:u16)
              n579 = local read "BUR_max"() -> (w1155:u16)
              n580 = Not Equal To 0?(x=w1154) -> (x != 0?=w1153:bool)
              n581 = Not Equal To 0?(x=w1155) -> (x != 0?=w1152:bool)
              n582 = And(x=w1153, y=w1152) -> (x .and. y?=w1151:bool)
              n583 = Boolean To (0,1)(Boolean=w1151) -> (0, 1=w1156:i16)
              n584 = To Unsigned Word Integer(number=w1156) -> (unsigned 16bit integer=w1150:u16)
              n585 = Replace Array Subset(array=w1194, new element #1=w1189, index #1=w1192, new element #2=w1150, index #2=w1188, new element #3=w1186, index #3=w1187, new element #4=w1184, index #4=w1185, new element #5=w1182, index #5=w1183, new element #6=w1180, index #6=w1181, new element #7=w1178, index #7=w1179, new element #8=w1176, index #8=w1177, new element #9=w1174, index #9=w1175, new element #10=w1172, index #10=w1173, new element #11=w1168, index #11=w1169, new element #12=w1164, index #12=w1166, new element #13=w1162, index #13=w1163, new element #14=w1160, index #14=w1161) -> (w1193:u16[])
            }
            frame "saveSettings2" {
              n586 = call "myRIO_BRig_RT_dataExp_Tcycle_RewardPost.vi"() -> ("output_Tcycle_RewardPost"=w1227:i32)  [unwired: 11 in]
              n587 = call "myRIO_BRig_RT_dataExp_Tcycle_Wrong.vi"() -> ("output_Tcycle_Wrong"=w1225:i32)  [unwired: 11 in]
              n588 = call "myRIO_BRig_RT_dataExp_Tcycle_Timeout.vi"() -> ("output_Tcycle_Timeout"=w1223:i32)  [unwired: 11 in]
              n589 = call "myRIO_BRig_RT_dataExp_Tcycle_Cue_min.vi"() -> ("output_Tcycle_Cue_min"=w1221:i32)  [unwired: 11 in]
              n590 = call "myRIO_BRig_RT_dataExp_Tcycle_Cue_max.vi"() -> ("output_Tcycle_Cue_max"=w1220:i32)  [unwired: 11 in]
              n591 = call "myRIO_BRig_RT_dataExp_Tcycle_CuePenalty.vi"() -> ("output_Tcycle_CuePenalty"=w1219:i32)  [unwired: 11 in]
              n592 = call "myRIO_BRig_RT_dataExp_nBlock.vi"() -> ("output_nBlock"=w1236:i32)  [unwired: 11 in]
              n593 = call "myRIO_BRig_RT_dataExp_nTrial.vi"() -> ("output_nTrial"=w1235:i32)  [unwired: 11 in]
              n594 = call "myRIO_BRig_RT_dataExp_runTime_seconds.vi"() -> ("output_RunTime_minutes"=w1234:i32)  [unwired: 11 in]
              n595 = call "myRIO_BRig_RT_dataExp_Tcycle_Selection.vi"() -> ("output_Tcycle_Selection"=w1233:i32)  [unwired: 11 in]
              n596 = call "myRIO_BRig_RT_dataExp_Tcycle_Reward__L.vi"() -> ("output_Tcycle_Reward__L"=w1231:i32)  [unwired: 11 in]
              n597 = call "myRIO_BRig_RT_dataExp_Tcycle_Reward__R.vi"() -> ("output_Tcycle_Reward__R"=w1229:i32)  [unwired: 11 in]
              n598 = local read "Tcycle_RewardPost"() -> (w1226:u16)
              n599 = local read "Tcycle_Wrong"() -> (w1224:u16)
              n600 = local read "Tcycle_Timeout"() -> (w1222:u16)
              n601 = local read "Tcycle_CuePenalty"() -> (w1212:u16)
              n602 = local read "Tcycle_Cue_max"() -> (w1200:u16)
              n603 = local read "Tcycle_Cue_min"() -> (w1201:u16)
              n604 = local read "Tcycle_Selection"() -> (w1232:u16)
              n605 = local read "Tcycle_Reward_L"() -> (w1230:u16)
              n606 = local read "Tcycle_Reward_R"() -> (w1228:u16)
              n607 = Replace Array Subset(array=w1238, new element #1=u16 0, index #1=w1236, new element #2=u16 0, index #2=w1235, new element #3=u16 0, index #3=w1234, new element #4=w1232, index #4=w1233, new element #5=w1230, index #5=w1231, new element #6=w1228, index #6=w1229, new element #7=w1226, index #7=w1227, new element #8=w1224, index #8=w1225, new element #9=w1222, index #9=w1223, new element #10=w1201, index #10=w1221, new element #11=w1200, index #11=w1220, new element #12=w1212, index #12=w1219) -> (w1237:u16[])
            }
            frame "saveSettings3" {
              w1247 = 100.0 ("y")
              n608 = call "myRIO_BRig_RT_dataExp_laser_Freq.vi"() -> ("output_laser_Freq"=w1271:i32)  [unwired: 11 in]
              n609 = call "myRIO_BRig_RT_dataExp_laser_Tpeak.vi"() -> ("output_laser_Tpeak"=w1266:i32)  [unwired: 11 in]
              n610 = call "myRIO_BRig_RT_dataExp_laser_Tshutter.vi"() -> ("output_laser_Tshutter"=w1261:i32)  [unwired: 11 in]
              n611 = call "myRIO_BRig_RT_dataExp_laser_f_millisec2count.vi"() -> ("output_laser_f_millisec2count"=w1256:i32)  [unwired: 11 in]
              n612 = call "myRIO_BRig_RT_dataExp_laser_Power.vi"() -> ("output_laser_Power"=w1251:i32)  [unwired: 11 in]
              n613 = call "myRIO_BRig_RT_dataExp_laser_duration.vi"() -> ("output_laser_duration"=w1245:i32)  [unwired: 11 in]
              n614 = call "myRIO_BRig_RT_dataExp_BUR_min.vi"() -> ("output_BUR_min"=w1293:i32)  [unwired: 11 in]
              n615 = call "myRIO_BRig_RT_dataExp_BUR_max.vi"() -> ("output_BUR_max"=w1291:i32)  [unwired: 11 in]
              n616 = call "myRIO_BRig_RT_dataExp_Audio_sp__L.vi"() -> ("output_Audio_sp__L"=w1288:i32)  [unwired: 11 in]
              n617 = call "myRIO_BRig_RT_dataExp_Audio_sp__R.vi"() -> ("output_Audio_sp__R"=w1287:i32)  [unwired: 11 in]
              n618 = local read "laser_Tshutter"() -> (w1258:dbl)
              n619 = local read "f_millisec2count"() -> (w1253:dbl)
              n620 = local read "laser_power"() -> (w1248:dbl)
              n621 = local read "laser_Tpeak"() -> (w1263:dbl)
              n622 = local read "laser_Freq"() -> (w1270:dbl)
              n623 = local read "sp_LeftSpout"() -> (w1286:u16)
              n624 = local read "BUR_max"() -> (w1290:u16)
              n625 = local read "sp_RightSpout"() -> (w1285:u16)
              n626 = local read "BUR_min"() -> (w1292:u16)
              n627 = Multiply(x=w1263, y=w1247) -> (x*y=w1265:dbl)
              n628 = Multiply(x=w1258, y=w1247) -> (x*y=w1260:dbl)
              n629 = Multiply(x=w1253, y=w1247) -> (x*y=w1255:dbl)
              n630 = Multiply(x=w1248, y=w1247) -> (x*y=w1250:dbl)
              n631 = Multiply(x=w1270, y=w1247) -> (x*y=w1269:dbl)
              n632 = Round To Nearest(number=w1265) -> (nearest integer value=w1264:dbl)
              n633 = Round To Nearest(number=w1260) -> (nearest integer value=w1259:dbl)
              n634 = Round To Nearest(number=w1255) -> (nearest integer value=w1254:dbl)
              n635 = Round To Nearest(number=w1250) -> (nearest integer value=w1249:dbl)
              n636 = Round To Nearest(number=w1269) -> (nearest integer value=w1268:dbl)
              n637 = To Unsigned Word Integer(number=w1264) -> (unsigned 16bit integer=w1262:u16)
              n638 = To Unsigned Word Integer(number=w1259) -> (unsigned 16bit integer=w1257:u16)
              n639 = To Unsigned Word Integer(number=w1254) -> (unsigned 16bit integer=w1252:u16)
              n640 = To Unsigned Word Integer(number=w1249) -> (unsigned 16bit integer=w1246:u16)
              n641 = To Unsigned Word Integer(number=w1268) -> (unsigned 16bit integer=w1267:u16)
              n642 = local read "laser_duration"() -> (w1244:u16)
              n643 = call "myRIO_BRig_RT_dataCurrent_LaserPulse_duration.vi"() -> ("output_LaserPulse_duration"=w1272:i32)  [unwired: 11 in]
              n644 = Replace Array Subset(array=w1294, new element #1=w1292, index #1=w1293, new element #2=w1290, index #2=w1291, new element #3=w1286, index #3=w1288, new element #4=w1285, index #4=w1287, new element #5=w1267, index #5=w1271, new element #6=w1262, index #6=w1266, new element #7=w1257, index #7=w1261, new element #8=w1252, index #8=w1256, new element #9=w1246, index #9=w1251, new element #10=w1244, index #10=w1245) -> (w1289:u16[])
              n645 = Replace Array Subset(array=w1274, new element=w1244, index=w1272) -> (w1273:u16[])
            }
            frame "saveSettings4_LC_ENL" {
              # "delayOpt"
              # "Count"
              # "Tdelay"
              # "Probability"
              # "OnOff"
              # "Block"
              # "ENL1 All"
              # "delayOpt"
              # "Count"
              # "Tdelay"
              # "Probability"
              # "OnOff"
              # "Block"
              # "ENL1 First"
              n646 = call "myRIO_BRig_RT_dataLC_ENL1_All_Block.vi"() -> ("output_ENL1_All_Block"=w1317:i32)  [unwired: 11 in]
              n647 = call "myRIO_BRig_RT_dataLC_ENL1_All_OnOff.vi"() -> ("output_ENL1_All_OnOff"=w1306:i32)  [unwired: 11 in]
              n648 = call "myRIO_BRig_RT_dataLC_ENL1_All_Probability.vi"() -> ("output_ENL1_All_Probability"=w1305:i32)  [unwired: 11 in]
              n649 = call "myRIO_BRig_RT_dataLC_ENL1_All_Tdelay.vi"() -> ("output_ENL1_All_Tdelay"=w1304:i32)  [unwired: 11 in]
              n650 = call "myRIO_BRig_RT_dataLC_ENL1_All_Count.vi"() -> ("output_ENL1_All_Count"=w1303:i32)  [unwired: 11 in]
              n651 = call "myRIO_BRig_RT_dataLC_ENL1_All_delayOpt.vi"() -> ("output_ENL1_All_delayOpt"=w1302:i32)  [unwired: 11 in]
              n652 = call "myRIO_BRig_RT_dataLC_ENL1_First_Block.vi"() -> ("output_ENL1_First_Block"=w1343:i32)  [unwired: 11 in]
              n653 = call "myRIO_BRig_RT_dataLC_ENL1_First_OnOff.vi"() -> ("output_ENL1_First_OnOff"=w1341:i32)  [unwired: 11 in]
              n654 = call "myRIO_BRig_RT_dataLC_ENL1_First_Probability.vi"() -> ("output_ENL1_First_Probability"=w1337:i32)  [unwired: 11 in]
              n655 = call "myRIO_BRig_RT_dataLC_ENL1_First_Tdelay.vi"() -> ("output_ENL1_First_Tdelay"=w1335:i32)  [unwired: 11 in]
              n656 = call "myRIO_BRig_RT_dataLC_ENL1_First_Count.vi"() -> ("output_ENL1_First_Count"=w1333:i32)  [unwired: 11 in]
              n657 = call "myRIO_BRig_RT_dataLC_ENL1_First_delayOpt.vi"() -> ("output_ENL1_First_delayOpt"=w1319:i32)  [unwired: 11 in]
              n658 = local read "LC_ENL1_First_delayOpt"() -> (w1320:bool)
              n659 = local read "LC_ENL1_First_Count"() -> (w1332:u16)
              n660 = local read "LC_ENL1_First_Probability"() -> (w1336:u16)
              n661 = local read "LC_ENL1_First_Block"() -> (w1342:u16)
              n662 = local read "LC_ENL1_First_Tdelay"() -> (w1334:u16)
              n663 = local read "LC_ENL1_First_OnOff"() -> (w1340:bool)
              n664 = local read "LC_ENL1_All_OnOff"() -> (w1313:bool)
              n665 = local read "LC_ENL1_All_Probability"() -> (w1311:u16)
              n666 = local read "LC_ENL1_All_delayOpt"() -> (w1308:bool)
              n667 = local read "LC_ENL1_All_Tdelay"() -> (w1310:u16)
              n668 = local read "LC_ENL1_All_Block"() -> (w1314:u16)
              n669 = local read "LC_ENL1_All_Count"() -> (w1309:u16)
              n670 = Boolean To (0,1)(Boolean=w1320) -> (0, 1=w1321:i16)
              n671 = Boolean To (0,1)(Boolean=w1340) -> (0, 1=w1339:i16)
              n672 = Boolean To (0,1)(Boolean=w1313) -> (0, 1=w1316:i16)
              n673 = To Unsigned Word Integer(number=w1321) -> (unsigned 16bit integer=w1318:u16)
              n674 = To Unsigned Word Integer(number=w1339) -> (unsigned 16bit integer=w1338:u16)
              n675 = Boolean To (0,1)(Boolean=w1308) -> (0, 1=w1315:i16)
              n676 = To Unsigned Word Integer(number=w1316) -> (unsigned 16bit integer=w1312:u16)
              n677 = To Unsigned Word Integer(number=w1315) -> (unsigned 16bit integer=w1307:u16)
              n678 = Replace Array Subset(array=w1344, new element #1=w1342, index #1=w1343, new element #2=w1338, index #2=w1341, new element #3=w1336, index #3=w1337, new element #4=w1334, index #4=w1335, new element #5=w1332, index #5=w1333, new element #6=w1318, index #6=w1319, new element #7=w1314, index #7=w1317, new element #8=w1312, index #8=w1306, new element #9=w1311, index #9=w1305, new element #10=w1310, index #10=w1304, new element #11=w1309, index #11=w1303, new element #12=w1307, index #12=w1302) -> (w1345:u16[])
            }
            frame "saveSettings5_LC_Cue" {
              # "delayOpt"
              # "Count"
              # "Tdelay"
              # "Probability"
              # "OnOff"
              # "Block"
              # "Cue1 All"
              # "delayOpt"
              # "Count"
              # "Tdelay"
              # "Probability"
              # "OnOff"
              # "Block"
              # "Cue1 First"
              n679 = call "myRIO_BRig_RT_dataLC_Cue1_First_delayOpt.vi"() -> ("output_Cue1_First_delayOpt"=w1372:i32)  [unwired: 11 in]
              n680 = call "myRIO_BRig_RT_dataLC_Cue1_First_Block.vi"() -> ("output_Cue1_First_Block"=w1395:i32)  [unwired: 11 in]
              n681 = call "myRIO_BRig_RT_dataLC_Cue1_First_OnOff.vi"() -> ("output_Cue1_First_OnOff"=w1393:i32)  [unwired: 11 in]
              n682 = call "myRIO_BRig_RT_dataLC_Cue1_First_Probability.vi"() -> ("output_Cue1_First_Probability"=w1389:i32)  [unwired: 11 in]
              n683 = call "myRIO_BRig_RT_dataLC_Cue1_First_Tdelay.vi"() -> ("output_Cue1_First_Tdelay"=w1387:i32)  [unwired: 11 in]
              n684 = call "myRIO_BRig_RT_dataLC_Cue1_First_Count.vi"() -> ("output_Cue1_First_Count"=w1385:i32)  [unwired: 11 in]
              n685 = call "myRIO_BRig_RT_dataLC_Cue1_All_Block.vi"() -> ("output_Cue1_All_Block"=w1369:i32)  [unwired: 11 in]
              n686 = call "myRIO_BRig_RT_dataLC_Cue1_All_OnOff.vi"() -> ("output_Cue1_All_OnOff"=w1368:i32)  [unwired: 11 in]
              n687 = call "myRIO_BRig_RT_dataLC_Cue1_All_Probability.vi"() -> ("output_Cue1_All_Probability"=w1367:i32)  [unwired: 11 in]
              n688 = call "myRIO_BRig_RT_dataLC_Cue1_All_Tdelay.vi"() -> ("output_Cue1_All_Tdelay"=w1366:i32)  [unwired: 11 in]
              n689 = call "myRIO_BRig_RT_dataLC_Cue1_All_Count.vi"() -> ("output_Cue1_All_Count"=w1365:i32)  [unwired: 11 in]
              n690 = call "myRIO_BRig_RT_dataLC_Cue1_All_delayOpt.vi"() -> ("output_Cue1_All_delayOpt"=w1364:i32)  [unwired: 11 in]
              n691 = local read "LC_Cue1_First_delayOpt"() -> (w1371:bool)
              n692 = local read "LC_Cue1_First_Count"() -> (w1384:u16)
              n693 = local read "LC_Cue1_First_Probability"() -> (w1388:u16)
              n694 = local read "LC_Cue1_First_Block"() -> (w1394:u16)
              n695 = local read "LC_Cue1_First_Tdelay"() -> (w1386:u16)
              n696 = local read "LC_Cue1_First_OnOff"() -> (w1392:bool)
              n697 = local read "LC_Cue1_All_OnOff"() -> (w1360:bool)
              n698 = local read "LC_Cue1_All_delayOpt"() -> (w1361:bool)
              n699 = local read "LC_Cue1_All_Probability"() -> (w1357:u16)
              n700 = local read "LC_Cue1_All_Tdelay"() -> (w1356:u16)
              n701 = local read "LC_Cue1_All_Count"() -> (w1355:u16)
              n702 = local read "LC_Cue1_All_Block"() -> (w1359:u16)
              n703 = Boolean To (0,1)(Boolean=w1371) -> (0, 1=w1373:i16)
              n704 = Boolean To (0,1)(Boolean=w1392) -> (0, 1=w1391:i16)
              n705 = Boolean To (0,1)(Boolean=w1360) -> (0, 1=w1363:i16)
              n706 = To Unsigned Word Integer(number=w1373) -> (unsigned 16bit integer=w1370:u16)
              n707 = To Unsigned Word Integer(number=w1391) -> (unsigned 16bit integer=w1390:u16)
              n708 = To Unsigned Word Integer(number=w1363) -> (unsigned 16bit integer=w1358:u16)
              n709 = Boolean To (0,1)(Boolean=w1361) -> (0, 1=w1362:i16)
              n710 = To Unsigned Word Integer(number=w1362) -> (unsigned 16bit integer=w1354:u16)
              n711 = Replace Array Subset(array=w1396, new element #1=w1394, index #1=w1395, new element #2=w1390, index #2=w1393, new element #3=w1388, index #3=w1389, new element #4=w1386, index #4=w1387, new element #5=w1384, index #5=w1385, new element #6=w1370, index #6=w1372, new element #7=w1359, index #7=w1369, new element #8=w1358, index #8=w1368, new element #9=w1357, index #9=w1367, new element #10=w1356, index #10=w1366, new element #11=w1355, index #11=w1365, new element #12=w1354, index #12=w1364) -> (w1397:u16[])
            }
            frame "saveSettings6_LC_Other" {
              # "Trial"
              # "Tdelay"
              # "Probability"
              # "OnOff"
              # "Block"
              # "Wrong"
              # "Trial"
              # "Tdelay"
              # "Probability"
              # "OnOff"
              # "Block"
              # "Reward"
              n712 = call "myRIO_BRig_RT_dataLC_Wrong_Block.vi"() -> ("output_Wrong_Block"=w1427:i32)  [unwired: 11 in]
              n713 = call "myRIO_BRig_RT_dataLC_Wrong_OnOff.vi"() -> ("output_Wrong_OnOff"=w1426:i32)  [unwired: 11 in]
              n714 = call "myRIO_BRig_RT_dataLC_Wrong_Probability.vi"() -> ("output_Wrong_Probability"=w1425:i32)  [unwired: 11 in]
              n715 = call "myRIO_BRig_RT_dataLC_Wrong_Tdelay.vi"() -> ("output_Wrong_Tdelay"=w1424:i32)  [unwired: 11 in]
              n716 = call "myRIO_BRig_RT_dataLC_Wrong_Trial.vi"() -> ("output_Wrong_Trial"=w1423:i32)  [unwired: 11 in]
              n717 = call "myRIO_BRig_RT_dataLC_Reward_Block.vi"() -> ("output_Reward_Block"=w1439:i32)  [unwired: 11 in]
              n718 = call "myRIO_BRig_RT_dataLC_Reward_OnOff.vi"() -> ("output_Reward_OnOff"=w1437:i32)  [unwired: 11 in]
              n719 = call "myRIO_BRig_RT_dataLC_Reward_Probability.vi"() -> ("output_Reward_Probability"=w1433:i32)  [unwired: 11 in]
              n720 = call "myRIO_BRig_RT_dataLC_Reward_Tdelay.vi"() -> ("output_Reward_Tdelay"=w1431:i32)  [unwired: 11 in]
              n721 = call "myRIO_BRig_RT_dataLC_Reward_Trial.vi"() -> ("output_Reward_Trial"=w1429:i32)  [unwired: 11 in]
              n722 = local read "LC_Wrong_OnOff"() -> (w1421:bool)
              n723 = local read "LC_Wrong_Probability"() -> (w1418:u16)
              n724 = local read "LC_Wrong_Block"() -> (w1420:u16)
              n725 = local read "LC_Wrong_Tdelay"() -> (w1417:u16)
              n726 = local read "LC_Wrong_Trial"() -> (w1416:u16)
              n727 = local read "LC_Reward_Probability"() -> (w1432:u16)
              n728 = local read "LC_Reward_Block"() -> (w1438:u16)
              n729 = local read "LC_Reward_Tdelay"() -> (w1430:u16)
              n730 = local read "LC_Reward_OnOff"() -> (w1436:bool)
              n731 = local read "LC_Reward_Trial"() -> (w1428:u16)
              n732 = Boolean To (0,1)(Boolean=w1421) -> (0, 1=w1422:i16)
              n733 = Boolean To (0,1)(Boolean=w1436) -> (0, 1=w1435:i16)
              n734 = To Unsigned Word Integer(number=w1422) -> (unsigned 16bit integer=w1419:u16)
              n735 = To Unsigned Word Integer(number=w1435) -> (unsigned 16bit integer=w1434:u16)
              n736 = Replace Array Subset(array=w1440, new element #1=w1438, index #1=w1439, new element #2=w1434, index #2=w1437, new element #3=w1432, index #3=w1433, new element #4=w1430, index #4=w1431, new element #5=w1428, index #5=w1429, new element #6=w1420, index #6=w1427, new element #7=w1419, index #7=w1426, new element #8=w1418, index #8=w1425, new element #9=w1417, index #9=w1424, new element #10=w1416, index #10=w1423) -> (w1441:u16[])
            }
            frame "setSettings_Audio" {
              # "amp_L"
              # "amp_R"
              # "freq_L"
              # "freq_R"
              n737 = call "myRIO_BRig_RT_dataExp_Audio_amp__L.vi"() -> ("output_Audio_amp__L"=w1464:i32)  [unwired: 11 in]
              n738 = call "myRIO_BRig_RT_dataExp_Audio_amp__R.vi"() -> ("output_Audio_amp__R"=w1463:i32)  [unwired: 11 in]
              n739 = call "myRIO_BRig_RT_dataExp_Audio_freq__L.vi"() -> ("output_Audio_freq__L"=w1462:i32)  [unwired: 11 in]
              n740 = call "myRIO_BRig_RT_dataExp_Audio_freq__R.vi"() -> ("output_Audio_freq__R"=w1461:i32)  [unwired: 11 in]
              n741 = Index Array(array=w1460, index #1=w1464, index #2=w1463, index #3=w1462, index #4=w1461) -> (element #1=w1459:u16, element #2=w1457:u16, element #3=w1458:u16, element #4=w1456:u16)
            }
            frame "setSettings_Laser" {
              n742 = call "myRIO_Brig_RT__covert_Voltage_to_FPGAvalue.vi"("input_voltage"="laser_power") -> ("output_PortA"=w1473:u16)  [unwired: 9 in, 1 out]
              n743 = call "myRIO_BRig_RT__calc_Tvalley.vi"("input_peakWidth"="laser_Tpeak", "input_freq"="laser_Freq") -> ("output_Tvalley"=w1480:dbl)  [unwired: 9 in]
              n744 = Multiply(x="f_millisec2count", y="laser_Tpeak") -> (x*y=w1490:dbl)
              n745 = Multiply(x="f_millisec2count", y=w1480) -> (x*y=w1487:dbl)
              n746 = Multiply(x="f_millisec2count", y="laser_Tshutter") -> (x*y=w1485:dbl)
              n747 = Round Toward +Infinity(x="laser_Tshutter") -> (ceil(x): smallest int >= x=w1474:dbl)
              n748 = Round Toward +Infinity(x="f_millisec2count") -> (ceil(x): smallest int >= x=w1493:dbl)
              n749 = Round Toward +Infinity(x=w1490) -> (ceil(x): smallest int >= x=w1491:dbl)
              n750 = Round Toward +Infinity(x=w1487) -> (ceil(x): smallest int >= x=w1488:dbl)
              n751 = Round Toward +Infinity(x=w1485) -> (ceil(x): smallest int >= x=w1479:dbl)
              n752 = To Unsigned Long Integer(number=w1493) -> (unsigned 32bit integer=w1492:u32)
              n753 = To Unsigned Long Integer(number=w1491) -> (unsigned 32bit integer=w1489:u32)
              n754 = To Unsigned Long Integer(number=w1488) -> (unsigned 32bit integer=w1486:u32)
              n755 = To Unsigned Long Integer(number=w1479) -> (unsigned 32bit integer=w1483:u32)
              n756 = To Unsigned Word Integer(number=w1474) -> (unsigned 16bit integer=w1478:u16)
              n757 = xnode "Read/Write Control"("FPGA VI Reference In"=w1497, "error in"=w1498, "laser_Npeak"=w1489, "laser_Nvalley"=w1486, "f_time_select"=w1492, "AnaOut_0"=w1473, "laser_Nshutter"=w1483) -> ("error out"=→"error out":errorcluster)  [unwired: 1 out]
              n758 = Add(x="laser_duration", y=w1478) -> (x+y=w1476:u16)
              n759 = call "myRIO_BRig_RT_dataCurrent_LaserPulse_duration.vi"() -> ("output_LaserPulse_duration"=w1494:i32)  [unwired: 11 in]
              n760 = Replace Array Subset(array=w1496, new element=w1476, index=w1494) -> (w1495:u16[])
            }
            frame "initBlock" {
              n761 = call "myRIO_Brig_RT__Case_Exp_State_initBlock.vi"("input_spout"=w1542, "input_dataExp"=w1540, "input_dataCurrent"=w1541) -> ("output_spout"=w1519:enum16{"Left", "Right"}, "output_state"=w1543:T2, "output_dataExp"=w1539:u16[], "output_dataCurrent"=w1525:u16[], "output_TpB_target"=→"TpB_target":u16)  [unwired: 4 in]
              "cSpout" <- w1519
              n762 = call "myRIO_BRig_RT_dataCurrent_iBlock.vi"() -> ("output_iBlock"=w1524:i32)  [unwired: 11 in]
              n763 = Index Array(array=w1525, index=w1524) -> (element=→"iBlock":u16)
            }
            frame "initBlock2" {
              n764 = local write "nRewards_cur"(u16 0 ("nRewards_cur")) -> ()
              n765 = call "myRIO_BRig_RT__Case_Exp_State_initBlock2.vi"("input_spout"=w1551, "input_dataBlock"=w1552, "input_dataCurrent"=w1550) -> ("idxDataBlock"=w1547:i32, "output_dataBlock"=w1549:u16[][])  [unwired: 7 in]
            }
            frame "initTrial" {
              n766 = call "myRIO_Brig_RT__Case_Exp_State_initTrial.vi"("input_dataExp"=w1581, "input_dataCurrent"=w1582) -> ("output_state"=w1583:T2, "output_dataExp"=w1580:u16[], "output_dataCurrent"=w1570:u16[])  [unwired: 7 in]
              n767 = call "myRIO_BRig_RT_dataCurrent_iTrial.vi"() -> ("output_iTrial"=w1569:i32)  [unwired: 11 in]
              n768 = Index Array(array=w1570, index=w1569) -> (element=→"iTrial":u16)
            }
            frame "initTrial2" {
              w1588 = u32 10
              # "laser time"
              # "Wrong tDelay"
              # "Reward tDelay"
              # "trialUntilReward"
              n769 = call "myRIO_BRig_RT__Case_Exp_subState_LC__initTrial.vi"("input_dataTrial"=w1598, "input_spout"=w1607, "input_dataCurrent"=w1596, "input_dataLC"=w1593) -> ("output_LC_Wrong"=w1608:bool, "output_LC_led_Wrong"=w1600:bool, "output_LC_Reward"=w1609:bool, "output_LC_led_Reward"=w1599:bool, "output_dataTrial"=w1597:u16[][])  [unwired: 2 in]
              n770 = Equal?(x=w1607, y=enum16{"Left", "Right"}."Right") -> (x = y?=w1605:bool)
              n771 = call "myRIO_BRig_RT_dataExp_ItrialUntilReward.vi"() -> ("output_I_trialUntilReward"=w1603:i32)  [unwired: 11 in]
              n772 = Index Array(array=w1604, index=w1603) -> (element=w1602:u16)
              n773 = call "myRIO_BRig_RT_dataLC_Reward_Tdelay.vi"() -> ("output_Reward_Tdelay"=w1594:i32)  [unwired: 11 in]
              n774 = call "myRIO_BRig_RT_dataLC_Wrong_Tdelay.vi"() -> ("output_Wrong_Tdelay"=w1595:i32)  [unwired: 11 in]
              n775 = Not Equal To 0?(x=w1602) -> (x != 0?=w1601:bool)
              n776 = Index Array(array=w1593, index #1=w1594, index #2=w1595) -> (element #1=w1592:u16, element #2=w1591:u16)
              n777 = To Unsigned Long Integer(number=w1592) -> (unsigned 32bit integer=w1590:u32)
              n778 = To Unsigned Long Integer(number=w1591) -> (unsigned 32bit integer=w1589:u32)
              n779 = xnode "Read/Write Control"("FPGA VI Reference In"=w1622, "error in"=w1621, "SelectionState"=FALSE, "laserResponse_reward"=w1609, "laserResponse_wrong"=w1608, "laserResponse_reward_LED"=w1599, "laserResponse_wrong_LED"=w1600, "Left(F)_or_Right(T)"=w1605, "ignoreWrong"=w1601, "tCycle_laser_rew"=w1588, "tDelay_laser_rew"=w1590, "tCycle_laser_wro"=w1588, "tDelay_laser_wro"=w1589) -> ("error out"=→"error_initTrial":errorcluster)  [unwired: 1 out]
            }
            frame "initTrial3" {
              n780 = call "myRIO_BRig_RT__Case_Exp_State_initTrial_dataTrial.vi"("input_spout"=w1629, "input_dataCurrent"=w1630, "input_dataTrial"=w1632) -> ("output_dataTrial"=w1631:u16[][])  [unwired: 8 in]
            }
            frame "initTrial4" {
            }
            frame "initTrial_LC_ENL1" {
              n781 = call "myRIO_BRig_RT__Case_Exp_State_initTrial_LC_ENL1__v2.vi"("input_dataTrial"=w1675, "input_spout"=w1680, "input_dataBlock"=w1673, "input_dataLC"=w1681, "input_dataCurrent"=w1677) -> ("output_LC__ENL1"=w1679:bool, "output_LC_led__ENL1"=w1678:bool, "output_dataTrial"=w1674:u16[][], "output_dataCurrent"=w1676:u16[])  [unwired: 3 in]
            }
            frame "initTrial_LC_Cue1" {
              n782 = call "myRIO_BRig_RT__Case_Exp_State_initTrial_LC_Cue1__v2.vi"("input_dataTrial"=w1702, "input_spout"=w1705, "input_dataBlock"=w1700, "input_dataLC"=w1706, "input_dataCurrent"=w1704) -> ("output_LC__Cue1"=w1698:bool, "output_LC_led__Cue1"=w1699:bool, "output_dataTrial"=w1701:u16[][], "output_dataCurrent"=w1703:u16[])  [unwired: 3 in]
            }
            frame "ENL1_pre" {
              # "ENL1_n"
              # "Tcycle"
              # "counter"
              n783 = call "myRIO_BRig_RT_dataCurrent_Tcycle_generic.vi"() -> ("output_Tcycle_generic"=w1752:i32)  [unwired: 11 in]
              n784 = call "myRIO_BRig_RT_dataCurrent_count_generic.vi"() -> ("output_count_generic"=w1754:i32)  [unwired: 11 in]
              n785 = call "myRIO_BRig_RT_dataCurrent_ENL.vi"() -> ("output_ENL"=w1751:i32)  [unwired: 11 in]
              n786 = call "myRIO_BRig_RT_dataCurrent_ENL1_n.vi"() -> ("output_ENL1_n"=w1723:i32)  [unwired: 11 in]
              n787 = Index Array(array=w1745, index #1=w1751, index #2=w1723) -> (element #1=w1750:u16, element #2=w1722:u16)
              n788 = Increment(x=w1722) -> (x+1=w1721:u16)
              n789 = Replace Array Subset(array=w1745, new element #1=u16 0 ("new element/subarray"), index #1=w1754, new element #2=w1750, index #2=w1752, new element #3=w1721, index #3=w1723) -> (w1749:u16[])
              n790 = Select(t=myRIO_BRig_RT__Case_Exp_stateList."ENL1Penalty_pre" ("Enum"), s=w1733, f=myRIO_BRig_RT__Case_Exp_stateList."ENL1" ("Enum")) -> (s? t:f=w1730:T2)
            }
            frame "ENL1" {
              n791 = call "myRIO_BRig_RT__Case_Exp_State_ENL1__v2.vi"("input_LC"=w1761, "I_lick"=w1765, "input_LC_led"=w1762, "input_laserOccurred"=w1757, "input_state"=w1771, "input_dataCurrent"=w1770) -> ("output_trigger_laser_led"=w1760:bool, "output_state"=w1768:T2, "output_dataCurrent"=w1769:u16[], "output_trigger_laser"=w1759:bool)  [unwired: 2 in]
              n792 = Or(x=w1760, y=w1757) -> (x .or. y?=w1763:bool)
            }
            frame "ENL1Penalty_pre" {
              # "Tcycle"
              # "counter"
              n793 = call "myRIO_BRig_RT_dataCurrent_Tcycle_generic.vi"() -> ("output_Tcycle_generic"=w1811:i32)  [unwired: 11 in]
              n794 = call "myRIO_BRig_RT_dataCurrent_count_generic.vi"() -> ("output_count_generic"=w1813:i32)  [unwired: 11 in]
              n795 = call "myRIO_BRig_RT_dataExp_ENL_penalty.vi"() -> ("output_ENL_penalty"=w1806:i32)  [unwired: 11 in]
              n796 = Index Array(array=w1807, index=w1806) -> (element=w1810:u16)
              n797 = Replace Array Subset(array=w1808, new element #1=u16 0 ("new element/subarray"), index #1=w1813, new element #2=w1810, index #2=w1811) -> (w1809:u16[])
            }
            frame "ENL1Penalty" {
              n798 = call "myRIO_BRig_RT__Case_Exp_State_ENL1Penalty.vi"("input_state"=w1836, "input_dataCurrent"=w1840) -> ("output_state"=w1837:T2, "output_dataCurrent"=w1839:u16[])  [unwired: 8 in]
            }
            frame "ENL2_pre" {
            }
            frame "ENL2" {
            }
            frame "ENL2Penalty_pre" {
            }
            frame "ENL2Penalty" {
            }
            frame "Cue1_pre" {
              # "Cue1_n"
              # "Tcycle_Cue1"
              # "0 = L, 1 = R, 2 = both"
              # "sp_R"
              # "sp_L"
              # "Tcycle"
              # "counter"
              n799 = Equal?(x=w1951, y=enum16{"Left", "Right"}."Left") -> (x = y?=w1950:bool)
              n800 = call "myRIO_BRig_RT_dataExp_Audio_sp__L.vi"() -> ("output_Audio_sp__L"=w1949:i32)  [unwired: 11 in]
              n801 = call "myRIO_BRig_RT_dataExp_Audio_sp__R.vi"() -> ("output_Audio_sp__R"=w1948:i32)  [unwired: 11 in]
              n802 = call "myRIO_BRig_RT_dataCurrent_Tcycle_generic.vi"() -> ("output_Tcycle_generic"=w1961:i32)  [unwired: 11 in]
              n803 = call "myRIO_BRig_RT_dataCurrent_count_generic.vi"() -> ("output_count_generic"=w1963:i32)  [unwired: 11 in]
              n804 = Select(t=w1949, s=w1950, f=w1948) -> (s? t:f=w1947:i32)
              n805 = call "myRIO_BRig_RT_dataCurrent_Cue1_n.vi"() -> ("output_Cue1_n"=w1925:i32)  [unwired: 11 in]
              n806 = call "myRIO_BRig_RT_dataCurrent_Tcycle_cue.vi"() -> ("output_Tcycle_cue"=w1934:i32)  [unwired: 11 in]
              n807 = Index Array(array=w1953, index=w1947) -> (element=w1945:u16)
              n808 = Index Array(array=w1935, index #1=w1934, index #2=w1925) -> (element #1=w1936:u16, element #2=w1927:u16)
              n809 = Increment(x=w1927) -> (x+1=w1926:u16)
              n810 = Not Equal To 0?(x=w1945) -> (x != 0?=w1943:bool)
              n811 = Not Equal?(x=w1945, y=u16 1) -> (x != y?=w1944:bool)
              n812 = Replace Array Subset(array=w1935, new element #1=u16 0 ("new element/subarray"), index #1=w1963, new element #2=w1936, index #2=w1961, new element #3=w1926, index #3=w1925) -> (w1960:u16[])
              n813 = Select(t=myRIO_BRig_RT__Case_Exp_stateList."Cue1Penalty_pre" ("Enum"), s=w1931, f=myRIO_BRig_RT__Case_Exp_stateList."Cue1" ("Enum")) -> (s? t:f=w1932:T2)
            }
            frame "Cue1" {
              n814 = call "myRIO_BRig_RT__Case_Exp_State_Cue1__v2.vi"("input_LC"=w1973, "I_lick"=w1976, "input_LC_led"=w1974, "input_laserOccurred"=w1968, "input_state"=w1978, "input_dataCurrent"=w1996) -> ("output_trigger_laser_led"=w1971:bool, "output_state"=w1977:T2, "output_dataCurrent"=w1995:u16[], "output_trigger_laser"=w1972:bool)  [unwired: 2 in]
              n815 = Or(x=w1971, y=w1968) -> (x .or. y?=w1970:bool)
              n816 = Equal?(x=myRIO_BRig_RT__Case_Exp_stateList."Selection_pre", y=w1977) -> (x = y?=w1981:bool)
              n817 = xnode "Read/Write Control"("FPGA VI Reference In"=w1980, "error in"=w1979, "SelectionState"=w1981) -> ()  [unwired: 2 out]
            }
            frame "Cue1Penalty_pre" {
              # "Tcycle"
              # "counter"
              n818 = call "myRIO_BRig_RT_dataCurrent_Tcycle_generic.vi"() -> ("output_Tcycle_generic"=w2027:i32)  [unwired: 11 in]
              n819 = call "myRIO_BRig_RT_dataCurrent_count_generic.vi"() -> ("output_count_generic"=w2029:i32)  [unwired: 11 in]
              n820 = call "myRIO_BRig_RT_dataExp_Tcycle_CuePenalty.vi"() -> ("output_Tcycle_CuePenalty"=w2026:i32)  [unwired: 11 in]
              n821 = Index Array(array=w2021, index=w2026) -> (element=w2025:u16)
              n822 = Replace Array Subset(array=w2023, new element #1=u16 0 ("new element/subarray"), index #1=w2029, new element #2=w2025, index #2=w2027) -> (w2022:u16[])
            }
            frame "Cue1Penalty" {
              # "reset laserOccurred"
              n823 = call "myRIO_BRig_RT__Case_Exp_State_Cue1Penalty.vi"("input_state"=w2053, "input_dataCurrent"=w2054) -> ("output_state"=w2051:T2, "output_dataCurrent"=w2052:u16[])  [unwired: 8 in]
            }
            frame "Cue2_pre" {
              n824 = call "myRIO_BRig_RT__Case_Exp_subState_LC__Cue2.vi"("input_spout"=w2071, "input_dataCurrent"=w2072, "input_dataLC"=w2070) -> ()  [unwired: 6 in, 2 out]
            }
            frame "Cue2" {
            }
            frame "Cue2Penalty_pre" {
            }
            frame "Cue2Penalty" {
            }
            frame "Selection_pre" {
              # "Tcycle"
              # "counter"
              n825 = xnode "Read/Write Control"("FPGA VI Reference In"=w2143, "error in"=w2144) -> ("error out"=→"error_Selection_pre":errorcluster, "SelectReward"=w2136:bool, "SelectWrong"=w2138:bool)  [unwired: 1 out]
              n826 = call "myRIO_BRig_RT_dataCurrent_Tcycle_generic.vi"() -> ("output_Tcycle_generic"=w2165:i32)  [unwired: 11 in]
              n827 = call "myRIO_BRig_RT_dataCurrent_count_generic.vi"() -> ("output_count_generic"=w2167:i32)  [unwired: 11 in]
              n828 = call "myRIO_BRig_RT_dataExp_Tcycle_Selection.vi"() -> ("output_Tcycle_Selection"=w2164:i32)  [unwired: 11 in]
              n829 = Index Array(array=w2161, index=w2164) -> (element=w2163:u16)
              n830 = Replace Array Subset(array=w2159, new element #1=u16 0 ("new element/subarray"), index #1=w2167, new element #2=w2163, index #2=w2165) -> (w2162:u16[])
              n831 = Or(x=w2136, y=w2138) -> (x .or. y?=w2137:bool)
              n832 = Select(t=myRIO_BRig_RT__Case_Exp_stateList."SelectReward_pre" ("Enum"), s=w2136, f=myRIO_BRig_RT__Case_Exp_stateList."SelectWrong_pre" ("Enum")) -> (s? t:f=w2142:T2)
              n833 = Select(t=w2142, s=w2137, f=myRIO_BRig_RT__Case_Exp_stateList."Selection" ("Enum")) -> (s? t:f=w2139:T2)
            }
            frame "Selection" {
              # "counter\nSelection"
              # "increment"
              # "get Tcycle"
              # "get count"
              n834 = xnode "Read/Write Control"("FPGA VI Reference In"=w2195, "error in"=w2194) -> ("FPGA VI Reference Out"=w2170:refnum<k20>, "error out"=w2171:errorcluster, "SelectReward"=w2191:bool, "SelectWrong"=w2192:bool)
              n835 = call "myRIO_BRig_RT_dataCurrent_Tcycle_generic.vi"() -> ("output_Tcycle_generic"=w2188:i32)  [unwired: 11 in]
              n836 = call "myRIO_BRig_RT_dataCurrent_count_generic.vi"() -> ("output_count_generic"=w2180:i32)  [unwired: 11 in]
              n837 = Index Array(array=w2189, index #1=w2188, index #2=w2180) -> (element #1=w2179:u16, element #2=w2187:u16)
              n838 = call "myRIO_BRig_RT__increment_u16.vi"() -> ("output_increment__u16"=w2186:u16)  [unwired: 11 in]
              n839 = Add(x=w2187, y=w2186) -> (x+y=w2181:u16)
              n840 = Greater?(x=w2179, y=w2181) -> (0:w2182:bool)
              n841 = Select(t=w2185, s=w2182, f=myRIO_BRig_RT__Case_Exp_stateList."SelectTimeout_pre" ("Enum")) -> (s? t:f=w2174:T2)
              n842 = Select(t=w2181, s=w2182, f=w2179) -> (s? t:f=w2177:u16)
              n843 = call "myRIO_BRig_RT_dataCurrent_count_selection.vi"() -> ("output_count_generic"=w2178:i32)  [unwired: 11 in]
              n844 = Select(t=myRIO_BRig_RT__Case_Exp_stateList."SelectReward_pre" ("Enum"), s=w2191, f=myRIO_BRig_RT__Case_Exp_stateList."SelectWrong_pre" ("Enum")) -> (s? t:f=w2190:T2)
              n845 = Replace Array Subset(array=w2189, new element #1=w2177, index #1=w2180, new element #2=w2177, index #2=w2178) -> (w2184:u16[])
              n846 = Or(x=w2191, y=w2192) -> (x .or. y?=w2173:bool)
              n847 = Not(x=w2173) -> (.not. x?=w2172:bool)
              n848 = xnode "Read/Write Control"("FPGA VI Reference In"=w2170, "error in"=w2171, "SelectionState"=w2172) -> ("error out"=→"error_Selection":errorcluster)  [unwired: 1 out]
              n849 = Select(t=w2190, s=w2173, f=w2174) -> (s? t:f=w2193:T2)
            }
            frame "SelectReward_pre" {
              # "iState"
              # "Tcycle\nReward"
              # "nRewTrials"
              # "Tcycle\nGeneric"
              # "counter"
              n850 = call "myRIO_BRig_RT_dataCurrent_nRewTrials.vi"() -> ("output_nRewTrials"=w2227:i32)  [unwired: 11 in]
              n851 = Equal?(x=w2236, y=enum16{"Left", "Right"}."Left") -> (x = y?=w2237:bool)
              n852 = Index Array(array=w2228, index=w2227) -> (element=w2226:u16)
              n853 = call "myRIO_BRig_RT_dataExp_Tcycle_Reward__L.vi"() -> ("output_Tcycle_Reward__L"=w2240:i32)  [unwired: 11 in]
              n854 = call "myRIO_BRig_RT_dataExp_Tcycle_Reward__R.vi"() -> ("output_Tcycle_Reward__R"=w2241:i32)  [unwired: 11 in]
              n855 = Increment(x=w2226) -> (x+1=w2225:u16)
              n856 = Select(t=w2240, s=w2237, f=w2241) -> (s? t:f=w2239:i32)
              n857 = call "myRIO_BRig_RT__Case_Exp_subState_LC__Reward.vi"("input_spout"=w2236, "input_dataCurrent"=w2228, "input_dataLC"=w2235) -> ()  [unwired: 6 in, 2 out]
              n858 = call "myRIO_BRig_RT_dataCurrent_count_generic.vi"() -> ("output_count_generic"=w2230:i32)  [unwired: 11 in]
              n859 = call "myRIO_BRig_RT_dataCurrent_Tcycle_generic.vi"() -> ("output_Tcycle_generic"=w2231:i32)  [unwired: 11 in]
              n860 = Index Array(array=w2242, index=w2239) -> (element=w2232:u16)
              n861 = call "myRIO_BRig_RT_dataCurrent_iState.vi"() -> ("output_iState"=w2220:i32)  [unwired: 11 in]
              n862 = Replace Array Subset(array=w2228, new element #1=w2225, index #1=w2227, new element #2=u16 0 ("new element/subarray"), index #2=w2230, new element #3=w2232, index #3=w2231, new element #4=u16 1 ("new element/subarray"), index #4=w2220) -> (w2243:u16[])
            }
            frame "SelectReward" {
              n863 = call "myRIO_BRig_RT__Case_Exp_State_Reward.vi"("input_dataCurrent"=w2265, "input_state"=w2262, "input_spout"=w2259, "input_LC"=w2260, "input_dataLC"=w2261) -> ("output_dataCurrent"=w2264:u16[], "output_state"=w2263:T2, "output__L"=w2257:bool, "output__R"=w2258:bool)  [unwired: 6 in, 1 out]
            }
            frame "SelectRewardPost_pre" {
              # "nRewards"
              # "nRewTrials"
              # "Tcycle"
              # "counter"
              n864 = call "myRIO_BRig_RT_dataBlock_nRewards__L.vi"() -> ("output_nRewards__L"=w2281:i32)  [unwired: 11 in]
              n865 = call "myRIO_BRig_RT_dataBlock_nRewards__R.vi"() -> ("output_nRewards__R"=w2280:i32)  [unwired: 11 in]
              n866 = call "myRIO_BRig_RT_dataCurrent_Tcycle_generic.vi"() -> ("output_Tcycle_generic"=w2300:i32)  [unwired: 11 in]
              n867 = call "myRIO_BRig_RT_dataCurrent_count_generic.vi"() -> ("output_count_generic"=w2302:i32)  [unwired: 11 in]
              n868 = case shown="\"Left\", Default" w2274 {
                tunnel: w2286 -> [w2307 w2311]
                tunnel: [w2306 w2311] -> w2285
                tunnel: [w2308 w2309] -> w2284
                tunnel: w2283 -> [w2308 w2310]
                frame "Left", Default {
                  n869 = Increment(x=w2307) -> (x+1=w2306:u16)
                }
                frame "Right" {
                  n870 = Increment(x=w2310) -> (x+1=w2309:u16)
                }
              }
              "nRewards_Left" <- w2285
              "nRewards_Right" <- w2284
              n871 = Equal?(x=w2274, y=enum16{"Left", "Right"}."Left") -> (x = y?=w2273:bool)
              n872 = Select(t=w2281, s=w2273, f=w2280) -> (s? t:f=w2279:i32)
              n873 = call "myRIO_BRig_RT_dataExp_Tcycle_RewardPost.vi"() -> ("output_Tcycle_RewardPost"=w2296:i32)  [unwired: 11 in]
              n874 = call "myRIO_BRig_RT_dataCurrent_nRewTrials.vi"() -> ("output_nRewTrials"=w2282:i32)  [unwired: 11 in]
              n875 = Index Array(array=w2297, index=w2296) -> (element=w2299:u16)
              n876 = Index Array(array=w2276, index=w2282) -> (element=w2271:u16)
              n877 = Replace Array Subset(array=w2276, new element #1=u16 0 ("new element/subarray"), index #1=w2302, new element #2=w2299, index #2=w2300) -> (w2298:u16[])
              n878 = Replace Array Subset(array=w2278, new element=w2271, index (row)=w2272, index (col)=w2279) -> (w2277:u16[][])
              n879 = local write "nRewards_cur"(w2271) -> ()
            }
            frame "SelectRewardPost" {
              n880 = call "myRIO_BRig_RT__Case_Exp_State_RewardPost.vi"("input_state"=w2326, "input_dataCurrent"=w2329) -> ("output_state"=w2327:T2, "output_dataCurrent"=w2328:u16[])  [unwired: 8 in]
            }
            frame "SelectWrong_pre" {
              # "iState"
              # "Tcycle"
              # "counter"
              n881 = call "myRIO_BRig_RT_dataCurrent_Tcycle_generic.vi"() -> ("output_Tcycle_generic"=w2354:i32)  [unwired: 11 in]
              n882 = call "myRIO_BRig_RT_dataCurrent_count_generic.vi"() -> ("output_count_generic"=w2356:i32)  [unwired: 11 in]
              n883 = call "myRIO_BRig_RT_dataExp_Tcycle_Wrong.vi"() -> ("output_Tcycle_Wrong"=w2352:i32)  [unwired: 11 in]
              n884 = call "myRIO_BRig_RT__Case_Exp_subState_LC__Wrong.vi"("input_spout"=w2348, "input_dataCurrent"=w2349, "input_dataLC"=w2346) -> ()  [unwired: 6 in, 2 out]
              n885 = Index Array(array=w2350, index=w2352) -> (element=w2353:u16)
              n886 = call "myRIO_BRig_RT_dataCurrent_iState.vi"() -> ("output_iState"=w2340:i32)  [unwired: 11 in]
              n887 = Replace Array Subset(array=w2349, new element #1=u16 0 ("new element/subarray"), index #1=w2356, new element #2=w2353, index #2=w2354, new element #3=u16 2 ("new element/subarray"), index #3=w2340) -> (w2351:u16[])
            }
            frame "SelectWrong" {
              n888 = call "myRIO_BRig_RT__Case_Exp_State_Wrong.vi"("input_dataLC"=w2377, "input_LC"=w2376, "input_state"=w2370, "input_dataCurrent"=w2380) -> ("output_state"=w2367:T2, "output_dataCurrent"=w2379:u16[])  [unwired: 5 in, 1 out]
              n889 = Not Equal?(x=w2370, y=w2367) -> (x != y?=w2369:bool)
              n890 = Select(t=myRIO_BRig_RT__Case_Exp_stateList."SelectWrong_post" ("Enum"), s=w2369, f=w2367) -> (s? t:f=w2366:T2)
            }
            frame "SelectWrong_post" {
            }
            frame "SelectTimeout_pre" {
              # "iState"
              # "Tcycle"
              # "counter"
              n891 = call "myRIO_BRig_RT_dataCurrent_Tcycle_generic.vi"() -> ("output_Tcycle_generic"=w2425:i32)  [unwired: 11 in]
              n892 = call "myRIO_BRig_RT_dataCurrent_count_generic.vi"() -> ("output_count_generic"=w2423:i32)  [unwired: 11 in]
              n893 = call "myRIO_BRig_RT_dataExp_Tcycle_Timeout.vi"() -> ("output_Tcycle_Timeout"=w2427:i32)  [unwired: 11 in]
              n894 = call "myRIO_BRig_RT__Case_Exp_subState_LC__Timeout.vi"("input_spout"=w2418, "input_dataCurrent"=w2419, "input_dataLC"=w2417) -> ()  [unwired: 6 in, 2 out]
              n895 = Index Array(array=w2421, index=w2427) -> (element=w2426:u16)
              n896 = call "myRIO_BRig_RT_dataCurrent_iState.vi"() -> ("output_iState"=w2411:i32)  [unwired: 11 in]
              n897 = Replace Array Subset(array=w2419, new element #1=u16 0 ("new element/subarray"), index #1=w2423, new element #2=w2426, index #2=w2425, new element #3=u16 3 ("new element/subarray"), index #3=w2411) -> (w2422:u16[])
            }
            frame "SelectTimeout" {
              n898 = call "myRIO_BRig_RT__Case_Exp_State_Timeout.vi"("input_dataLC"=w2446, "input_LC"=w2447, "input_state"=w2437, "input_dataCurrent"=w2452) -> ("output_state"=w2438:T2, "output_dataCurrent"=w2451:u16[])  [unwired: 5 in, 1 out]
              n899 = Not Equal?(x=w2437, y=w2438) -> (x != y?=w2441:bool)
              n900 = Select(t=myRIO_BRig_RT__Case_Exp_stateList."SelectTimeout_post" ("Enum"), s=w2441, f=w2438) -> (s? t:f=w2439:T2)
            }
            frame "SelectTimeout_post" {
            }
            frame "endTrial1" {
              # "Update dataBlock"
              n901 = call "myRIO_BRig_RT__Case_Exp_State_endTrial1.vi"("input_spout"=w2485, "input_dataBlock"=w2484, "input_dataCurrent"=w2482) -> ("output_dataBlock"=w2483:u16[][], "output_dataCurrent"=w2481:u16[])  [unwired: 7 in]
            }
            frame "endTrial2" {
              # "update dataTrial"
              n902 = call "myRIO_BRig_RT__Case_Exp_State_endTrial2.vi"("input_spout"=w2504, "input_dataTrial"=w2508, "input_dataCurrent"=w2506) -> ("output_dataTrial"=w2507:u16[][], "output_dataCurrent"=w2505:u16[])  [unwired: 7 in]
            }
            frame "endTrial3" {
              w2530 = myRIO_BRig_RT__Case_Exp_stateList."endBlock" ("Enum")
              # "nRewTrials"
              # "iTrial"
              # "I_blockUntilReward"
              # "TPB"
              # "end block?"
              n903 = local read "STOP_endTrial"() -> (w2528:bool)
              n904 = local read "STOP_abort"() -> (w2527:bool)
              n905 = local read "START"() -> (w2525:bool)
              n906 = call "myRIO_BRig_RT_dataExp_IblockUntilReward.vi"() -> ("output_I_blockUntilReward"=w2537:i32)  [unwired: 11 in]
              n907 = Index Array(array=w2521, index=w2537) -> (element=w2517:u16)
              n908 = Not(x=w2525) -> (.not. x?=w2526:bool)
              n909 = Not Equal To 0?(x=w2517) -> (x != 0?=w2535:bool)
              n910 = Compound Arithmetic op=OR(w2528, w2526, w2527) -> (w2529:bool)
              n911 = call "myRIO_BRig_RT_dataCurrent_nRewTrials.vi"() -> ("output_nRewTrials"=w2533:i32)  [unwired: 11 in]
              n912 = call "myRIO_BRig_RT_dataCurrent_iTrial.vi"() -> ("output_iTrial"=w2534:i32)  [unwired: 11 in]
              n913 = Select(t=w2533, s=w2535, f=w2534) -> (s? t:f=w2532:i32)
              n914 = call "myRIO_BRig_RT_dataCurrent_TpB.vi"() -> ("output_TpB"=w2536:i32)  [unwired: 11 in]
              n915 = Index Array(array=w2522, index #1=w2536, index #2=w2532) -> (element #1=w2523:u16, element #2=w2524:u16)
              n916 = Less Or Equal?(x=w2523, y=w2524) -> (x <= y?=w2520:bool)
              n917 = Select(t=w2530, s=w2520, f=myRIO_BRig_RT__Case_Exp_stateList."empty_endTrial1" ("Enum")) -> (s? t:f=w2531:T2)
              n918 = Select(t=w2530, s=w2529, f=w2531) -> (s? t:f=w2518:T2)
            }
            frame "endBlock" {
              # "R"
              # "L"
              # "idxDataBlock"
              n919 = Equal?(x=w2561, y=enum16{"Left", "Right"}."Left") -> (x = y?=w2560:bool)
              n920 = call "myRIO_BRig_RT_dataCurrent_idxDataBlockL.vi"() -> ("output_idxDataBlock__L"=w2564:i32)  [unwired: 11 in]
              n921 = call "myRIO_BRig_RT_dataCurrent_idxDataBlockR.vi"() -> ("output_idxDataBlock__R"=w2563:i32)  [unwired: 11 in]
              n922 = Increment(x=w2555) -> (x+1=w2554:i32)
              n923 = Select(t=w2564, s=w2560, f=w2563) -> (s? t:f=w2558:i32)
              n924 = To Unsigned Word Integer(number=w2554) -> (unsigned 16bit integer=w2556:u16)
              n925 = local read "START"() -> (w2584:bool)
              n926 = local read "STOP_endBlock"() -> (w2579:bool)
              n927 = local read "STOP_endTrial"() -> (w2582:bool)
              n928 = local read "STOP_abort"() -> (w2581:bool)
              n929 = Replace Array Subset(array=w2559, new element=w2556, index=w2558) -> (w2557:u16[])
              n930 = Not(x=w2584) -> (.not. x?=w2583:bool)
              n931 = Compound Arithmetic op=OR(w2583, w2579, w2582, w2581) -> (w2580:bool)
              n932 = Select(t=myRIO_BRig_RT__Case_Exp_stateList."endExp" ("Enum"), s=w2580, f=myRIO_BRig_RT__Case_Exp_stateList."empty_endBlock1" ("Enum")) -> (s? t:f=w2588:T2)
            }
            frame "endExp" {
            }
            frame "commConnect" {
              n933 = call "myRIO_BRig_RT_comm_webdav_connect.vi"("input_password"="Host Password", "input_username"="Host UserName") -> ("output_Iconnected"=w2609:bool, "output_hSession"=w2627:T6)  [unwired: 7 in, 1 out]
              "Connected To Host?" <- w2609
              n934 = case shown="False" w2609 {
                frame False {
                  n935 = One Button Dialog(message="Connection Failed!\nData not being saved!") -> ()  [unwired: 1 in, 1 out]
                }
                frame True {
                }
              }
            }
            frame "commUpload_pre" {
              n936 = Select(t=myRIO_BRig_RT__Case_Exp_stateList."commUpload_dataBlock" ("Enum"), s=w2634, f=myRIO_BRig_RT__Case_Exp_stateList."endTrial3") -> (s? t:f=w2632:T2)
            }
            frame "commUpload_dataBlock" {
              n937 = call "myRIO_BRig_RT_comm_webdav_uploadFile__data.vi"("input_fileName_prefix"=w2655, "input_fileName"="dataBlock" ("input_filename"), "input_hSession"=w2657) -> ()  [unwired: 8 in, 1 out]
            }
            frame "commUpload_dataCurrent" {
              n938 = call "myRIO_BRig_RT_comm_webdav_uploadFile__data.vi"("input_fileName_prefix"=w2676, "input_fileName"="dataCurrent" ("input_filename"), "input_hSession"=w2678) -> ()  [unwired: 8 in, 1 out]
            }
            frame "commUpload_dataExp" {
              n939 = call "myRIO_BRig_RT_comm_webdav_uploadFile__data.vi"("input_fileName_prefix"=w2697, "input_fileName"="dataExp" ("input_filename"), "input_hSession"=w2699) -> ()  [unwired: 8 in, 1 out]
            }
            frame "commUpload_dataLC" {
              n940 = call "myRIO_BRig_RT_comm_webdav_uploadFile__data.vi"("input_fileName_prefix"=w2718, "input_fileName"="dataLC" ("input_filename"), "input_hSession"=w2720) -> ()  [unwired: 8 in, 1 out]
            }
            frame "commUpload_dataTrial" {
              n941 = call "myRIO_BRig_RT_comm_webdav_uploadFile__data.vi"("input_fileName_prefix"=w2742, "input_fileName"="dataTrial" ("input_filename"), "input_hSession"=w2744) -> ()  [unwired: 8 in, 1 out]
            }
            frame "saveData_dataBlock" {
              # "idxDataBlockR"
              # "idxDataBlockL"
              n942 = call "myRIO_BRig_RT_dataCurrent_idxDataBlockL.vi"() -> ("output_idxDataBlock__L"=w2768:i32)  [unwired: 11 in]
              n943 = call "myRIO_BRig_RT_dataCurrent_idxDataBlockR.vi"() -> ("output_idxDataBlock__R"=w2769:i32)  [unwired: 11 in]
              n944 = Index Array(array=w2770, index #1=w2768, index #2=w2769) -> (element #1=w2767:u16, element #2=w2766:u16)
              n945 = Greater?(x=w2767, y=w2766) -> (0:w2765:bool)
              n946 = Select(t=w2767, s=w2765, f=w2766) -> (s? t:f=w2763:u16)
              n947 = Increment(x=w2763) -> (x+1=w2762:u16)
              n948 = To Long Integer(number=w2762) -> (32bit integer=w2761:i32)
              n949 = Array Subset(array=w2764, length (row)=w2761) -> (w2760:u16[][])  [unwired: 3 in]
              n950 = call "myRIO_BRig_RT_comm_webdav_saveArrayToFile__2D_u16.vi"("Array"=w2760, "input_filename"="dataBlock") -> ()  [unwired: 10 in]
            }
            frame "saveData_dataCurrent" {
              n951 = call "myRIO_BRig_RT_comm_webdav_saveArrayToFile__1D_u16.vi"("Array"=w2789, "input_filename"="dataCurrent") -> ()  [unwired: 10 in]
            }
            frame "saveData_dataExp" {
              # "runTime"
              n952 = Get Date/Time In Seconds() -> (seconds since 1Jan1904=w2817:timestamp)
              n953 = To Double Precision Float(number=w2817) -> (double precision float=w2816:dbl)
              n954 = call "myRIO_BRig_RT_dataExp_runTime_seconds.vi"() -> ("output_RunTime_minutes"=w2815:i32)  [unwired: 11 in]
              n955 = Subtract(x=w2816, y=w2814) -> (x-y=w2811:dbl)
              n956 = To Unsigned Word Integer(number=w2811) -> (unsigned 16bit integer=w2810:u16)
              n957 = Replace Array Subset(array=w2809, new element=w2810, index=w2815) -> (w2812:u16[])
              n958 = call "myRIO_BRig_RT_comm_webdav_saveArrayToFile__1D_u16.vi"("Array"=w2812, "input_filename"="dataExp") -> ()  [unwired: 10 in]
            }
            frame "saveData_dataLC" {
              n959 = call "myRIO_BRig_RT_comm_webdav_saveArrayToFile__1D_u16.vi"("Array"=w2836, "input_filename"="dataLC") -> ()  [unwired: 10 in]
            }
            frame "saveData_dataTrial" {
              # "idxTrial"
              n960 = call "myRIO_BRig_RT_dataCurrent_idxDataTrial.vi"() -> ("output_idxDataTrial"=w2861:i32)  [unwired: 11 in]
              n961 = Index Array(array=w2862, index=w2861) -> (element=w2858:u16)
              n962 = Increment(x=w2858) -> (x+1=w2857:u16)
              n963 = To Long Integer(number=w2857) -> (32bit integer=w2856:i32)
              n964 = Array Subset(array=w2859, length (row)=w2856) -> (w2860:u16[][])  [unwired: 3 in]
              n965 = call "myRIO_BRig_RT_comm_webdav_saveArrayToFile__2D_u16.vi"("Array"=w2860, "input_filename"="dataTrial") -> ()  [unwired: 10 in]
            }
            frame "empty_endBlock1" {
            }
            frame "empty_endBlock2" {
            }
            frame "empty_endTrial1" {
            }
            frame "empty_endTrial2" {
            }
            frame "empty_endTrial3" {
            }
            frame "empty_endTrial4" {
            }
            frame "empty_endTrial5" {
            }
          }
          n966 = case shown="True" w1051 {
            tunnel: w1047 -> [w1074 w1082]
            tunnel: w1050 -> [_ w1078]
            tunnel: w1049 -> [_ w1077]
            tunnel: w1048 -> [_ w1076]
            tunnel: w1017 -> [_ w1075]
            tunnel: [w1074 w1081] -> w1046
            tunnel: w1045 -> [w1073 w1080]
            tunnel: [w1073 w1079] -> w1044
            frame False {
            }
            frame True {
              n967 = call "myRIO_BRig_RT__Case_Exp__recordLick.vi"("intput_state__trialEnd"=w1075, "intput_state__trialStart"=w1076, "input_lick__R"=w1077, "input_lick__L"=w1078, "input_dataCurrent"=w1080, "input_dataLick"=w1082) -> ("output_dataCurrent"=w1079:u16[], "output_dataLick"=w1081:u16[][])  [unwired: 4 in]
            }
          }
          n968 = Or(x=w1019, y=w1020) -> (x .or. y?=w1006:bool)
          n969 = Or(x=w1023, y=w1003) -> (x .or. y?=w992:bool)
          n970 = Or(x=w1002, y=w1024) -> (x .or. y?=w1018:bool)
          n971 = Or(x=w1022, y=w1021) -> (x .or. y?=w1007:bool)
          n972 = Or(x=w1052, y="STOP_abort") -> (x .or. y?=w1054:bool)
          n973 = Or(x=w980, y=w981) -> (x .or. y?=w978:bool)
          n974 = Or(x=w982, y=w981) -> (x .or. y?=w979:bool)
          n975 = xnode "Read/Write Control"("FPGA VI Reference In"=w994, "error in"=w993, "A1_SR"=w1007, "A3_SL"=w1006, "A6_Act"=w991, "audioTrigger_L"=w992, "audioAmp_L"=w1033, "audioFreq_L_Hz"=w1001, "audioTrigger_R"=w1018, "audioAmp_R"=w1034, "audioFreq_R_Hz"=w1035, "laserledMTrig"=w978, "laserMTrig"=w979) -> ("FPGA VI Reference Out"=w1043:refnum<k20>, "error out"=w1042:errorcluster)
          n976 = node-c288() -> ()  [unwired: 1 in, 1 out]
          "cState" <- w1048
        }
        n977 = node-c288(w938) -> ()  [unwired: 1 out]
        n978 = flat-sequence {
          tunnel: w934 -> [w970]
          tunnel: w933 -> [w969]
          tunnel: [w968] -> w926
          tunnel: [w967] -> w925
          tunnel: [w974] -> w927
          tunnel: [w975] -> w932
          tunnel: w926 -> [w975]
          tunnel: w925 -> [w974]
          frame #0 {
            w971 = u16 0 ("AudioLeft_phase_inc")
            w966 = FALSE
            n979 = xnode "Read/Write Control"("FPGA VI Reference In"=w970, "error in"=w969, "Counts_Reset"=TRUE, "audioTrigger_L"=w966, "audioFreq_L_Hz"=w971, "audioAmp_L"=w971, "audioTrigger_R"=w966, "audioFreq_R_Hz"=w971, "audioAmp_R"=w971, "A3_SL"=w966, "A1_SR"=w966, "A6_Act"=w966) -> ("FPGA VI Reference Out"=w968:refnum<k20>, "error out"=w967:errorcluster)
          }
          frame #1 {
            w973 = FALSE ("START")
            n980 = local write "START"(w973) -> ()
            n981 = local write "STOP_endTrial"(w973) -> ()
            n982 = local write "STOP_endBlock"(w973) -> ()
          }
        }
        n983 = stacked-sequence {
          tunnel: w910 -> [w946 _]
          tunnel: w908 -> [w947 _]
          tunnel: w907 -> [_ w952]
          tunnel: w906 -> [_ w951]
          tunnel: w905 -> [_ w950]
          tunnel: w904 -> [w940 _]
          frame #0 {
            n984 = call "myRIO_BRig_RT_dataCurrent_idxDataLick.vi"() -> ("output_idxDataLick"=w941:i32)  [unwired: 11 in]
            n985 = Index Array(array=w940, index=w941) -> (element=w943:u16)
            n986 = Increment(x=w943) -> (x+1=w944:u16)
            n987 = call "myRIO_BRig_RT_comm_webdav_saveArrayToFile__1D_u16.vi"("Array"=w947, "input_filename"="dataMTrig") -> ()  [unwired: 10 in]
            n988 = To Long Integer(number=w944) -> (32bit integer=w942:i32)
            n989 = Array Subset(array=w946, length (row)=w942) -> (w945:u16[][])  [unwired: 3 in]
            n990 = call "myRIO_BRig_RT_comm_webdav_saveArrayToFile__2D_u16.vi"("Array"=w945, "input_filename"="dataLick") -> ()  [unwired: 10 in]
          }
          frame #1 {
            n991 = case shown="True" w952 {
              tunnel: w951 -> [_ w954]
              tunnel: w950 -> [_ w953]
              frame False {
              }
              frame True {
                n992 = stacked-sequence {
                  tunnel: w954 -> [w956 w963 w965]
                  tunnel: w953 -> [w957 w962 _]
                  frame #0 {
                    n993 = call "myRIO_BRig_RT_comm_webdav_uploadFile__announce.vi"("input_addText"=TRUE, "input_fileName_prefix"=w957, "intput_fileName"="curExp_end", "intput_hSession"=w956) -> ("output_Isuccess"=w955:bool)  [unwired: 6 in, 1 out]
                    n994 = case shown="True" w955 {
                      frame False {
                        n995 = One Button Dialog(message="!!! Warning !!! Your data is located at C:\\BehaviorRig\\commTransfer") -> ()  [unwired: 1 in, 1 out]
                      }
                      frame True {
                        n996 = Wait (ms)(milliseconds to wait=u32 20) -> ()  [unwired: 1 out]
                      }
                    }
                  }
                  frame #1 {
                    n997 = call "myRIO_BRig_RT__endExp_sendData.vi"("input_fileName_prefix"=w962, "input_hSession"=w963) -> ()  [unwired: 8 in, 2 out]
                  }
                  frame #2 {
                    n998 = local write "Connected To Host?"(FALSE ("Connected To Host?")) -> ()
                    n999 = call <vilib>:"Close Session.vi"("session handle"=w965) -> ()  [unwired: 14 in, 1 out]
                  }
                }
              }
            }
          }
        }
      }
    }
    n1000 = local read "STOP_abort"() -> (w30:bool)
  }
  n1001 = xnode "Read/Write Control"("FPGA VI Reference In"=w8, "error in"=w7, "FPGA_Stop"=TRUE) -> ("FPGA VI Reference Out"=w13:refnum<k20>, "error out"=w14:errorcluster)
  n1002 = xnode "Close FPGA VI Reference"("FPGA VI Reference In"=w13, "error in"=w14) -> ("error out"=w12:errorcluster)
  n1003 = call <vilib>:"Reset myRIO.vi"("error in (no error)"=w12) -> ()  [unwired: 10 in, 1 out]
